vi "Variant_KVP to Strict Variant.vi"(6 "KVP":variant, 7 "use system decimal point (F)":bool, 8 "Strict type matching? (F)":bool, 9 "Default Value Name (empty: label)":string, 10 "Default Value":variant, 11 "Parent Name":string) -> (0 "all found?":bool, 1 "any found?":bool, 2 "Value":variant, 3 "name out":string)   [LabVIEW 2013, in "OpenVariant.lvlib"]
doc: "***********************\nDEPRECATED METHOD KEPT FOR BACKWARD COMPATIBILITY.\nUse the \"Variant_KVP to Strict variant (Standard).vi\" method instead for future development.\n***********************\nThis VI takes a default value as the input and replaces it recursively (cluster, array) with values found in key value pair arrays."
uses:
  TypeDescriptor/TypeDescriptor_GetPString.vi
  Variant_EmptyCluster.vi
  Scalar/FinalStringFormatting.vi
  TypeDescriptor/TypeDescriptor_SetName.vi
  <vilib>/Utility/GetType.llb/TD_Create Cluster.vi
  <vilib>/Utility/GetType.llb/TD_Get Array Information.vi
  <vilib>/Utility/GetType.llb/Get Type Code from I16 Array And Pos.vi
  Scalar/Get Decimal Separator.vi
  OpenVariant.lvlib
  TypeDescriptor/OpenDescriptor.lvlib
  Conversions/OpenConvert.lvlib
  Scalar/OpenScalar.lvlib
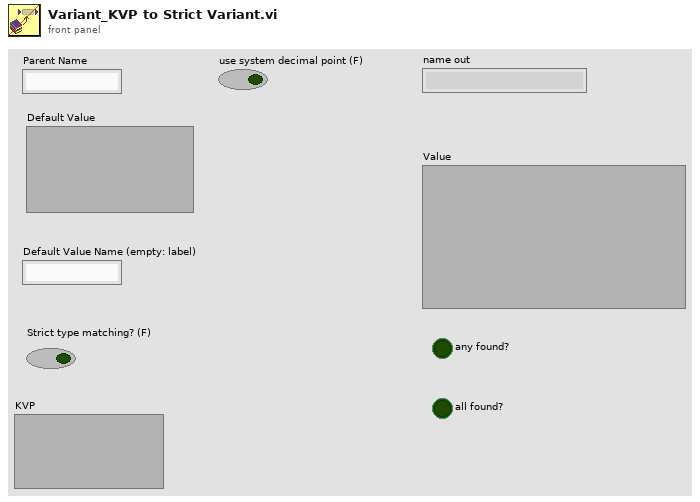
[diagram p1: front panel]
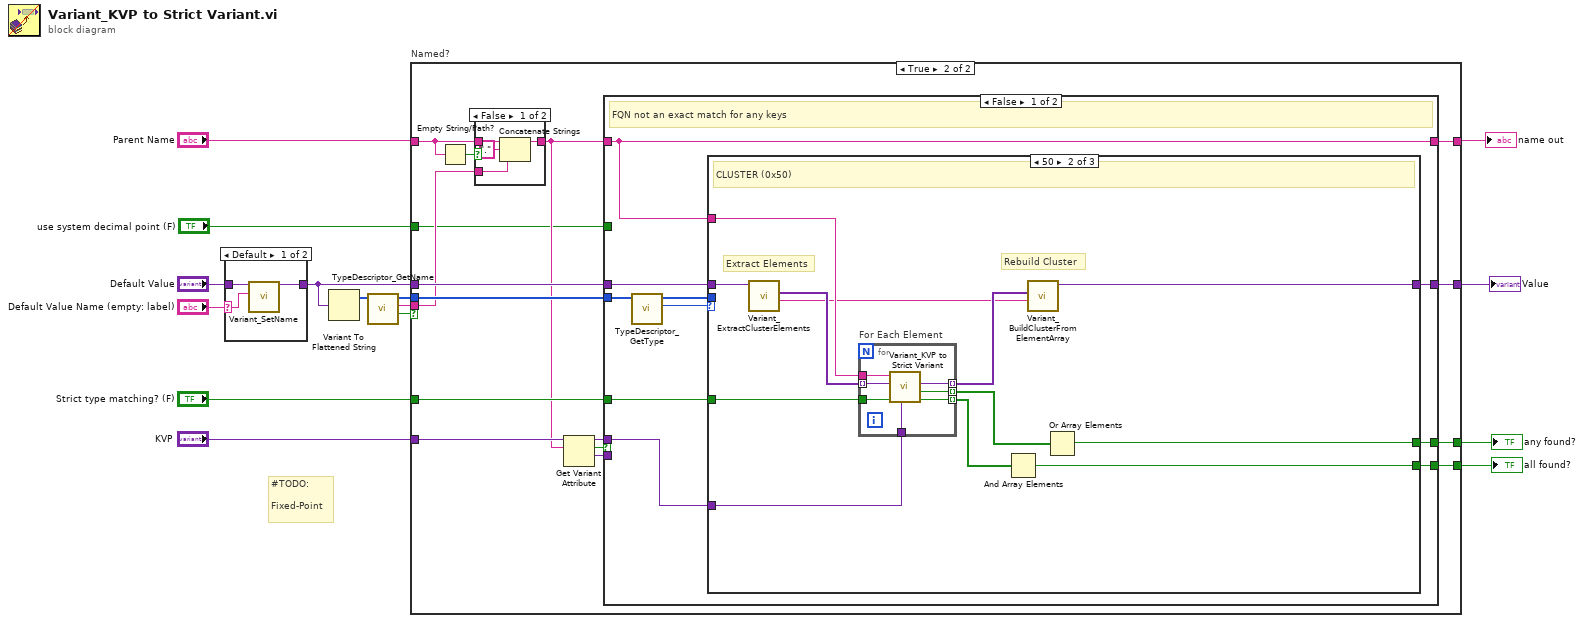
[diagram p0: block diagram]
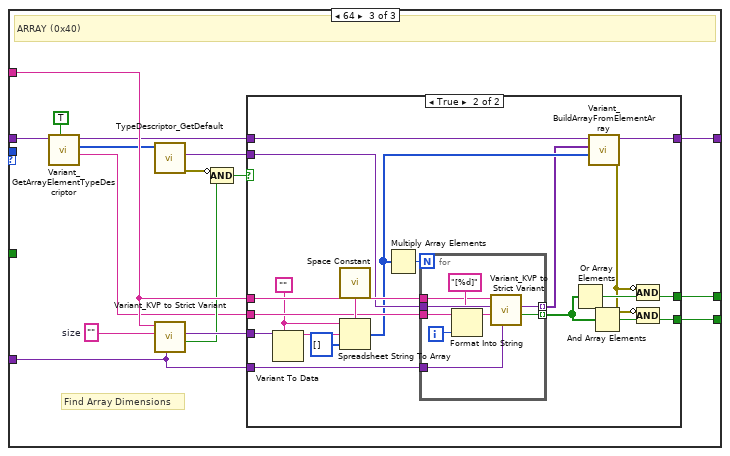
[diagram p6: hidden frame]
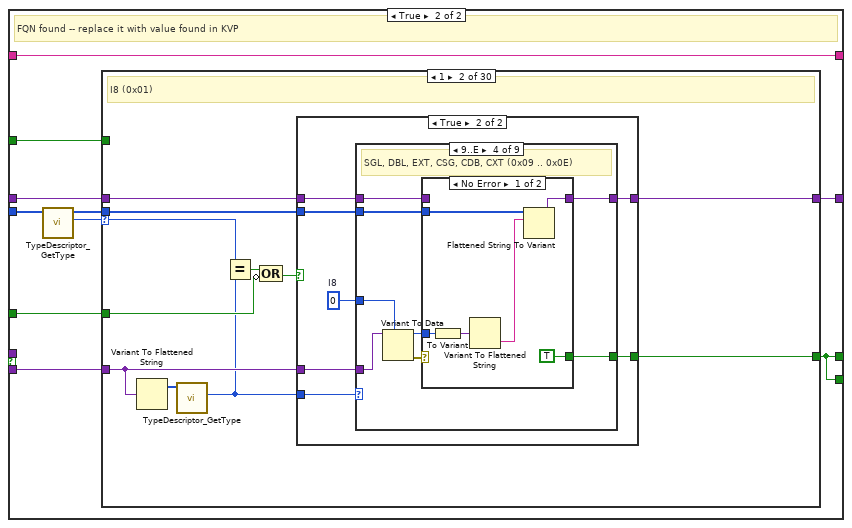
[diagram p8: hidden frame]
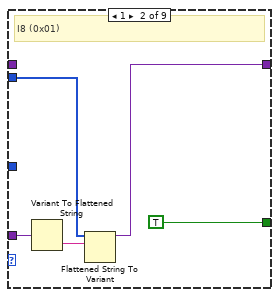
[diagram p12: hidden frame]
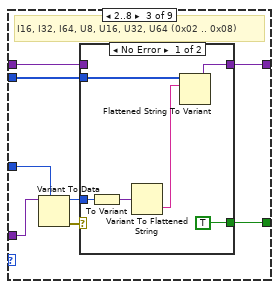
[diagram p13: hidden frame]
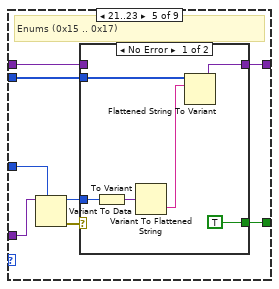
[diagram p16: hidden frame]
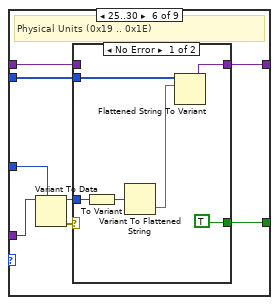
[diagram p18: hidden frame]
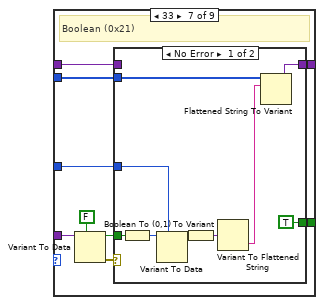
[diagram p20: hidden frame]
diagram:
  # "#TODO: \n\nFixed-Point"
  n1 = case shown="Default" "Default Value Name (empty: label)" {
    selector: "Default Value Name (empty: label)" -> [w17 _]
    tunnel: "Default Value" -> [w18 w19]
    tunnel: [w16 w19] -> w6
    frame Default {
      n2 = call "Variant_SetName.vi"("Name"=w17, "Variant"=w18) -> ("Named Variant"=w16:variant)  [unwired: 9 in]
    }
    frame "" {
    }
  }
  n3 = Variant To Flattened String(Variant=w6) -> (1:w5:i16[])  [unwired: 1 out]
  n4 = call "TypeDescriptor_GetName.vi"("type descriptor"=w5) -> ("found"=w3:bool, "name"=w4:string, "type descriptor dup"=w15:i16[])  [unwired: 8 in]
  n5 = case "Named?" shown="True" w3 {
    tunnel: [w21 w37] -> w13
    tunnel: w6 -> [w21 w36]
    tunnel: w15 -> [_ w32]
    tunnel: w4 -> [_ w28]
    tunnel: "Parent Name" -> [w20 w33]
    tunnel: [w20 w35] -> w14
    tunnel: "Strict type matching? (F)" -> [_ w31]
    tunnel: [_ w30] -> w10
    tunnel: [_ w29] -> w9
    tunnel: "KVP" -> [_ w27]
    tunnel: "use system decimal point (F)" -> [_ w22]
    frame False {
      # "No Name Found -- no value to replace"
    }
    frame True {
      # "Has Name?"
      n6 = Empty String/Path?(string/path=w33) -> (empty?=w34:bool)
      n7 = case shown="False" w34 {
        tunnel: w28 -> [w39 w42]
        tunnel: [w40 w42] -> w24
        tunnel: w33 -> [w41 _]
        frame False {
          n8 = Concatenate Strings(w41, "." ("string"), w39) -> (w40:string)
        }
        frame True {
        }
      }
      n9 = Get Variant Attribute(Variant=w27, name=w24) -> (duplicate Variant=w26:variant, found=w23:bool, value=w25:variant)  [unwired: 2 in, 1 out]
      n10 = case shown="False" w23 {
        tunnel: [w51 w128] -> w37
        tunnel: w36 -> [w50 w127]
        tunnel: w32 -> [w52 w126]
        tunnel: w24 -> [w48 w123]
        tunnel: [w48 w123] -> w35
        tunnel: w31 -> [w47 w122]
        tunnel: [w46 w121] -> w30
        tunnel: [w45 w121] -> w29
        tunnel: w26 -> [w43 _]
        tunnel: w25 -> [_ w120]
        tunnel: w22 -> [_ w119]
        frame False {
          # "FQN not an exact match for any keys"
          n11 = call "TypeDescriptor_GetType.vi"("type descriptor"=w52) -> ("Type"=w49:u8, "type descriptor dup"=w44:i16[])  [unwired: 9 in]
          n12 = case shown="50" w49 {
            tunnel: [w53 w56 w86] -> w51
            tunnel: w50 -> [w53 w65 w76]
            tunnel: w48 -> [_ w64 w83]
            tunnel: w47 -> [_ w63 _]
            tunnel: [_ w61 w88] -> w46
            tunnel: [_ w59 w87] -> w45
            tunnel: w44 -> [_ _ _]
            tunnel: w43 -> [_ w54 w73]
            frame Default {
              # "No Match"
            }
            frame 80 {
              # "Rebuild Cluster"
              # "Extract Elements"
              # "CLUSTER (0x50)"
              n13 = call "Variant_ExtractClusterElements.vi"("Cluster"=w65) -> ("name"=w55:string, "Elements"=w57:variant[])  [unwired: 8 in, 1 out]
              n14 = for "For Each Element" {
                tunnel: [w72] -> w58 mode=indexing
                tunnel: w54 -> [w71]
                tunnel: w57 -> [w70] mode=indexing
                tunnel: w64 -> [w69]
                tunnel: [w68] -> w62 mode=indexing
                tunnel: [w67] -> w60 mode=indexing
                tunnel: w63 -> [w66]
                n15 = call "Variant_KVP to Strict Variant.vi"("KVP"=w71, "Strict type matching? (F)"=w66, "Default Value"=w70, "Parent Name"=w69) -> ("all found?"=w68:bool, "any found?"=w67:bool, "Value"=w72:variant)  [unwired: 4 in, 1 out]
              }
              n16 = And Array Elements(Boolean array=w62) -> (logical AND=w61:bool)
              n17 = call "Variant_BuildClusterFromElementArray.vi"("name"=w55, "Elements"=w58) -> ("Cluster"=w56:variant)  [unwired: 9 in]
              n18 = Or Array Elements(Boolean array=w60) -> (logical OR=w59:bool)
            }
            frame 64 {
              w84 = ""  # size
              # "Find Array Dimensions"
              # "ARRAY (0x40)"
              n19 = call "Variant_GetArrayElementTypeDescriptor.vi"("Name Element if empty string (F)"=TRUE, "Array"=w76) -> ("Element Name"=w78:string, "Element Descriptor"=w77:i16[], "Array dup"=w75:variant)  [unwired: 7 in]
              n20 = call "TypeDescriptor_GetDefault.vi"("type descriptor"=w77) -> ("error out"=w74:errorcluster, "Default"=w81:variant)  [unwired: 8 in, 1 out]
              n21 = call "Variant_KVP to Strict Variant.vi"("KVP"=w73, "Default Value"=w84, "Parent Name"=w83) -> ("any found?"=w80:bool, "Value"=w85:variant)  [unwired: 5 in, 2 out]
              n22 = Compound Arithmetic op=AND(invert w74, w80) -> (w79:bool)
              n23 = case shown="True" w79 {
                tunnel: [_ w93] -> w88
                tunnel: [_ w96] -> w87
                tunnel: [w89 w98] -> w86
                tunnel: w73 -> [_ w105]
                tunnel: w85 -> [_ w104]
                tunnel: w83 -> [_ w102]
                tunnel: w78 -> [_ w101]
                tunnel: w75 -> [w89 w99]
                tunnel: w81 -> [_ w92]
                frame False {
                  # "No Array Dimensions Found in the key value pairs"
                }
                frame True {
                  w100 = "" ("format string")
                  n24 = Variant To Data(type=w100, Variant=w104) -> (data=w103:string)  [unwired: 1 in, 1 out]
                  n25 = call <vilib>:"Space Constant.vi"() -> ("String"=w106:string)
                  n26 = Spreadsheet String To Array(delimiter (Tab)=w106, format string=w100, spreadsheet string=w103, array type (2D Dbl)=u32[] [] ("Dimensions")) -> (array=w91:u32[])
                  n27 = Multiply Array Elements(1:w91) -> (0:w109:u32)
                  n28 = for {
                    N: w109 -> [_]
                    tunnel: w92 -> [w118]
                    tunnel: w105 -> [w115]
                    tunnel: w102 -> [w114]
                    tunnel: [w113] -> w108 mode=indexing
                    tunnel: w101 -> [w112]
                    tunnel: [w110] -> w90 mode=indexing
                    i -> [w111]
                    n29 = Format Into String(format string="[%d]", initial string=w112, w111) -> (resulting string=w116:string)  [unwired: 1 in, 1 out]
                    n30 = call "Variant_KVP to Strict Variant.vi"("KVP"=w115, "Default Value Name (empty: label)"=w116, "Default Value"=w118, "Parent Name"=w114) -> ("any found?"=w113:bool, "Value"=w110:variant)  [unwired: 4 in, 2 out]
                  }
                  n31 = Or Array Elements(Boolean array=w108) -> (logical OR=w97:bool)
                  n32 = call "Variant_BuildArrayFromElementArray.vi"("Dimensions"=w91, "Elements"=w90, "Default Array"=w99) -> ("error out"=w95:errorcluster, "Output Array"=w98:variant)  [unwired: 7 in]
                  n33 = And Array Elements(Boolean array=w108) -> (logical AND=w94:bool)
                  n34 = Compound Arithmetic op=AND(invert w95, w97) -> (w96:bool)
                  n35 = Compound Arithmetic op=AND(invert w95, w94) -> (w93:bool)
                }
              }
            }
          }
        }
        frame True {
          # "FQN found -- replace it with value found in KVP"
          n36 = call "TypeDescriptor_GetType.vi"("type descriptor"=w126) -> ("Type"=w124:u8, "type descriptor dup"=w125:i16[])  [unwired: 9 in]
          n37 = case shown="1" w124 {
            selector: w124 -> [_ w131 w263 w393 w525 w656 w787 w918 w1049 w1180 w1270 w1360 w1449 w1535 w1620 w1706 w1811 w1915 w2017 w2089 w2158 w2229 w2299 w2368 w2438 w2497 w2805 w2863 _ w2903]
            tunnel: w120 -> [_ w136 w267 w398 w529 w660 w791 w922 w1053 w1185 w1275 w1364 w1453 w1540 w1625 w1711 w1816 w1920 w2023 w2093 w2163 w2233 w2303 w2373 w2443 w2503 w2814 w2854 _ w2917]
            tunnel: [w129 w138 w269 w400 w531 w662 w793 w924 w1055 w1187 w1277 w1366 w1455 w1542 w1627 w1713 w1818 w1922 w2025 w2095 w2165 w2235 w2305 w2375 w2445 w2506 w2810 w2866 w2890 w2913] -> w128
            tunnel: w127 -> [w129 w139 w270 w401 w532 w663 w794 w925 w1056 w1188 w1278 w1367 w1456 w1538 w1628 w1714 w1819 w1923 w2026 w2096 w2166 w2236 w2306 w2376 w2446 w2507 w2811 w2867 w2892 w2914]
            tunnel: w125 -> [_ w137 w268 w399 w530 w661 w792 w923 w1054 w1186 w1276 w1365 w1454 w1541 w1626 w1712 w1817 w1921 w2024 w2094 w2164 w2234 w2304 w2374 w2444 w2505 w2809 w2853 _ w2910]
            tunnel: [_ w135 w266 w397 w528 w659 w790 w921 w1052 w1184 w1274 w1363 w1452 w1539 w1624 w1710 w1815 w1919 w2022 w2092 w2162 w2232 w2302 w2372 w2442 w2500 w2807 w2865 w2891 w2908] -> w121
            tunnel: w122 -> [_ w132 w261 w394 w523 w654 w786 w916 w1048 w1181 w1271 w1358 w1447 w1534 w1621 w1707 w1812 w1916 w2019 w2087 w2159 w2228 w2297 w2369 w2439 w2495 w2803 w2856 w2889 w2905]
            tunnel: w119 -> [_ _ _ _ _ _ _ _ _ w1178 w1268 w1357 _ _ _ _ _ _ _ _ _ _ _ _ _ w2494 _ _ _ _]
            frame Default {
            }
            frame 1 {
              # "I8 (0x01)"
              n38 = Variant To Flattened String(Variant=w136) -> (1:w140:i16[])  [unwired: 1 out]
              n39 = call "TypeDescriptor_GetType.vi"("type descriptor"=w140) -> ("Type"=w130:u8)  [unwired: 9 in, 1 out]
              n40 = Equal?(x=w131, y=w130) -> (x = y?=w134:bool)
              n41 = Compound Arithmetic op=OR(w134, invert w132) -> (w133:bool)
              n42 = case shown="True" w133 {
                tunnel: w139 -> [w141 w148]
                tunnel: [w141 w147] -> w138
                tunnel: w137 -> [_ w146]
                tunnel: w130 -> [_ w145]
                tunnel: w136 -> [_ w143]
                tunnel: [_ w142] -> w135
                frame False {
                }
                frame True {
                  w144 = i8 0  # I8
                  n43 = case shown="9..E" w145 {
                    tunnel: w148 -> [w149 _ w159 w174 w189 w204 w216 w238 _]
                    tunnel: [w149 w151 w161 w176 w191 w206 w222 w240 w259] -> w147
                    tunnel: w146 -> [_ w152 w162 w177 w192 w207 w223 w242 w260]
                    tunnel: w144 -> [_ _ w157 w172 w187 w202 w217 w236 w258]
                    tunnel: w143 -> [_ w154 w156 w171 w186 w201 w221 w235 w254]
                    tunnel: [_ TRUE w155 w170 w185 w200 w215 w234 TRUE] -> w142
                    frame Default {
                      # "INCOMPATIBLE DATATYPES"
                    }
                    frame 1 {
                      # "I8 (0x01)"
                      n44 = Variant To Flattened String(Variant=w154) -> (data string=w153:string)  [unwired: 1 out]
                      n45 = Flattened String To Variant(6:w153, 7:w152) -> (3:w151:variant)  [unwired: 1 in, 1 out]
                    }
                    frame 2..8 {
                      # "I16, I32, I64, U8, U16, U32, U64 (0x02 .. 0x08)"
                      n46 = Variant To Data(type=w157, Variant=w156) -> (data=w158:i8, error out=w160:errorcluster)  [unwired: 1 in]
                      n47 = case shown="No Error" w160 {
                        tunnel: w162 -> [w168 _]
                        tunnel: [w167 w169] -> w161
                        tunnel: w159 -> [_ w169]
                        tunnel: w158 -> [w165 _]
                        tunnel: [TRUE _] -> w155
                        frame No Error {
                          n48 = To Variant(anything=w165) -> (Variant=w164:variant)
                          n49 = Variant To Flattened String(Variant=w164) -> (data string=w166:string)  [unwired: 1 out]
                          n50 = Flattened String To Variant(6:w166, 7:w168) -> (3:w167:variant)  [unwired: 1 in, 1 out]
                        }
                        frame Error {
                        }
                      }
                    }
                    frame 9..14 {
                      # "SGL, DBL, EXT, CSG, CDB, CXT (0x09 .. 0x0E)"
                      n51 = Variant To Data(type=w172, Variant=w171) -> (data=w173:i8, error out=w175:errorcluster)  [unwired: 1 in]
                      n52 = case shown="No Error" w175 {
                        tunnel: w177 -> [w183 _]
                        tunnel: [w182 w184] -> w176
                        tunnel: w174 -> [_ w184]
                        tunnel: w173 -> [w180 _]
                        tunnel: [TRUE _] -> w170
                        frame No Error {
                          n53 = To Variant(anything=w180) -> (Variant=w179:variant)
                          n54 = Variant To Flattened String(Variant=w179) -> (data string=w181:string)  [unwired: 1 out]
                          n55 = Flattened String To Variant(6:w181, 7:w183) -> (3:w182:variant)  [unwired: 1 in, 1 out]
                        }
                        frame Error {
                        }
                      }
                    }
                    frame 21..23 {
                      # "Enums (0x15 .. 0x17)"
                      n56 = Variant To Data(type=w187, Variant=w186) -> (data=w188:i8, error out=w190:errorcluster)  [unwired: 1 in]
                      n57 = case shown="No Error" w190 {
                        tunnel: w192 -> [w198 _]
                        tunnel: [w197 w199] -> w191
                        tunnel: w189 -> [_ w199]
                        tunnel: w188 -> [w195 _]
                        tunnel: [TRUE _] -> w185
                        frame No Error {
                          n58 = To Variant(anything=w195) -> (Variant=w194:variant)
                          n59 = Variant To Flattened String(Variant=w194) -> (data string=w196:string)  [unwired: 1 out]
                          n60 = Flattened String To Variant(6:w196, 7:w198) -> (3:w197:variant)  [unwired: 1 in, 1 out]
                        }
                        frame Error {
                        }
                      }
                    }
                    frame 25..30 {
                      # "Physical Units (0x19 .. 0x1E)"
                      n61 = Variant To Data(type=w202, Variant=w201) -> (data=w203:i8, error out=w205:errorcluster)  [unwired: 1 in]
                      n62 = case shown="No Error" w205 {
                        tunnel: w207 -> [w213 _]
                        tunnel: [w212 w214] -> w206
                        tunnel: w204 -> [_ w214]
                        tunnel: w203 -> [w210 _]
                        tunnel: [TRUE _] -> w200
                        frame No Error {
                          n63 = To Variant(anything=w210) -> (Variant=w209:variant)
                          n64 = Variant To Flattened String(Variant=w209) -> (data string=w211:string)  [unwired: 1 out]
                          n65 = Flattened String To Variant(6:w211, 7:w213) -> (3:w212:variant)  [unwired: 1 in, 1 out]
                        }
                        frame Error {
                        }
                      }
                    }
                    frame 33 {
                      # "Boolean (0x21)"
                      n66 = Variant To Data(type=FALSE, Variant=w221) -> (data=w218:bool, error out=w219:errorcluster)  [unwired: 1 in]
                      n67 = case shown="No Error" w219 {
                        tunnel: w223 -> [w232 _]
                        tunnel: [w231 w233] -> w222
                        tunnel: w218 -> [w228 _]
                        tunnel: w217 -> [w226 _]
                        tunnel: w216 -> [_ w233]
                        tunnel: [TRUE _] -> w215
                        frame No Error {
                          n68 = Boolean To (0,1)(Boolean=w228) -> (0, 1=w227:i16)
                          n69 = Variant To Data(type=w226, Variant=w227) -> (data=w225:i8)  [unwired: 1 in, 1 out]
                          n70 = To Variant(anything=w225) -> (Variant=w229:variant)
                          n71 = Variant To Flattened String(Variant=w229) -> (data string=w230:string)  [unwired: 1 out]
                          n72 = Flattened String To Variant(6:w230, 7:w232) -> (3:w231:variant)  [unwired: 1 in, 1 out]
                        }
                        frame Error {
                        }
                      }
                    }
                    frame 48 {
                      # "STRING (0x30)"
                      n73 = Variant To Data(type="", Variant=w235) -> (data=w237:string, error out=w239:errorcluster)  [unwired: 1 in]
                      n74 = case shown="No Error" w239 {
                        tunnel: w242 -> [w250 _]
                        tunnel: [w249 w251] -> w240
                        tunnel: w238 -> [_ w251]
                        tunnel: w237 -> [w246 _]
                        tunnel: w236 -> [w244 _]
                        tunnel: [TRUE _] -> w234
                        frame No Error {
                          n75 = Fract/Exp String To Number(string=w246, default (0 dbl)=w244) -> (number=w245:i8)  [unwired: 2 in, 1 out]
                          n76 = To Variant(anything=w245) -> (Variant=w248:variant)
                          n77 = Variant To Flattened String(Variant=w248) -> (data string=w247:string)  [unwired: 1 out]
                          n78 = Flattened String To Variant(6:w247, 7:w250) -> (3:w249:variant)  [unwired: 1 in, 1 out]
                        }
                        frame Error {
                        }
                      }
                    }
                    frame 112 {
                      # "Refnum (0x70)"
                      n79 = Variant To Flattened String(Variant=w254) -> (data string=w253:string)  [unwired: 1 out]
                      n80 = Type Cast(type=w258, x=w253) -> (*(type *) &x=w257:i8)
                      n81 = To Variant(anything=w257) -> (Variant=w256:variant)
                      n82 = Variant To Flattened String(Variant=w256) -> (data string=w255:string)  [unwired: 1 out]
                      n83 = Flattened String To Variant(6:w255, 7:w260) -> (3:w259:variant)  [unwired: 1 in, 1 out]
                    }
                  }
                }
              }
            }
            frame 2 {
              # "I16 (0x02)"
              n84 = Variant To Flattened String(Variant=w267) -> (1:w271:i16[])  [unwired: 1 out]
              n85 = call "TypeDescriptor_GetType.vi"("type descriptor"=w271) -> ("Type"=w262:u8)  [unwired: 9 in, 1 out]
              n86 = Equal?(x=w263, y=w262) -> (x = y?=w265:bool)
              n87 = Compound Arithmetic op=OR(w265, invert w261) -> (w264:bool)
              n88 = case shown="True" w264 {
                tunnel: w270 -> [w272 w279]
                tunnel: [w272 w278] -> w269
                tunnel: w268 -> [_ w277]
                tunnel: w262 -> [_ w276]
                tunnel: w267 -> [_ w274]
                tunnel: [_ w273] -> w266
                frame False {
                }
                frame True {
                  w275 = i16 0  # I16
                  n89 = case shown="2" w276 {
                    tunnel: w279 -> [w280 _ w290 w305 w320 w335 w347 w369 _]
                    tunnel: [w280 w282 w292 w307 w322 w337 w353 w371 w390] -> w278
                    tunnel: w277 -> [_ w283 w293 w308 w323 w338 w354 w373 w391]
                    tunnel: w275 -> [_ _ w288 w303 w318 w333 w348 w367 w389]
                    tunnel: w274 -> [_ w285 w287 w302 w317 w332 w352 w366 w385]
                    tunnel: [_ TRUE w286 w301 w316 w331 w346 w365 TRUE] -> w273
                    frame Default {
                      # "INCOMPATIBLE DATATYPES"
                    }
                    frame 2 {
                      # "I16 (0x02)"
                      n90 = Variant To Flattened String(Variant=w285) -> (data string=w284:string)  [unwired: 1 out]
                      n91 = Flattened String To Variant(6:w284, 7:w283) -> (3:w282:variant)  [unwired: 1 in, 1 out]
                    }
                    frame 1, 3..8 {
                      # "I8, I32, I64, U8, U16, U32, U64 (0x02 .. 0x08)"
                      n92 = Variant To Data(type=w288, Variant=w287) -> (data=w289:i16, error out=w291:errorcluster)  [unwired: 1 in]
                      n93 = case shown="No Error" w291 {
                        tunnel: w293 -> [w299 _]
                        tunnel: [w298 w300] -> w292
                        tunnel: w290 -> [_ w300]
                        tunnel: w289 -> [w296 _]
                        tunnel: [TRUE _] -> w286
                        frame No Error {
                          n94 = To Variant(anything=w296) -> (Variant=w295:variant)
                          n95 = Variant To Flattened String(Variant=w295) -> (data string=w297:string)  [unwired: 1 out]
                          n96 = Flattened String To Variant(6:w297, 7:w299) -> (3:w298:variant)  [unwired: 1 in, 1 out]
                        }
                        frame Error {
                        }
                      }
                    }
                    frame 9..14 {
                      # "SGL, DBL, EXT, CSG, CDB, CXT (0x09 .. 0x0E)"
                      n97 = Variant To Data(type=w303, Variant=w302) -> (data=w304:i16, error out=w306:errorcluster)  [unwired: 1 in]
                      n98 = case shown="No Error" w306 {
                        tunnel: w308 -> [w314 _]
                        tunnel: [w313 w315] -> w307
                        tunnel: w305 -> [_ w315]
                        tunnel: w304 -> [w311 _]
                        tunnel: [TRUE _] -> w301
                        frame No Error {
                          n99 = To Variant(anything=w311) -> (Variant=w310:variant)
                          n100 = Variant To Flattened String(Variant=w310) -> (data string=w312:string)  [unwired: 1 out]
                          n101 = Flattened String To Variant(6:w312, 7:w314) -> (3:w313:variant)  [unwired: 1 in, 1 out]
                        }
                        frame Error {
                        }
                      }
                    }
                    frame 21..23 {
                      # "Enums (0x15 .. 0x17)"
                      n102 = Variant To Data(type=w318, Variant=w317) -> (data=w319:i16, error out=w321:errorcluster)  [unwired: 1 in]
                      n103 = case shown="No Error" w321 {
                        tunnel: w323 -> [w329 _]
                        tunnel: [w328 w330] -> w322
                        tunnel: w320 -> [_ w330]
                        tunnel: w319 -> [w326 _]
                        tunnel: [TRUE _] -> w316
                        frame No Error {
                          n104 = To Variant(anything=w326) -> (Variant=w325:variant)
                          n105 = Variant To Flattened String(Variant=w325) -> (data string=w327:string)  [unwired: 1 out]
                          n106 = Flattened String To Variant(6:w327, 7:w329) -> (3:w328:variant)  [unwired: 1 in, 1 out]
                        }
                        frame Error {
                        }
                      }
                    }
                    frame 25..30 {
                      # "Physical Units (0x19 .. 0x1E)"
                      n107 = Variant To Data(type=w333, Variant=w332) -> (data=w334:i16, error out=w336:errorcluster)  [unwired: 1 in]
                      n108 = case shown="No Error" w336 {
                        tunnel: w338 -> [w344 _]
                        tunnel: [w343 w345] -> w337
                        tunnel: w335 -> [_ w345]
                        tunnel: w334 -> [w341 _]
                        tunnel: [TRUE _] -> w331
                        frame No Error {
                          n109 = To Variant(anything=w341) -> (Variant=w340:variant)
                          n110 = Variant To Flattened String(Variant=w340) -> (data string=w342:string)  [unwired: 1 out]
                          n111 = Flattened String To Variant(6:w342, 7:w344) -> (3:w343:variant)  [unwired: 1 in, 1 out]
                        }
                        frame Error {
                        }
                      }
                    }
                    frame 33 {
                      # "Boolean (0x21)"
                      n112 = Variant To Data(type=FALSE, Variant=w352) -> (data=w349:bool, error out=w350:errorcluster)  [unwired: 1 in]
                      n113 = case shown="No Error" w350 {
                        tunnel: w354 -> [w363 _]
                        tunnel: [w362 w364] -> w353
                        tunnel: w349 -> [w359 _]
                        tunnel: w348 -> [w357 _]
                        tunnel: w347 -> [_ w364]
                        tunnel: [TRUE _] -> w346
                        frame No Error {
                          n114 = Boolean To (0,1)(Boolean=w359) -> (0, 1=w358:i16)
                          n115 = Variant To Data(type=w357, Variant=w358) -> (data=w356:i16)  [unwired: 1 in, 1 out]
                          n116 = To Variant(anything=w356) -> (Variant=w360:variant)
                          n117 = Variant To Flattened String(Variant=w360) -> (data string=w361:string)  [unwired: 1 out]
                          n118 = Flattened String To Variant(6:w361, 7:w363) -> (3:w362:variant)  [unwired: 1 in, 1 out]
                        }
                        frame Error {
                        }
                      }
                    }
                    frame 48 {
                      # "STRING (0x30)"
                      n119 = Variant To Data(type="", Variant=w366) -> (data=w368:string, error out=w370:errorcluster)  [unwired: 1 in]
                      n120 = case shown="No Error" w370 {
                        tunnel: w373 -> [w381 _]
                        tunnel: [w380 w382] -> w371
                        tunnel: w369 -> [_ w382]
                        tunnel: w368 -> [w377 _]
                        tunnel: w367 -> [w375 _]
                        tunnel: [TRUE _] -> w365
                        frame No Error {
                          n121 = Fract/Exp String To Number(string=w377, default (0 dbl)=w375) -> (number=w376:i16)  [unwired: 2 in, 1 out]
                          n122 = To Variant(anything=w376) -> (Variant=w379:variant)
                          n123 = Variant To Flattened String(Variant=w379) -> (data string=w378:string)  [unwired: 1 out]
                          n124 = Flattened String To Variant(6:w378, 7:w381) -> (3:w380:variant)  [unwired: 1 in, 1 out]
                        }
                        frame Error {
                        }
                      }
                    }
                    frame 112 {
                      # "Refnum (0x70)"
                      n125 = Variant To Flattened String(Variant=w385) -> (data string=w384:string)  [unwired: 1 out]
                      n126 = Type Cast(type=w389, x=w384) -> (*(type *) &x=w388:i16)
                      n127 = To Variant(anything=w388) -> (Variant=w387:variant)
                      n128 = Variant To Flattened String(Variant=w387) -> (data string=w386:string)  [unwired: 1 out]
                      n129 = Flattened String To Variant(6:w386, 7:w391) -> (3:w390:variant)  [unwired: 1 in, 1 out]
                    }
                  }
                }
              }
            }
            frame 3 {
              # "I32 (0x03)"
              n130 = Variant To Flattened String(Variant=w398) -> (1:w402:i16[])  [unwired: 1 out]
              n131 = call "TypeDescriptor_GetType.vi"("type descriptor"=w402) -> ("Type"=w392:u8)  [unwired: 9 in, 1 out]
              n132 = Equal?(x=w393, y=w392) -> (x = y?=w396:bool)
              n133 = Compound Arithmetic op=OR(w396, invert w394) -> (w395:bool)
              n134 = case shown="True" w395 {
                tunnel: w401 -> [w403 w410]
                tunnel: [w403 w409] -> w400
                tunnel: w399 -> [_ w408]
                tunnel: w392 -> [_ w407]
                tunnel: w398 -> [_ w405]
                tunnel: [_ w404] -> w397
                frame False {
                }
                frame True {
                  w406 = 0  # I32
                  n135 = case shown="21" w407 {
                    tunnel: w410 -> [w411 _ w421 w436 w451 w466 w478 w500 _]
                    tunnel: [w411 w413 w423 w438 w453 w468 w484 w502 w521] -> w409
                    tunnel: w408 -> [_ w414 w424 w439 w454 w469 w485 w504 w522]
                    tunnel: w406 -> [_ _ w419 w434 w449 w464 w479 w498 w520]
                    tunnel: w405 -> [_ w416 w418 w433 w448 w463 w483 w497 w516]
                    tunnel: [_ TRUE w417 w432 w447 w462 w477 w496 TRUE] -> w404
                    frame Default {
                      # "INCOMPATIBLE DATATYPES"
                    }
                    frame 3 {
                      # "I32 (0x03)"
                      n136 = Variant To Flattened String(Variant=w416) -> (data string=w415:string)  [unwired: 1 out]
                      n137 = Flattened String To Variant(6:w415, 7:w414) -> (3:w413:variant)  [unwired: 1 in, 1 out]
                    }
                    frame 1, 2, 4..8 {
                      # "I8, I16, I64, U8, U16, U32, U64 (0x02 .. 0x08)"
                      n138 = Variant To Data(type=w419, Variant=w418) -> (data=w420:i32, error out=w422:errorcluster)  [unwired: 1 in]
                      n139 = case shown="No Error" w422 {
                        tunnel: w424 -> [w430 _]
                        tunnel: [w429 w431] -> w423
                        tunnel: w421 -> [_ w431]
                        tunnel: w420 -> [w427 _]
                        tunnel: [TRUE _] -> w417
                        frame No Error {
                          n140 = To Variant(anything=w427) -> (Variant=w426:variant)
                          n141 = Variant To Flattened String(Variant=w426) -> (data string=w428:string)  [unwired: 1 out]
                          n142 = Flattened String To Variant(6:w428, 7:w430) -> (3:w429:variant)  [unwired: 1 in, 1 out]
                        }
                        frame Error {
                        }
                      }
                    }
                    frame 9..14 {
                      # "SGL, DBL, EXT, CSG, CDB, CXT (0x09 .. 0x0E)"
                      n143 = Variant To Data(type=w434, Variant=w433) -> (data=w435:i32, error out=w437:errorcluster)  [unwired: 1 in]
                      n144 = case shown="No Error" w437 {
                        tunnel: w439 -> [w445 _]
                        tunnel: [w444 w446] -> w438
                        tunnel: w436 -> [_ w446]
                        tunnel: w435 -> [w442 _]
                        tunnel: [TRUE _] -> w432
                        frame No Error {
                          n145 = To Variant(anything=w442) -> (Variant=w441:variant)
                          n146 = Variant To Flattened String(Variant=w441) -> (data string=w443:string)  [unwired: 1 out]
                          n147 = Flattened String To Variant(6:w443, 7:w445) -> (3:w444:variant)  [unwired: 1 in, 1 out]
                        }
                        frame Error {
                        }
                      }
                    }
                    frame 21..23 {
                      # "Enums (0x15 .. 0x17)"
                      n148 = Variant To Data(type=w449, Variant=w448) -> (data=w450:i32, error out=w452:errorcluster)  [unwired: 1 in]
                      n149 = case shown="No Error" w452 {
                        tunnel: w454 -> [w460 _]
                        tunnel: [w459 w461] -> w453
                        tunnel: w451 -> [_ w461]
                        tunnel: w450 -> [w457 _]
                        tunnel: [TRUE _] -> w447
                        frame No Error {
                          n150 = To Variant(anything=w457) -> (Variant=w456:variant)
                          n151 = Variant To Flattened String(Variant=w456) -> (data string=w458:string)  [unwired: 1 out]
                          n152 = Flattened String To Variant(6:w458, 7:w460) -> (3:w459:variant)  [unwired: 1 in, 1 out]
                        }
                        frame Error {
                        }
                      }
                    }
                    frame 25..30 {
                      # "Physical Units (0x19 .. 0x1E)"
                      n153 = Variant To Data(type=w464, Variant=w463) -> (data=w465:i32, error out=w467:errorcluster)  [unwired: 1 in]
                      n154 = case shown="No Error" w467 {
                        tunnel: w469 -> [w475 _]
                        tunnel: [w474 w476] -> w468
                        tunnel: w466 -> [_ w476]
                        tunnel: w465 -> [w472 _]
                        tunnel: [TRUE _] -> w462
                        frame No Error {
                          n155 = To Variant(anything=w472) -> (Variant=w471:variant)
                          n156 = Variant To Flattened String(Variant=w471) -> (data string=w473:string)  [unwired: 1 out]
                          n157 = Flattened String To Variant(6:w473, 7:w475) -> (3:w474:variant)  [unwired: 1 in, 1 out]
                        }
                        frame Error {
                        }
                      }
                    }
                    frame 33 {
                      # "Boolean (0x21)"
                      n158 = Variant To Data(type=FALSE, Variant=w483) -> (data=w480:bool, error out=w481:errorcluster)  [unwired: 1 in]
                      n159 = case shown="No Error" w481 {
                        tunnel: w485 -> [w494 _]
                        tunnel: [w493 w495] -> w484
                        tunnel: w480 -> [w490 _]
                        tunnel: w479 -> [w488 _]
                        tunnel: w478 -> [_ w495]
                        tunnel: [TRUE _] -> w477
                        frame No Error {
                          n160 = Boolean To (0,1)(Boolean=w490) -> (0, 1=w489:i16)
                          n161 = Variant To Data(type=w488, Variant=w489) -> (data=w487:i32)  [unwired: 1 in, 1 out]
                          n162 = To Variant(anything=w487) -> (Variant=w491:variant)
                          n163 = Variant To Flattened String(Variant=w491) -> (data string=w492:string)  [unwired: 1 out]
                          n164 = Flattened String To Variant(6:w492, 7:w494) -> (3:w493:variant)  [unwired: 1 in, 1 out]
                        }
                        frame Error {
                        }
                      }
                    }
                    frame 48 {
                      # "STRING (0x30)"
                      n165 = Variant To Data(type="", Variant=w497) -> (data=w499:string, error out=w501:errorcluster)  [unwired: 1 in]
                      n166 = case shown="No Error" w501 {
                        tunnel: w504 -> [w512 _]
                        tunnel: [w511 w513] -> w502
                        tunnel: w500 -> [_ w513]
                        tunnel: w499 -> [w508 _]
                        tunnel: w498 -> [w506 _]
                        tunnel: [TRUE _] -> w496
                        frame No Error {
                          n167 = Fract/Exp String To Number(string=w508, default (0 dbl)=w506) -> (number=w507:i32)  [unwired: 2 in, 1 out]
                          n168 = To Variant(anything=w507) -> (Variant=w510:variant)
                          n169 = Variant To Flattened String(Variant=w510) -> (data string=w509:string)  [unwired: 1 out]
                          n170 = Flattened String To Variant(6:w509, 7:w512) -> (3:w511:variant)  [unwired: 1 in, 1 out]
                        }
                        frame Error {
                        }
                      }
                    }
                    frame 112 {
                      # "Refnum (0x70)"
                      n171 = Variant To Flattened String(Variant=w516) -> (data string=w515:string)  [unwired: 1 out]
                      n172 = Type Cast(type=w520, x=w515) -> (*(type *) &x=w519:i32)
                      n173 = To Variant(anything=w519) -> (Variant=w518:variant)
                      n174 = Variant To Flattened String(Variant=w518) -> (data string=w517:string)  [unwired: 1 out]
                      n175 = Flattened String To Variant(6:w517, 7:w522) -> (3:w521:variant)  [unwired: 1 in, 1 out]
                    }
                  }
                }
              }
            }
            frame 4 {
              # "I64 (0x04)"
              n176 = Variant To Flattened String(Variant=w529) -> (1:w533:i16[])  [unwired: 1 out]
              n177 = call "TypeDescriptor_GetType.vi"("type descriptor"=w533) -> ("Type"=w524:u8)  [unwired: 9 in, 1 out]
              n178 = Equal?(x=w525, y=w524) -> (x = y?=w527:bool)
              n179 = Compound Arithmetic op=OR(w527, invert w523) -> (w526:bool)
              n180 = case shown="True" w526 {
                tunnel: w532 -> [w534 w541]
                tunnel: [w534 w540] -> w531
                tunnel: w530 -> [_ w539]
                tunnel: w524 -> [_ w538]
                tunnel: w529 -> [_ w536]
                tunnel: [_ w535] -> w528
                frame False {
                }
                frame True {
                  w537 = i64 0  # I64
                  n181 = case shown="1..3, 5..8" w538 {
                    tunnel: w541 -> [w542 _ w552 w567 w582 w597 w609 w631 _]
                    tunnel: [w542 w544 w554 w569 w584 w599 w615 w633 w652] -> w540
                    tunnel: w539 -> [_ w545 w555 w570 w585 w600 w616 w635 w653]
                    tunnel: w537 -> [_ _ w550 w565 w580 w595 w610 w629 w651]
                    tunnel: w536 -> [_ w547 w549 w564 w579 w594 w614 w628 w647]
                    tunnel: [_ TRUE w548 w563 w578 w593 w608 w627 TRUE] -> w535
                    frame Default {
                      # "INCOMPATIBLE DATATYPES"
                    }
                    frame 4 {
                      # "I64 (0x04)"
                      n182 = Variant To Flattened String(Variant=w547) -> (data string=w546:string)  [unwired: 1 out]
                      n183 = Flattened String To Variant(6:w546, 7:w545) -> (3:w544:variant)  [unwired: 1 in, 1 out]
                    }
                    frame 1..3, 5..8 {
                      # "I8, I16, I32, U8, U16, U32, U64"
                      n184 = Variant To Data(type=w550, Variant=w549) -> (data=w551:i64, error out=w553:errorcluster)  [unwired: 1 in]
                      n185 = case shown="No Error" w553 {
                        tunnel: w555 -> [w561 _]
                        tunnel: [w560 w562] -> w554
                        tunnel: w552 -> [_ w562]
                        tunnel: w551 -> [w558 _]
                        tunnel: [TRUE _] -> w548
                        frame No Error {
                          n186 = To Variant(anything=w558) -> (Variant=w557:variant)
                          n187 = Variant To Flattened String(Variant=w557) -> (data string=w559:string)  [unwired: 1 out]
                          n188 = Flattened String To Variant(6:w559, 7:w561) -> (3:w560:variant)  [unwired: 1 in, 1 out]
                        }
                        frame Error {
                        }
                      }
                    }
                    frame 9..14 {
                      # "SGL, DBL, EXT, CSG, CDB, CXT (0x09 .. 0x0E)"
                      n189 = Variant To Data(type=w565, Variant=w564) -> (data=w566:i64, error out=w568:errorcluster)  [unwired: 1 in]
                      n190 = case shown="No Error" w568 {
                        tunnel: w570 -> [w576 _]
                        tunnel: [w575 w577] -> w569
                        tunnel: w567 -> [_ w577]
                        tunnel: w566 -> [w573 _]
                        tunnel: [TRUE _] -> w563
                        frame No Error {
                          n191 = To Variant(anything=w573) -> (Variant=w572:variant)
                          n192 = Variant To Flattened String(Variant=w572) -> (data string=w574:string)  [unwired: 1 out]
                          n193 = Flattened String To Variant(6:w574, 7:w576) -> (3:w575:variant)  [unwired: 1 in, 1 out]
                        }
                        frame Error {
                        }
                      }
                    }
                    frame 21..23 {
                      # "Enums (0x15 .. 0x17)"
                      n194 = Variant To Data(type=w580, Variant=w579) -> (data=w581:i64, error out=w583:errorcluster)  [unwired: 1 in]
                      n195 = case shown="No Error" w583 {
                        tunnel: w585 -> [w591 _]
                        tunnel: [w590 w592] -> w584
                        tunnel: w582 -> [_ w592]
                        tunnel: w581 -> [w588 _]
                        tunnel: [TRUE _] -> w578
                        frame No Error {
                          n196 = To Variant(anything=w588) -> (Variant=w587:variant)
                          n197 = Variant To Flattened String(Variant=w587) -> (data string=w589:string)  [unwired: 1 out]
                          n198 = Flattened String To Variant(6:w589, 7:w591) -> (3:w590:variant)  [unwired: 1 in, 1 out]
                        }
                        frame Error {
                        }
                      }
                    }
                    frame 25..30 {
                      # "Physical Units (0x19 .. 0x1E)"
                      n199 = Variant To Data(type=w595, Variant=w594) -> (data=w596:i64, error out=w598:errorcluster)  [unwired: 1 in]
                      n200 = case shown="No Error" w598 {
                        tunnel: w600 -> [w606 _]
                        tunnel: [w605 w607] -> w599
                        tunnel: w597 -> [_ w607]
                        tunnel: w596 -> [w603 _]
                        tunnel: [TRUE _] -> w593
                        frame No Error {
                          n201 = To Variant(anything=w603) -> (Variant=w602:variant)
                          n202 = Variant To Flattened String(Variant=w602) -> (data string=w604:string)  [unwired: 1 out]
                          n203 = Flattened String To Variant(6:w604, 7:w606) -> (3:w605:variant)  [unwired: 1 in, 1 out]
                        }
                        frame Error {
                        }
                      }
                    }
                    frame 33 {
                      # "Boolean (0x21)"
                      n204 = Variant To Data(type=FALSE, Variant=w614) -> (data=w611:bool, error out=w612:errorcluster)  [unwired: 1 in]
                      n205 = case shown="No Error" w612 {
                        tunnel: w616 -> [w625 _]
                        tunnel: [w624 w626] -> w615
                        tunnel: w611 -> [w621 _]
                        tunnel: w610 -> [w619 _]
                        tunnel: w609 -> [_ w626]
                        tunnel: [TRUE _] -> w608
                        frame No Error {
                          n206 = Boolean To (0,1)(Boolean=w621) -> (0, 1=w620:i16)
                          n207 = Variant To Data(type=w619, Variant=w620) -> (data=w618:i64)  [unwired: 1 in, 1 out]
                          n208 = To Variant(anything=w618) -> (Variant=w622:variant)
                          n209 = Variant To Flattened String(Variant=w622) -> (data string=w623:string)  [unwired: 1 out]
                          n210 = Flattened String To Variant(6:w623, 7:w625) -> (3:w624:variant)  [unwired: 1 in, 1 out]
                        }
                        frame Error {
                        }
                      }
                    }
                    frame 48 {
                      # "STRING (0x30)"
                      n211 = Variant To Data(type="", Variant=w628) -> (data=w630:string, error out=w632:errorcluster)  [unwired: 1 in]
                      n212 = case shown="No Error" w632 {
                        tunnel: w635 -> [w643 _]
                        tunnel: [w642 w644] -> w633
                        tunnel: w631 -> [_ w644]
                        tunnel: w630 -> [w639 _]
                        tunnel: w629 -> [w637 _]
                        tunnel: [TRUE _] -> w627
                        frame No Error {
                          n213 = Fract/Exp String To Number(string=w639, default (0 dbl)=w637) -> (number=w638:i64)  [unwired: 2 in, 1 out]
                          n214 = To Variant(anything=w638) -> (Variant=w641:variant)
                          n215 = Variant To Flattened String(Variant=w641) -> (data string=w640:string)  [unwired: 1 out]
                          n216 = Flattened String To Variant(6:w640, 7:w643) -> (3:w642:variant)  [unwired: 1 in, 1 out]
                        }
                        frame Error {
                        }
                      }
                    }
                    frame 112 {
                      # "Refnum (0x70)"
                      n217 = Variant To Flattened String(Variant=w647) -> (data string=w646:string)  [unwired: 1 out]
                      n218 = Type Cast(type=w651, x=w646) -> (*(type *) &x=w650:i64)
                      n219 = To Variant(anything=w650) -> (Variant=w649:variant)
                      n220 = Variant To Flattened String(Variant=w649) -> (data string=w648:string)  [unwired: 1 out]
                      n221 = Flattened String To Variant(6:w648, 7:w653) -> (3:w652:variant)  [unwired: 1 in, 1 out]
                    }
                  }
                }
              }
            }
            frame 5 {
              # "U8 (0x05)"
              n222 = Variant To Flattened String(Variant=w660) -> (1:w664:i16[])  [unwired: 1 out]
              n223 = call "TypeDescriptor_GetType.vi"("type descriptor"=w664) -> ("Type"=w655:u8)  [unwired: 9 in, 1 out]
              n224 = Equal?(x=w656, y=w655) -> (x = y?=w658:bool)
              n225 = Compound Arithmetic op=OR(w658, invert w654) -> (w657:bool)
              n226 = case shown="True" w657 {
                tunnel: w663 -> [w665 w672]
                tunnel: [w665 w671] -> w662
                tunnel: w661 -> [_ w670]
                tunnel: w655 -> [_ w669]
                tunnel: w660 -> [_ w667]
                tunnel: [_ w666] -> w659
                frame False {
                }
                frame True {
                  w668 = u8 0  # U8
                  n227 = case shown="1..4, 6..8" w669 {
                    tunnel: w672 -> [w673 _ w683 w698 w713 w728 w740 w762 _]
                    tunnel: [w673 w675 w685 w700 w715 w730 w746 w764 w783] -> w671
                    tunnel: w670 -> [_ w676 w686 w701 w716 w731 w747 w766 w784]
                    tunnel: w668 -> [_ _ w681 w696 w711 w726 w741 w760 w782]
                    tunnel: w667 -> [_ w678 w680 w695 w710 w725 w745 w759 w778]
                    tunnel: [_ TRUE w679 w694 w709 w724 w739 w758 TRUE] -> w666
                    frame Default {
                      # "INCOMPATIBLE DATATYPES"
                    }
                    frame 5 {
                      # "U8 (0x05)"
                      n228 = Variant To Flattened String(Variant=w678) -> (data string=w677:string)  [unwired: 1 out]
                      n229 = Flattened String To Variant(6:w677, 7:w676) -> (3:w675:variant)  [unwired: 1 in, 1 out]
                    }
                    frame 1..4, 6..8 {
                      # "I8, I16, I32, I64, U16, U32, U64"
                      n230 = Variant To Data(type=w681, Variant=w680) -> (data=w682:u8, error out=w684:errorcluster)  [unwired: 1 in]
                      n231 = case shown="No Error" w684 {
                        tunnel: w686 -> [w692 _]
                        tunnel: [w691 w693] -> w685
                        tunnel: w683 -> [_ w693]
                        tunnel: w682 -> [w689 _]
                        tunnel: [TRUE _] -> w679
                        frame No Error {
                          n232 = To Variant(anything=w689) -> (Variant=w688:variant)
                          n233 = Variant To Flattened String(Variant=w688) -> (data string=w690:string)  [unwired: 1 out]
                          n234 = Flattened String To Variant(6:w690, 7:w692) -> (3:w691:variant)  [unwired: 1 in, 1 out]
                        }
                        frame Error {
                        }
                      }
                    }
                    frame 9..14 {
                      # "SGL, DBL, EXT, CSG, CDB, CXT (0x09 .. 0x0E)"
                      n235 = Variant To Data(type=w696, Variant=w695) -> (data=w697:u8, error out=w699:errorcluster)  [unwired: 1 in]
                      n236 = case shown="No Error" w699 {
                        tunnel: w701 -> [w707 _]
                        tunnel: [w706 w708] -> w700
                        tunnel: w698 -> [_ w708]
                        tunnel: w697 -> [w704 _]
                        tunnel: [TRUE _] -> w694
                        frame No Error {
                          n237 = To Variant(anything=w704) -> (Variant=w703:variant)
                          n238 = Variant To Flattened String(Variant=w703) -> (data string=w705:string)  [unwired: 1 out]
                          n239 = Flattened String To Variant(6:w705, 7:w707) -> (3:w706:variant)  [unwired: 1 in, 1 out]
                        }
                        frame Error {
                        }
                      }
                    }
                    frame 21..23 {
                      # "Enums (0x15 .. 0x17)"
                      n240 = Variant To Data(type=w711, Variant=w710) -> (data=w712:u8, error out=w714:errorcluster)  [unwired: 1 in]
                      n241 = case shown="No Error" w714 {
                        tunnel: w716 -> [w722 _]
                        tunnel: [w721 w723] -> w715
                        tunnel: w713 -> [_ w723]
                        tunnel: w712 -> [w719 _]
                        tunnel: [TRUE _] -> w709
                        frame No Error {
                          n242 = To Variant(anything=w719) -> (Variant=w718:variant)
                          n243 = Variant To Flattened String(Variant=w718) -> (data string=w720:string)  [unwired: 1 out]
                          n244 = Flattened String To Variant(6:w720, 7:w722) -> (3:w721:variant)  [unwired: 1 in, 1 out]
                        }
                        frame Error {
                        }
                      }
                    }
                    frame 25..30 {
                      # "Physical Units (0x19 .. 0x1E)"
                      n245 = Variant To Data(type=w726, Variant=w725) -> (data=w727:u8, error out=w729:errorcluster)  [unwired: 1 in]
                      n246 = case shown="No Error" w729 {
                        tunnel: w731 -> [w737 _]
                        tunnel: [w736 w738] -> w730
                        tunnel: w728 -> [_ w738]
                        tunnel: w727 -> [w734 _]
                        tunnel: [TRUE _] -> w724
                        frame No Error {
                          n247 = To Variant(anything=w734) -> (Variant=w733:variant)
                          n248 = Variant To Flattened String(Variant=w733) -> (data string=w735:string)  [unwired: 1 out]
                          n249 = Flattened String To Variant(6:w735, 7:w737) -> (3:w736:variant)  [unwired: 1 in, 1 out]
                        }
                        frame Error {
                        }
                      }
                    }
                    frame 33 {
                      # "Boolean (0x21)"
                      n250 = Variant To Data(type=FALSE, Variant=w745) -> (data=w742:bool, error out=w743:errorcluster)  [unwired: 1 in]
                      n251 = case shown="No Error" w743 {
                        tunnel: w747 -> [w756 _]
                        tunnel: [w755 w757] -> w746
                        tunnel: w742 -> [w752 _]
                        tunnel: w741 -> [w750 _]
                        tunnel: w740 -> [_ w757]
                        tunnel: [TRUE _] -> w739
                        frame No Error {
                          n252 = Boolean To (0,1)(Boolean=w752) -> (0, 1=w751:i16)
                          n253 = Variant To Data(type=w750, Variant=w751) -> (data=w749:u8)  [unwired: 1 in, 1 out]
                          n254 = To Variant(anything=w749) -> (Variant=w753:variant)
                          n255 = Variant To Flattened String(Variant=w753) -> (data string=w754:string)  [unwired: 1 out]
                          n256 = Flattened String To Variant(6:w754, 7:w756) -> (3:w755:variant)  [unwired: 1 in, 1 out]
                        }
                        frame Error {
                        }
                      }
                    }
                    frame 48 {
                      # "STRING (0x30)"
                      n257 = Variant To Data(type="", Variant=w759) -> (data=w761:string, error out=w763:errorcluster)  [unwired: 1 in]
                      n258 = case shown="No Error" w763 {
                        tunnel: w766 -> [w774 _]
                        tunnel: [w773 w775] -> w764
                        tunnel: w762 -> [_ w775]
                        tunnel: w761 -> [w770 _]
                        tunnel: w760 -> [w768 _]
                        tunnel: [TRUE _] -> w758
                        frame No Error {
                          n259 = Fract/Exp String To Number(string=w770, default (0 dbl)=w768) -> (number=w769:u8)  [unwired: 2 in, 1 out]
                          n260 = To Variant(anything=w769) -> (Variant=w772:variant)
                          n261 = Variant To Flattened String(Variant=w772) -> (data string=w771:string)  [unwired: 1 out]
                          n262 = Flattened String To Variant(6:w771, 7:w774) -> (3:w773:variant)  [unwired: 1 in, 1 out]
                        }
                        frame Error {
                        }
                      }
                    }
                    frame 112 {
                      # "Refnum (0x70)"
                      n263 = Variant To Flattened String(Variant=w778) -> (data string=w777:string)  [unwired: 1 out]
                      n264 = Type Cast(type=w782, x=w777) -> (*(type *) &x=w781:u8)
                      n265 = To Variant(anything=w781) -> (Variant=w780:variant)
                      n266 = Variant To Flattened String(Variant=w780) -> (data string=w779:string)  [unwired: 1 out]
                      n267 = Flattened String To Variant(6:w779, 7:w784) -> (3:w783:variant)  [unwired: 1 in, 1 out]
                    }
                  }
                }
              }
            }
            frame 6 {
              # "U16 (0x06)"
              n268 = Variant To Flattened String(Variant=w791) -> (1:w795:i16[])  [unwired: 1 out]
              n269 = call "TypeDescriptor_GetType.vi"("type descriptor"=w795) -> ("Type"=w785:u8)  [unwired: 9 in, 1 out]
              n270 = Equal?(x=w787, y=w785) -> (x = y?=w789:bool)
              n271 = Compound Arithmetic op=OR(w789, invert w786) -> (w788:bool)
              n272 = case shown="True" w788 {
                tunnel: w794 -> [w796 w803]
                tunnel: [w796 w802] -> w793
                tunnel: w792 -> [_ w801]
                tunnel: w785 -> [_ w800]
                tunnel: w791 -> [_ w798]
                tunnel: [_ w797] -> w790
                frame False {
                }
                frame True {
                  w799 = u16 0  # U16
                  n273 = case shown="1..5, 7, 8" w800 {
                    tunnel: w803 -> [w804 _ w814 w829 w844 w859 w871 w893 _]
                    tunnel: [w804 w806 w816 w831 w846 w861 w877 w895 w914] -> w802
                    tunnel: w801 -> [_ w807 w817 w832 w847 w862 w878 w897 w915]
                    tunnel: w799 -> [_ _ w812 w827 w842 w857 w872 w891 w913]
                    tunnel: w798 -> [_ w809 w811 w826 w841 w856 w876 w890 w909]
                    tunnel: [_ TRUE w810 w825 w840 w855 w870 w889 TRUE] -> w797
                    frame Default {
                      # "INCOMPATIBLE DATATYPES"
                    }
                    frame 6 {
                      # "U16 (0x06)"
                      n274 = Variant To Flattened String(Variant=w809) -> (data string=w808:string)  [unwired: 1 out]
                      n275 = Flattened String To Variant(6:w808, 7:w807) -> (3:w806:variant)  [unwired: 1 in, 1 out]
                    }
                    frame 1..5, 7, 8 {
                      # "I8, I16, I32, I64, U8, U32, U64"
                      n276 = Variant To Data(type=w812, Variant=w811) -> (data=w813:u16, error out=w815:errorcluster)  [unwired: 1 in]
                      n277 = case shown="No Error" w815 {
                        tunnel: w817 -> [w823 _]
                        tunnel: [w822 w824] -> w816
                        tunnel: w814 -> [_ w824]
                        tunnel: w813 -> [w820 _]
                        tunnel: [TRUE _] -> w810
                        frame No Error {
                          n278 = To Variant(anything=w820) -> (Variant=w819:variant)
                          n279 = Variant To Flattened String(Variant=w819) -> (data string=w821:string)  [unwired: 1 out]
                          n280 = Flattened String To Variant(6:w821, 7:w823) -> (3:w822:variant)  [unwired: 1 in, 1 out]
                        }
                        frame Error {
                        }
                      }
                    }
                    frame 9..14 {
                      # "SGL, DBL, EXT, CSG, CDB, CXT (0x09 .. 0x0E)"
                      n281 = Variant To Data(type=w827, Variant=w826) -> (data=w828:u16, error out=w830:errorcluster)  [unwired: 1 in]
                      n282 = case shown="No Error" w830 {
                        tunnel: w832 -> [w838 _]
                        tunnel: [w837 w839] -> w831
                        tunnel: w829 -> [_ w839]
                        tunnel: w828 -> [w835 _]
                        tunnel: [TRUE _] -> w825
                        frame No Error {
                          n283 = To Variant(anything=w835) -> (Variant=w834:variant)
                          n284 = Variant To Flattened String(Variant=w834) -> (data string=w836:string)  [unwired: 1 out]
                          n285 = Flattened String To Variant(6:w836, 7:w838) -> (3:w837:variant)  [unwired: 1 in, 1 out]
                        }
                        frame Error {
                        }
                      }
                    }
                    frame 21..23 {
                      # "Enums (0x15 .. 0x17)"
                      n286 = Variant To Data(type=w842, Variant=w841) -> (data=w843:u16, error out=w845:errorcluster)  [unwired: 1 in]
                      n287 = case shown="No Error" w845 {
                        tunnel: w847 -> [w853 _]
                        tunnel: [w852 w854] -> w846
                        tunnel: w844 -> [_ w854]
                        tunnel: w843 -> [w850 _]
                        tunnel: [TRUE _] -> w840
                        frame No Error {
                          n288 = To Variant(anything=w850) -> (Variant=w849:variant)
                          n289 = Variant To Flattened String(Variant=w849) -> (data string=w851:string)  [unwired: 1 out]
                          n290 = Flattened String To Variant(6:w851, 7:w853) -> (3:w852:variant)  [unwired: 1 in, 1 out]
                        }
                        frame Error {
                        }
                      }
                    }
                    frame 25..30 {
                      # "Physical Units (0x19 .. 0x1E)"
                      n291 = Variant To Data(type=w857, Variant=w856) -> (data=w858:u16, error out=w860:errorcluster)  [unwired: 1 in]
                      n292 = case shown="No Error" w860 {
                        tunnel: w862 -> [w868 _]
                        tunnel: [w867 w869] -> w861
                        tunnel: w859 -> [_ w869]
                        tunnel: w858 -> [w865 _]
                        tunnel: [TRUE _] -> w855
                        frame No Error {
                          n293 = To Variant(anything=w865) -> (Variant=w864:variant)
                          n294 = Variant To Flattened String(Variant=w864) -> (data string=w866:string)  [unwired: 1 out]
                          n295 = Flattened String To Variant(6:w866, 7:w868) -> (3:w867:variant)  [unwired: 1 in, 1 out]
                        }
                        frame Error {
                        }
                      }
                    }
                    frame 33 {
                      # "Boolean (0x21)"
                      n296 = Variant To Data(type=FALSE, Variant=w876) -> (data=w873:bool, error out=w874:errorcluster)  [unwired: 1 in]
                      n297 = case shown="No Error" w874 {
                        tunnel: w878 -> [w887 _]
                        tunnel: [w886 w888] -> w877
                        tunnel: w873 -> [w883 _]
                        tunnel: w872 -> [w881 _]
                        tunnel: w871 -> [_ w888]
                        tunnel: [TRUE _] -> w870
                        frame No Error {
                          n298 = Boolean To (0,1)(Boolean=w883) -> (0, 1=w882:i16)
                          n299 = Variant To Data(type=w881, Variant=w882) -> (data=w880:u16)  [unwired: 1 in, 1 out]
                          n300 = To Variant(anything=w880) -> (Variant=w884:variant)
                          n301 = Variant To Flattened String(Variant=w884) -> (data string=w885:string)  [unwired: 1 out]
                          n302 = Flattened String To Variant(6:w885, 7:w887) -> (3:w886:variant)  [unwired: 1 in, 1 out]
                        }
                        frame Error {
                        }
                      }
                    }
                    frame 48 {
                      # "STRING (0x30)"
                      n303 = Variant To Data(type="", Variant=w890) -> (data=w892:string, error out=w894:errorcluster)  [unwired: 1 in]
                      n304 = case shown="No Error" w894 {
                        tunnel: w897 -> [w905 _]
                        tunnel: [w904 w906] -> w895
                        tunnel: w893 -> [_ w906]
                        tunnel: w892 -> [w901 _]
                        tunnel: w891 -> [w899 _]
                        tunnel: [TRUE _] -> w889
                        frame No Error {
                          n305 = Fract/Exp String To Number(string=w901, default (0 dbl)=w899) -> (number=w900:u16)  [unwired: 2 in, 1 out]
                          n306 = To Variant(anything=w900) -> (Variant=w903:variant)
                          n307 = Variant To Flattened String(Variant=w903) -> (data string=w902:string)  [unwired: 1 out]
                          n308 = Flattened String To Variant(6:w902, 7:w905) -> (3:w904:variant)  [unwired: 1 in, 1 out]
                        }
                        frame Error {
                        }
                      }
                    }
                    frame 112 {
                      # "Refnum (0x70)"
                      n309 = Variant To Flattened String(Variant=w909) -> (data string=w908:string)  [unwired: 1 out]
                      n310 = Type Cast(type=w913, x=w908) -> (*(type *) &x=w912:u16)
                      n311 = To Variant(anything=w912) -> (Variant=w911:variant)
                      n312 = Variant To Flattened String(Variant=w911) -> (data string=w910:string)  [unwired: 1 out]
                      n313 = Flattened String To Variant(6:w910, 7:w915) -> (3:w914:variant)  [unwired: 1 in, 1 out]
                    }
                  }
                }
              }
            }
            frame 7 {
              # "U32 (0x07)"
              n314 = Variant To Flattened String(Variant=w922) -> (1:w926:i16[])  [unwired: 1 out]
              n315 = call "TypeDescriptor_GetType.vi"("type descriptor"=w926) -> ("Type"=w917:u8)  [unwired: 9 in, 1 out]
              n316 = Equal?(x=w918, y=w917) -> (x = y?=w920:bool)
              n317 = Compound Arithmetic op=OR(w920, invert w916) -> (w919:bool)
              n318 = case shown="True" w919 {
                tunnel: w925 -> [w927 w934]
                tunnel: [w927 w933] -> w924
                tunnel: w923 -> [_ w932]
                tunnel: w917 -> [_ w931]
                tunnel: w922 -> [_ w929]
                tunnel: [_ w928] -> w921
                frame False {
                }
                frame True {
                  w930 = u32 0  # U32
                  n319 = case shown="1..6, 8" w931 {
                    tunnel: w934 -> [w935 _ w945 w960 w975 w990 w1002 w1024 _]
                    tunnel: [w935 w937 w947 w962 w977 w992 w1008 w1026 w1045] -> w933
                    tunnel: w932 -> [_ w938 w948 w963 w978 w993 w1009 w1028 w1046]
                    tunnel: w930 -> [_ _ w943 w958 w973 w988 w1003 w1022 w1044]
                    tunnel: w929 -> [_ w940 w942 w957 w972 w987 w1007 w1021 w1040]
                    tunnel: [_ TRUE w941 w956 w971 w986 w1001 w1020 TRUE] -> w928
                    frame Default {
                      # "INCOMPATIBLE DATATYPES"
                    }
                    frame 7 {
                      # "U32 (0x07)"
                      n320 = Variant To Flattened String(Variant=w940) -> (data string=w939:string)  [unwired: 1 out]
                      n321 = Flattened String To Variant(6:w939, 7:w938) -> (3:w937:variant)  [unwired: 1 in, 1 out]
                    }
                    frame 1..6, 8 {
                      # "I8, I16, I32, I64, U8, U16, U64"
                      n322 = Variant To Data(type=w943, Variant=w942) -> (data=w944:u32, error out=w946:errorcluster)  [unwired: 1 in]
                      n323 = case shown="No Error" w946 {
                        tunnel: w948 -> [w954 _]
                        tunnel: [w953 w955] -> w947
                        tunnel: w945 -> [_ w955]
                        tunnel: w944 -> [w951 _]
                        tunnel: [TRUE _] -> w941
                        frame No Error {
                          n324 = To Variant(anything=w951) -> (Variant=w950:variant)
                          n325 = Variant To Flattened String(Variant=w950) -> (data string=w952:string)  [unwired: 1 out]
                          n326 = Flattened String To Variant(6:w952, 7:w954) -> (3:w953:variant)  [unwired: 1 in, 1 out]
                        }
                        frame Error {
                        }
                      }
                    }
                    frame 9..14 {
                      # "SGL, DBL, EXT, CSG, CDB, CXT (0x09 .. 0x0E)"
                      n327 = Variant To Data(type=w958, Variant=w957) -> (data=w959:u32, error out=w961:errorcluster)  [unwired: 1 in]
                      n328 = case shown="No Error" w961 {
                        tunnel: w963 -> [w969 _]
                        tunnel: [w968 w970] -> w962
                        tunnel: w960 -> [_ w970]
                        tunnel: w959 -> [w966 _]
                        tunnel: [TRUE _] -> w956
                        frame No Error {
                          n329 = To Variant(anything=w966) -> (Variant=w965:variant)
                          n330 = Variant To Flattened String(Variant=w965) -> (data string=w967:string)  [unwired: 1 out]
                          n331 = Flattened String To Variant(6:w967, 7:w969) -> (3:w968:variant)  [unwired: 1 in, 1 out]
                        }
                        frame Error {
                        }
                      }
                    }
                    frame 21..23 {
                      # "Enums (0x15 .. 0x17)"
                      n332 = Variant To Data(type=w973, Variant=w972) -> (data=w974:u32, error out=w976:errorcluster)  [unwired: 1 in]
                      n333 = case shown="No Error" w976 {
                        tunnel: w978 -> [w984 _]
                        tunnel: [w983 w985] -> w977
                        tunnel: w975 -> [_ w985]
                        tunnel: w974 -> [w981 _]
                        tunnel: [TRUE _] -> w971
                        frame No Error {
                          n334 = To Variant(anything=w981) -> (Variant=w980:variant)
                          n335 = Variant To Flattened String(Variant=w980) -> (data string=w982:string)  [unwired: 1 out]
                          n336 = Flattened String To Variant(6:w982, 7:w984) -> (3:w983:variant)  [unwired: 1 in, 1 out]
                        }
                        frame Error {
                        }
                      }
                    }
                    frame 25..30 {
                      # "Physical Units (0x19 .. 0x1E)"
                      n337 = Variant To Data(type=w988, Variant=w987) -> (data=w989:u32, error out=w991:errorcluster)  [unwired: 1 in]
                      n338 = case shown="No Error" w991 {
                        tunnel: w993 -> [w999 _]
                        tunnel: [w998 w1000] -> w992
                        tunnel: w990 -> [_ w1000]
                        tunnel: w989 -> [w996 _]
                        tunnel: [TRUE _] -> w986
                        frame No Error {
                          n339 = To Variant(anything=w996) -> (Variant=w995:variant)
                          n340 = Variant To Flattened String(Variant=w995) -> (data string=w997:string)  [unwired: 1 out]
                          n341 = Flattened String To Variant(6:w997, 7:w999) -> (3:w998:variant)  [unwired: 1 in, 1 out]
                        }
                        frame Error {
                        }
                      }
                    }
                    frame 33 {
                      # "Boolean (0x21)"
                      n342 = Variant To Data(type=FALSE, Variant=w1007) -> (data=w1004:bool, error out=w1005:errorcluster)  [unwired: 1 in]
                      n343 = case shown="No Error" w1005 {
                        tunnel: w1009 -> [w1018 _]
                        tunnel: [w1017 w1019] -> w1008
                        tunnel: w1004 -> [w1014 _]
                        tunnel: w1003 -> [w1012 _]
                        tunnel: w1002 -> [_ w1019]
                        tunnel: [TRUE _] -> w1001
                        frame No Error {
                          n344 = Boolean To (0,1)(Boolean=w1014) -> (0, 1=w1013:i16)
                          n345 = Variant To Data(type=w1012, Variant=w1013) -> (data=w1011:u32)  [unwired: 1 in, 1 out]
                          n346 = To Variant(anything=w1011) -> (Variant=w1015:variant)
                          n347 = Variant To Flattened String(Variant=w1015) -> (data string=w1016:string)  [unwired: 1 out]
                          n348 = Flattened String To Variant(6:w1016, 7:w1018) -> (3:w1017:variant)  [unwired: 1 in, 1 out]
                        }
                        frame Error {
                        }
                      }
                    }
                    frame 48 {
                      # "STRING (0x30)"
                      n349 = Variant To Data(type="", Variant=w1021) -> (data=w1023:string, error out=w1025:errorcluster)  [unwired: 1 in]
                      n350 = case shown="No Error" w1025 {
                        tunnel: w1028 -> [w1036 _]
                        tunnel: [w1035 w1037] -> w1026
                        tunnel: w1024 -> [_ w1037]
                        tunnel: w1023 -> [w1032 _]
                        tunnel: w1022 -> [w1030 _]
                        tunnel: [TRUE _] -> w1020
                        frame No Error {
                          n351 = Fract/Exp String To Number(string=w1032, default (0 dbl)=w1030) -> (number=w1031:u32)  [unwired: 2 in, 1 out]
                          n352 = To Variant(anything=w1031) -> (Variant=w1034:variant)
                          n353 = Variant To Flattened String(Variant=w1034) -> (data string=w1033:string)  [unwired: 1 out]
                          n354 = Flattened String To Variant(6:w1033, 7:w1036) -> (3:w1035:variant)  [unwired: 1 in, 1 out]
                        }
                        frame Error {
                        }
                      }
                    }
                    frame 112 {
                      # "Refnum (0x70)"
                      n355 = Variant To Flattened String(Variant=w1040) -> (data string=w1039:string)  [unwired: 1 out]
                      n356 = Type Cast(type=w1044, x=w1039) -> (*(type *) &x=w1043:u32)
                      n357 = To Variant(anything=w1043) -> (Variant=w1042:variant)
                      n358 = Variant To Flattened String(Variant=w1042) -> (data string=w1041:string)  [unwired: 1 out]
                      n359 = Flattened String To Variant(6:w1041, 7:w1046) -> (3:w1045:variant)  [unwired: 1 in, 1 out]
                    }
                  }
                }
              }
            }
            frame 8 {
              # "U64 (0x08)"
              n360 = Variant To Flattened String(Variant=w1053) -> (1:w1057:i16[])  [unwired: 1 out]
              n361 = call "TypeDescriptor_GetType.vi"("type descriptor"=w1057) -> ("Type"=w1047:u8)  [unwired: 9 in, 1 out]
              n362 = Equal?(x=w1049, y=w1047) -> (x = y?=w1051:bool)
              n363 = Compound Arithmetic op=OR(w1051, invert w1048) -> (w1050:bool)
              n364 = case shown="True" w1050 {
                tunnel: w1056 -> [w1058 w1065]
                tunnel: [w1058 w1064] -> w1055
                tunnel: w1054 -> [_ w1063]
                tunnel: w1047 -> [_ w1062]
                tunnel: w1053 -> [_ w1060]
                tunnel: [_ w1059] -> w1052
                frame False {
                }
                frame True {
                  w1061 = u64 0  # U64
                  n365 = case shown="1..7" w1062 {
                    tunnel: w1065 -> [w1066 _ w1076 w1091 w1106 w1121 w1133 w1155 _]
                    tunnel: [w1066 w1068 w1078 w1093 w1108 w1123 w1139 w1157 w1176] -> w1064
                    tunnel: w1063 -> [_ w1069 w1079 w1094 w1109 w1124 w1140 w1159 w1177]
                    tunnel: w1061 -> [_ _ w1074 w1089 w1104 w1119 w1134 w1153 w1175]
                    tunnel: w1060 -> [_ w1071 w1073 w1088 w1103 w1118 w1138 w1152 w1171]
                    tunnel: [_ TRUE w1072 w1087 w1102 w1117 w1132 w1151 TRUE] -> w1059
                    frame Default {
                      # "INCOMPATIBLE DATATYPES"
                    }
                    frame 8 {
                      # "U64 (0x08)"
                      n366 = Variant To Flattened String(Variant=w1071) -> (data string=w1070:string)  [unwired: 1 out]
                      n367 = Flattened String To Variant(6:w1070, 7:w1069) -> (3:w1068:variant)  [unwired: 1 in, 1 out]
                    }
                    frame 1..7 {
                      # "I8, I16, I32, I64, U8, U16, U32"
                      n368 = Variant To Data(type=w1074, Variant=w1073) -> (data=w1075:u64, error out=w1077:errorcluster)  [unwired: 1 in]
                      n369 = case shown="No Error" w1077 {
                        tunnel: w1079 -> [w1085 _]
                        tunnel: [w1084 w1086] -> w1078
                        tunnel: w1076 -> [_ w1086]
                        tunnel: w1075 -> [w1082 _]
                        tunnel: [TRUE _] -> w1072
                        frame No Error {
                          n370 = To Variant(anything=w1082) -> (Variant=w1081:variant)
                          n371 = Variant To Flattened String(Variant=w1081) -> (data string=w1083:string)  [unwired: 1 out]
                          n372 = Flattened String To Variant(6:w1083, 7:w1085) -> (3:w1084:variant)  [unwired: 1 in, 1 out]
                        }
                        frame Error {
                        }
                      }
                    }
                    frame 9..14 {
                      # "SGL, DBL, EXT, CSG, CDB, CXT (0x09 .. 0x0E)"
                      n373 = Variant To Data(type=w1089, Variant=w1088) -> (data=w1090:u64, error out=w1092:errorcluster)  [unwired: 1 in]
                      n374 = case shown="No Error" w1092 {
                        tunnel: w1094 -> [w1100 _]
                        tunnel: [w1099 w1101] -> w1093
                        tunnel: w1091 -> [_ w1101]
                        tunnel: w1090 -> [w1097 _]
                        tunnel: [TRUE _] -> w1087
                        frame No Error {
                          n375 = To Variant(anything=w1097) -> (Variant=w1096:variant)
                          n376 = Variant To Flattened String(Variant=w1096) -> (data string=w1098:string)  [unwired: 1 out]
                          n377 = Flattened String To Variant(6:w1098, 7:w1100) -> (3:w1099:variant)  [unwired: 1 in, 1 out]
                        }
                        frame Error {
                        }
                      }
                    }
                    frame 21..23 {
                      # "Enums (0x15 .. 0x17)"
                      n378 = Variant To Data(type=w1104, Variant=w1103) -> (data=w1105:u64, error out=w1107:errorcluster)  [unwired: 1 in]
                      n379 = case shown="No Error" w1107 {
                        tunnel: w1109 -> [w1115 _]
                        tunnel: [w1114 w1116] -> w1108
                        tunnel: w1106 -> [_ w1116]
                        tunnel: w1105 -> [w1112 _]
                        tunnel: [TRUE _] -> w1102
                        frame No Error {
                          n380 = To Variant(anything=w1112) -> (Variant=w1111:variant)
                          n381 = Variant To Flattened String(Variant=w1111) -> (data string=w1113:string)  [unwired: 1 out]
                          n382 = Flattened String To Variant(6:w1113, 7:w1115) -> (3:w1114:variant)  [unwired: 1 in, 1 out]
                        }
                        frame Error {
                        }
                      }
                    }
                    frame 25..30 {
                      # "Physical Units (0x19 .. 0x1E)"
                      n383 = Variant To Data(type=w1119, Variant=w1118) -> (data=w1120:u64, error out=w1122:errorcluster)  [unwired: 1 in]
                      n384 = case shown="No Error" w1122 {
                        tunnel: w1124 -> [w1130 _]
                        tunnel: [w1129 w1131] -> w1123
                        tunnel: w1121 -> [_ w1131]
                        tunnel: w1120 -> [w1127 _]
                        tunnel: [TRUE _] -> w1117
                        frame No Error {
                          n385 = To Variant(anything=w1127) -> (Variant=w1126:variant)
                          n386 = Variant To Flattened String(Variant=w1126) -> (data string=w1128:string)  [unwired: 1 out]
                          n387 = Flattened String To Variant(6:w1128, 7:w1130) -> (3:w1129:variant)  [unwired: 1 in, 1 out]
                        }
                        frame Error {
                        }
                      }
                    }
                    frame 33 {
                      # "Boolean (0x21)"
                      n388 = Variant To Data(type=FALSE, Variant=w1138) -> (data=w1135:bool, error out=w1136:errorcluster)  [unwired: 1 in]
                      n389 = case shown="No Error" w1136 {
                        tunnel: w1140 -> [w1149 _]
                        tunnel: [w1148 w1150] -> w1139
                        tunnel: w1135 -> [w1145 _]
                        tunnel: w1134 -> [w1143 _]
                        tunnel: w1133 -> [_ w1150]
                        tunnel: [TRUE _] -> w1132
                        frame No Error {
                          n390 = Boolean To (0,1)(Boolean=w1145) -> (0, 1=w1144:i16)
                          n391 = Variant To Data(type=w1143, Variant=w1144) -> (data=w1142:u64)  [unwired: 1 in, 1 out]
                          n392 = To Variant(anything=w1142) -> (Variant=w1146:variant)
                          n393 = Variant To Flattened String(Variant=w1146) -> (data string=w1147:string)  [unwired: 1 out]
                          n394 = Flattened String To Variant(6:w1147, 7:w1149) -> (3:w1148:variant)  [unwired: 1 in, 1 out]
                        }
                        frame Error {
                        }
                      }
                    }
                    frame 48 {
                      # "STRING (0x30)"
                      n395 = Variant To Data(type="", Variant=w1152) -> (data=w1154:string, error out=w1156:errorcluster)  [unwired: 1 in]
                      n396 = case shown="No Error" w1156 {
                        tunnel: w1159 -> [w1167 _]
                        tunnel: [w1166 w1168] -> w1157
                        tunnel: w1155 -> [_ w1168]
                        tunnel: w1154 -> [w1163 _]
                        tunnel: w1153 -> [w1161 _]
                        tunnel: [TRUE _] -> w1151
                        frame No Error {
                          n397 = Fract/Exp String To Number(string=w1163, default (0 dbl)=w1161) -> (number=w1162:u64)  [unwired: 2 in, 1 out]
                          n398 = To Variant(anything=w1162) -> (Variant=w1165:variant)
                          n399 = Variant To Flattened String(Variant=w1165) -> (data string=w1164:string)  [unwired: 1 out]
                          n400 = Flattened String To Variant(6:w1164, 7:w1167) -> (3:w1166:variant)  [unwired: 1 in, 1 out]
                        }
                        frame Error {
                        }
                      }
                    }
                    frame 112 {
                      # "Refnum (0x70)"
                      n401 = Variant To Flattened String(Variant=w1171) -> (data string=w1170:string)  [unwired: 1 out]
                      n402 = Type Cast(type=w1175, x=w1170) -> (*(type *) &x=w1174:u64)
                      n403 = To Variant(anything=w1174) -> (Variant=w1173:variant)
                      n404 = Variant To Flattened String(Variant=w1173) -> (data string=w1172:string)  [unwired: 1 out]
                      n405 = Flattened String To Variant(6:w1172, 7:w1177) -> (3:w1176:variant)  [unwired: 1 in, 1 out]
                    }
                  }
                }
              }
            }
            frame 9 {
              # "SGL (0x09)"
              n406 = Variant To Flattened String(Variant=w1185) -> (1:w1189:i16[])  [unwired: 1 out]
              n407 = call "TypeDescriptor_GetType.vi"("type descriptor"=w1189) -> ("Type"=w1179:u8)  [unwired: 9 in, 1 out]
              n408 = Equal?(x=w1180, y=w1179) -> (x = y?=w1183:bool)
              n409 = Compound Arithmetic op=OR(w1183, invert w1181) -> (w1182:bool)
              n410 = case shown="True" w1182 {
                tunnel: w1188 -> [w1190 w1198]
                tunnel: [w1190 w1197] -> w1187
                tunnel: w1186 -> [_ w1196]
                tunnel: w1179 -> [_ w1195]
                tunnel: w1185 -> [_ w1193]
                tunnel: [_ w1192] -> w1184
                tunnel: w1178 -> [_ w1191]
                frame False {
                }
                frame True {
                  w1194 = sgl 0.0  # SGL
                  n411 = case shown="30" w1195 {
                    tunnel: w1198 -> [w1199 _ w1209 w1224 w1239 w1255]
                    tunnel: [w1199 w1200 w1211 w1226 w1241 w1257] -> w1197
                    tunnel: w1196 -> [_ w1202 w1212 w1227 w1242 w1259]
                    tunnel: w1194 -> [_ _ w1207 w1222 w1237 w1253]
                    tunnel: w1193 -> [_ w1204 w1206 w1221 w1236 w1252]
                    tunnel: [_ TRUE w1205 w1220 w1235 w1251] -> w1192
                    tunnel: w1191 -> [_ _ _ _ _ w1250]
                    frame Default {
                      # "INCOMPATIBLE DATATYPES"
                    }
                    frame 9 {
                      # "SGL (0x09)"
                      n412 = Variant To Flattened String(Variant=w1204) -> (data string=w1203:string)  [unwired: 1 out]
                      n413 = Flattened String To Variant(6:w1203, 7:w1202) -> (3:w1200:variant)  [unwired: 1 in, 1 out]
                    }
                    frame 1..8 {
                      # "I8, I16, I32, I64, U8, U16, U32, U64"
                      n414 = Variant To Data(type=w1207, Variant=w1206) -> (data=w1208:sgl, error out=w1210:errorcluster)  [unwired: 1 in]
                      n415 = case shown="No Error" w1210 {
                        tunnel: w1212 -> [w1218 _]
                        tunnel: [w1217 w1219] -> w1211
                        tunnel: w1209 -> [_ w1219]
                        tunnel: w1208 -> [w1215 _]
                        tunnel: [TRUE _] -> w1205
                        frame No Error {
                          n416 = To Variant(anything=w1215) -> (Variant=w1214:variant)
                          n417 = Variant To Flattened String(Variant=w1214) -> (data string=w1216:string)  [unwired: 1 out]
                          n418 = Flattened String To Variant(6:w1216, 7:w1218) -> (3:w1217:variant)  [unwired: 1 in, 1 out]
                        }
                        frame Error {
                        }
                      }
                    }
                    frame 10..14 {
                      # "DBL, EXT, CSG, CDB, CXT (0x10 .. 0x0E)"
                      n419 = Variant To Data(type=w1222, Variant=w1221) -> (data=w1223:sgl, error out=w1225:errorcluster)  [unwired: 1 in]
                      n420 = case shown="No Error" w1225 {
                        tunnel: w1227 -> [w1233 _]
                        tunnel: [w1232 w1234] -> w1226
                        tunnel: w1224 -> [_ w1234]
                        tunnel: w1223 -> [w1230 _]
                        tunnel: [TRUE _] -> w1220
                        frame No Error {
                          n421 = To Variant(anything=w1230) -> (Variant=w1229:variant)
                          n422 = Variant To Flattened String(Variant=w1229) -> (data string=w1231:string)  [unwired: 1 out]
                          n423 = Flattened String To Variant(6:w1231, 7:w1233) -> (3:w1232:variant)  [unwired: 1 in, 1 out]
                        }
                        frame Error {
                        }
                      }
                    }
                    frame 25..30 {
                      # "Physical Units (0x19 .. 0x1E)"
                      n424 = Variant To Data(type=w1237, Variant=w1236) -> (data=w1238:sgl, error out=w1240:errorcluster)  [unwired: 1 in]
                      n425 = case shown="No Error" w1240 {
                        tunnel: w1242 -> [w1248 _]
                        tunnel: [w1247 w1249] -> w1241
                        tunnel: w1239 -> [_ w1249]
                        tunnel: w1238 -> [w1245 _]
                        tunnel: [TRUE _] -> w1235
                        frame No Error {
                          n426 = To Variant(anything=w1245) -> (Variant=w1244:variant)
                          n427 = Variant To Flattened String(Variant=w1244) -> (data string=w1246:string)  [unwired: 1 out]
                          n428 = Flattened String To Variant(6:w1246, 7:w1248) -> (3:w1247:variant)  [unwired: 1 in, 1 out]
                        }
                        frame Error {
                        }
                      }
                    }
                    frame 48 {
                      # "STRING (0x30)"
                      n429 = Variant To Data(type="", Variant=w1252) -> (data=w1254:string, error out=w1256:errorcluster)  [unwired: 1 in]
                      n430 = case shown="No Error" w1256 {
                        tunnel: w1259 -> [w1266 _]
                        tunnel: [w1265 w1267] -> w1257
                        tunnel: w1255 -> [_ w1267]
                        tunnel: w1254 -> [w1261 _]
                        tunnel: w1253 -> [_ _]
                        tunnel: [TRUE _] -> w1251
                        tunnel: w1250 -> [_ _]
                        frame No Error {
                          n431 = call "String to SingleFloat (Scalar).vi"("Value (String)"=w1261) -> ("Value (Single)"=w1260:sgl)  [unwired: 8 in, 2 out]
                          n432 = To Variant(anything=w1260) -> (Variant=w1264:variant)
                          n433 = Variant To Flattened String(Variant=w1264) -> (data string=w1263:string)  [unwired: 1 out]
                          n434 = Flattened String To Variant(6:w1263, 7:w1266) -> (3:w1265:variant)  [unwired: 1 in, 1 out]
                        }
                        frame Error {
                        }
                      }
                    }
                  }
                }
              }
            }
            frame 10 {
              # "DBL (0xA)"
              n435 = Variant To Flattened String(Variant=w1275) -> (1:w1279:i16[])  [unwired: 1 out]
              n436 = call "TypeDescriptor_GetType.vi"("type descriptor"=w1279) -> ("Type"=w1269:u8)  [unwired: 9 in, 1 out]
              n437 = Equal?(x=w1270, y=w1269) -> (x = y?=w1273:bool)
              n438 = Compound Arithmetic op=OR(w1273, invert w1271) -> (w1272:bool)
              n439 = case shown="True" w1272 {
                tunnel: w1278 -> [w1280 w1288]
                tunnel: [w1280 w1287] -> w1277
                tunnel: w1276 -> [_ w1286]
                tunnel: w1269 -> [_ w1285]
                tunnel: w1275 -> [_ w1283]
                tunnel: [_ w1282] -> w1274
                tunnel: w1268 -> [_ w1281]
                frame False {
                }
                frame True {
                  w1284 = 0.0  # DBL
                  n440 = case shown="30" w1285 {
                    tunnel: w1288 -> [w1289 _ w1299 w1314 w1329 w1344]
                    tunnel: [w1289 w1291 w1301 w1316 w1331 w1346] -> w1287
                    tunnel: w1286 -> [_ w1292 w1302 w1317 w1332 w1348]
                    tunnel: w1284 -> [_ _ w1297 w1312 w1327 _]
                    tunnel: w1283 -> [_ w1294 w1296 w1311 w1326 w1342]
                    tunnel: [_ TRUE w1295 w1310 w1325 w1341] -> w1282
                    tunnel: w1281 -> [_ _ _ _ _ w1340]
                    frame Default {
                      # "INCOMPATIBLE DATATYPES"
                    }
                    frame 10 {
                      # "DBL (0x0A)"
                      n441 = Variant To Flattened String(Variant=w1294) -> (data string=w1293:string)  [unwired: 1 out]
                      n442 = Flattened String To Variant(6:w1293, 7:w1292) -> (3:w1291:variant)  [unwired: 1 in, 1 out]
                    }
                    frame 1..8 {
                      # "I8, I16, I32, I64, U8, U16, U32, U64"
                      n443 = Variant To Data(type=w1297, Variant=w1296) -> (data=w1298:dbl, error out=w1300:errorcluster)  [unwired: 1 in]
                      n444 = case shown="No Error" w1300 {
                        tunnel: w1302 -> [w1308 _]
                        tunnel: [w1307 w1309] -> w1301
                        tunnel: w1299 -> [_ w1309]
                        tunnel: w1298 -> [w1305 _]
                        tunnel: [TRUE _] -> w1295
                        frame No Error {
                          n445 = To Variant(anything=w1305) -> (Variant=w1304:variant)
                          n446 = Variant To Flattened String(Variant=w1304) -> (data string=w1306:string)  [unwired: 1 out]
                          n447 = Flattened String To Variant(6:w1306, 7:w1308) -> (3:w1307:variant)  [unwired: 1 in, 1 out]
                        }
                        frame Error {
                        }
                      }
                    }
                    frame 9, 11..14 {
                      # "SGL, EXT, CSG, CDB, CXT (0x09 .. 0x0E)"
                      n448 = Variant To Data(type=w1312, Variant=w1311) -> (data=w1313:dbl, error out=w1315:errorcluster)  [unwired: 1 in]
                      n449 = case shown="No Error" w1315 {
                        tunnel: w1317 -> [w1323 _]
                        tunnel: [w1322 w1324] -> w1316
                        tunnel: w1314 -> [_ w1324]
                        tunnel: w1313 -> [w1320 _]
                        tunnel: [TRUE _] -> w1310
                        frame No Error {
                          n450 = To Variant(anything=w1320) -> (Variant=w1319:variant)
                          n451 = Variant To Flattened String(Variant=w1319) -> (data string=w1321:string)  [unwired: 1 out]
                          n452 = Flattened String To Variant(6:w1321, 7:w1323) -> (3:w1322:variant)  [unwired: 1 in, 1 out]
                        }
                        frame Error {
                        }
                      }
                    }
                    frame 25..30 {
                      # "Physical Units (0x19 .. 0x1E)"
                      n453 = Variant To Data(type=w1327, Variant=w1326) -> (data=w1328:dbl, error out=w1330:errorcluster)  [unwired: 1 in]
                      n454 = case shown="No Error" w1330 {
                        tunnel: w1332 -> [w1338 _]
                        tunnel: [w1337 w1339] -> w1331
                        tunnel: w1329 -> [_ w1339]
                        tunnel: w1328 -> [w1335 _]
                        tunnel: [TRUE _] -> w1325
                        frame No Error {
                          n455 = To Variant(anything=w1335) -> (Variant=w1334:variant)
                          n456 = Variant To Flattened String(Variant=w1334) -> (data string=w1336:string)  [unwired: 1 out]
                          n457 = Flattened String To Variant(6:w1336, 7:w1338) -> (3:w1337:variant)  [unwired: 1 in, 1 out]
                        }
                        frame Error {
                        }
                      }
                    }
                    frame 48 {
                      # "STRING (0x30)"
                      n458 = Variant To Data(type="", Variant=w1342) -> (data=w1343:string, error out=w1345:errorcluster)  [unwired: 1 in]
                      n459 = case shown="No Error" w1345 {
                        tunnel: w1348 -> [w1355 _]
                        tunnel: [w1354 w1356] -> w1346
                        tunnel: w1344 -> [_ w1356]
                        tunnel: w1343 -> [w1350 _]
                        tunnel: [TRUE _] -> w1341
                        tunnel: w1340 -> [_ _]
                        frame No Error {
                          n460 = call "String to DoubleFloat (Scalar).vi"("Value (String)"=w1350) -> ("Value (Double)"=w1349:dbl)  [unwired: 8 in, 2 out]
                          n461 = To Variant(anything=w1349) -> (Variant=w1353:variant)
                          n462 = Variant To Flattened String(Variant=w1353) -> (data string=w1352:string)  [unwired: 1 out]
                          n463 = Flattened String To Variant(6:w1352, 7:w1355) -> (3:w1354:variant)  [unwired: 1 in, 1 out]
                        }
                        frame Error {
                        }
                      }
                    }
                  }
                }
              }
            }
            frame 11 {
              # "EXT (0x0B)"
              n464 = Variant To Flattened String(Variant=w1364) -> (1:w1368:i16[])  [unwired: 1 out]
              n465 = call "TypeDescriptor_GetType.vi"("type descriptor"=w1368) -> ("Type"=w1359:u8)  [unwired: 9 in, 1 out]
              n466 = Equal?(x=w1360, y=w1359) -> (x = y?=w1362:bool)
              n467 = Compound Arithmetic op=OR(w1362, invert w1358) -> (w1361:bool)
              n468 = case shown="True" w1361 {
                tunnel: w1367 -> [w1369 w1377]
                tunnel: [w1369 w1376] -> w1366
                tunnel: w1365 -> [_ w1375]
                tunnel: w1359 -> [_ w1374]
                tunnel: w1364 -> [_ w1372]
                tunnel: [_ w1371] -> w1363
                tunnel: w1357 -> [_ w1370]
                frame False {
                }
                frame True {
                  w1373 = ext 0.0  # EXT
                  n469 = case shown="30" w1374 {
                    tunnel: w1377 -> [w1378 _ w1388 w1403 w1418 w1434]
                    tunnel: [w1378 w1379 w1390 w1405 w1420 w1436] -> w1376
                    tunnel: w1375 -> [_ w1381 w1391 w1406 w1421 w1438]
                    tunnel: w1373 -> [_ _ w1386 w1401 w1416 w1432]
                    tunnel: w1372 -> [_ w1383 w1385 w1400 w1415 w1431]
                    tunnel: [_ TRUE w1384 w1399 w1414 w1430] -> w1371
                    tunnel: w1370 -> [_ _ _ _ _ w1429]
                    frame Default {
                      # "INCOMPATIBLE DATATYPES"
                    }
                    frame 11 {
                      # "EXT (0x0B)"
                      n470 = Variant To Flattened String(Variant=w1383) -> (data string=w1382:string)  [unwired: 1 out]
                      n471 = Flattened String To Variant(6:w1382, 7:w1381) -> (3:w1379:variant)  [unwired: 1 in, 1 out]
                    }
                    frame 1..8 {
                      # "I8, I16, I32, I64, U8, U16, U32, U64"
                      n472 = Variant To Data(type=w1386, Variant=w1385) -> (data=w1387:ext, error out=w1389:errorcluster)  [unwired: 1 in]
                      n473 = case shown="No Error" w1389 {
                        tunnel: w1391 -> [w1397 _]
                        tunnel: [w1396 w1398] -> w1390
                        tunnel: w1388 -> [_ w1398]
                        tunnel: w1387 -> [w1394 _]
                        tunnel: [TRUE _] -> w1384
                        frame No Error {
                          n474 = To Variant(anything=w1394) -> (Variant=w1393:variant)
                          n475 = Variant To Flattened String(Variant=w1393) -> (data string=w1395:string)  [unwired: 1 out]
                          n476 = Flattened String To Variant(6:w1395, 7:w1397) -> (3:w1396:variant)  [unwired: 1 in, 1 out]
                        }
                        frame Error {
                        }
                      }
                    }
                    frame 9, 10, 12..14 {
                      # "SGL, DBL, CSG, CDB, CXT (0x09 .. 0x0E)"
                      n477 = Variant To Data(type=w1401, Variant=w1400) -> (data=w1402:ext, error out=w1404:errorcluster)  [unwired: 1 in]
                      n478 = case shown="No Error" w1404 {
                        tunnel: w1406 -> [w1412 _]
                        tunnel: [w1411 w1413] -> w1405
                        tunnel: w1403 -> [_ w1413]
                        tunnel: w1402 -> [w1409 _]
                        tunnel: [TRUE _] -> w1399
                        frame No Error {
                          n479 = To Variant(anything=w1409) -> (Variant=w1408:variant)
                          n480 = Variant To Flattened String(Variant=w1408) -> (data string=w1410:string)  [unwired: 1 out]
                          n481 = Flattened String To Variant(6:w1410, 7:w1412) -> (3:w1411:variant)  [unwired: 1 in, 1 out]
                        }
                        frame Error {
                        }
                      }
                    }
                    frame 25..30 {
                      # "Physical Units (0x19 .. 0x1E)"
                      n482 = Variant To Data(type=w1416, Variant=w1415) -> (data=w1417:ext, error out=w1419:errorcluster)  [unwired: 1 in]
                      n483 = case shown="No Error" w1419 {
                        tunnel: w1421 -> [w1427 _]
                        tunnel: [w1426 w1428] -> w1420
                        tunnel: w1418 -> [_ w1428]
                        tunnel: w1417 -> [w1424 _]
                        tunnel: [TRUE _] -> w1414
                        frame No Error {
                          n484 = To Variant(anything=w1424) -> (Variant=w1423:variant)
                          n485 = Variant To Flattened String(Variant=w1423) -> (data string=w1425:string)  [unwired: 1 out]
                          n486 = Flattened String To Variant(6:w1425, 7:w1427) -> (3:w1426:variant)  [unwired: 1 in, 1 out]
                        }
                        frame Error {
                        }
                      }
                    }
                    frame 48 {
                      # "STRING (0x30)"
                      n487 = Variant To Data(type="", Variant=w1431) -> (data=w1433:string, error out=w1435:errorcluster)  [unwired: 1 in]
                      n488 = case shown="No Error" w1435 {
                        tunnel: w1438 -> [w1445 _]
                        tunnel: [w1444 w1446] -> w1436
                        tunnel: w1434 -> [_ w1446]
                        tunnel: w1433 -> [w1440 _]
                        tunnel: w1432 -> [_ _]
                        tunnel: [TRUE _] -> w1430
                        tunnel: w1429 -> [_ _]
                        frame No Error {
                          n489 = call "String to ExtendedFloat (Scalar).vi"("Value (String)"=w1440) -> ("Value (Extended)"=w1439:ext)  [unwired: 8 in, 2 out]
                          n490 = To Variant(anything=w1439) -> (Variant=w1443:variant)
                          n491 = Variant To Flattened String(Variant=w1443) -> (data string=w1442:string)  [unwired: 1 out]
                          n492 = Flattened String To Variant(6:w1442, 7:w1445) -> (3:w1444:variant)  [unwired: 1 in, 1 out]
                        }
                        frame Error {
                        }
                      }
                    }
                  }
                }
              }
            }
            frame 12 {
              # "CSG (0x0C)"
              n493 = Variant To Flattened String(Variant=w1453) -> (1:w1457:i16[])  [unwired: 1 out]
              n494 = call "TypeDescriptor_GetType.vi"("type descriptor"=w1457) -> ("Type"=w1448:u8)  [unwired: 9 in, 1 out]
              n495 = Equal?(x=w1449, y=w1448) -> (x = y?=w1451:bool)
              n496 = Compound Arithmetic op=OR(w1451, invert w1447) -> (w1450:bool)
              n497 = case shown="True" w1450 {
                tunnel: w1456 -> [w1458 w1465]
                tunnel: [w1458 w1464] -> w1455
                tunnel: w1454 -> [_ w1463]
                tunnel: w1448 -> [_ w1462]
                tunnel: w1453 -> [_ w1460]
                tunnel: [_ w1459] -> w1452
                frame False {
                }
                frame True {
                  w1461 = csg 0.0+0.0i  # CSG
                  n498 = case shown="30" w1462 {
                    tunnel: w1465 -> [w1466 _ w1476 w1491 w1506 w1521]
                    tunnel: [w1466 w1467 w1478 w1493 w1508 w1523] -> w1464
                    tunnel: w1463 -> [_ w1469 w1479 w1494 w1509 w1524]
                    tunnel: w1461 -> [_ _ w1474 w1489 w1504 _]
                    tunnel: w1460 -> [_ w1471 w1473 w1488 w1503 w1519]
                    tunnel: [_ TRUE w1472 w1487 w1502 w1518] -> w1459
                    frame Default {
                      # "INCOMPATIBLE DATATYPES"
                    }
                    frame 12 {
                      # "CSG (0x0C)"
                      n499 = Variant To Flattened String(Variant=w1471) -> (data string=w1470:string)  [unwired: 1 out]
                      n500 = Flattened String To Variant(6:w1470, 7:w1469) -> (3:w1467:variant)  [unwired: 1 in, 1 out]
                    }
                    frame 1..8 {
                      # "I8, I16, I32, I64, U8, U16, U32, U64"
                      n501 = Variant To Data(type=w1474, Variant=w1473) -> (data=w1475:csg, error out=w1477:errorcluster)  [unwired: 1 in]
                      n502 = case shown="No Error" w1477 {
                        tunnel: w1479 -> [w1485 _]
                        tunnel: [w1484 w1486] -> w1478
                        tunnel: w1476 -> [_ w1486]
                        tunnel: w1475 -> [w1482 _]
                        tunnel: [TRUE _] -> w1472
                        frame No Error {
                          n503 = To Variant(anything=w1482) -> (Variant=w1481:variant)
                          n504 = Variant To Flattened String(Variant=w1481) -> (data string=w1483:string)  [unwired: 1 out]
                          n505 = Flattened String To Variant(6:w1483, 7:w1485) -> (3:w1484:variant)  [unwired: 1 in, 1 out]
                        }
                        frame Error {
                        }
                      }
                    }
                    frame 9..11, 13, 14 {
                      # "SGL, DBL, EXT, CDB, CXT (0x09 .. 0x0E)"
                      n506 = Variant To Data(type=w1489, Variant=w1488) -> (data=w1490:csg, error out=w1492:errorcluster)  [unwired: 1 in]
                      n507 = case shown="No Error" w1492 {
                        tunnel: w1494 -> [w1500 _]
                        tunnel: [w1499 w1501] -> w1493
                        tunnel: w1491 -> [_ w1501]
                        tunnel: w1490 -> [w1497 _]
                        tunnel: [TRUE _] -> w1487
                        frame No Error {
                          n508 = To Variant(anything=w1497) -> (Variant=w1496:variant)
                          n509 = Variant To Flattened String(Variant=w1496) -> (data string=w1498:string)  [unwired: 1 out]
                          n510 = Flattened String To Variant(6:w1498, 7:w1500) -> (3:w1499:variant)  [unwired: 1 in, 1 out]
                        }
                        frame Error {
                        }
                      }
                    }
                    frame 25..30 {
                      # "Physical Units (0x19 .. 0x1E)"
                      n511 = Variant To Data(type=w1504, Variant=w1503) -> (data=w1505:csg, error out=w1507:errorcluster)  [unwired: 1 in]
                      n512 = case shown="No Error" w1507 {
                        tunnel: w1509 -> [w1515 _]
                        tunnel: [w1514 w1516] -> w1508
                        tunnel: w1506 -> [_ w1516]
                        tunnel: w1505 -> [w1512 _]
                        tunnel: [TRUE _] -> w1502
                        frame No Error {
                          n513 = To Variant(anything=w1512) -> (Variant=w1511:variant)
                          n514 = Variant To Flattened String(Variant=w1511) -> (data string=w1513:string)  [unwired: 1 out]
                          n515 = Flattened String To Variant(6:w1513, 7:w1515) -> (3:w1514:variant)  [unwired: 1 in, 1 out]
                        }
                        frame Error {
                        }
                      }
                    }
                    frame 48 {
                      # "String (0x30)"
                      n516 = Variant To Data(type="", Variant=w1519) -> (data=w1520:string, error out=w1522:errorcluster)  [unwired: 1 in]
                      n517 = case shown="No Error" w1522 {
                        tunnel: w1524 -> [w1531 _]
                        tunnel: [w1530 w1532] -> w1523
                        tunnel: w1521 -> [_ w1532]
                        tunnel: w1520 -> [w1526 _]
                        tunnel: [TRUE _] -> w1518
                        frame No Error {
                          n518 = call "String to SingleComplex (Scalar).vi"("Value (String)"=w1526) -> ("Value (CSG)"=w1525:csg)  [unwired: 8 in, 2 out]
                          n519 = To Variant(anything=w1525) -> (Variant=w1528:variant)
                          n520 = Variant To Flattened String(Variant=w1528) -> (data string=w1529:string)  [unwired: 1 out]
                          n521 = Flattened String To Variant(6:w1529, 7:w1531) -> (3:w1530:variant)  [unwired: 1 in, 1 out]
                        }
                        frame Error {
                        }
                      }
                    }
                  }
                }
              }
            }
            frame 13 {
              # "CDB (0x0D)"
              n522 = Variant To Flattened String(Variant=w1540) -> (1:w1543:i16[])  [unwired: 1 out]
              n523 = call "TypeDescriptor_GetType.vi"("type descriptor"=w1543) -> ("Type"=w1533:u8)  [unwired: 9 in, 1 out]
              n524 = Equal?(x=w1535, y=w1533) -> (x = y?=w1537:bool)
              n525 = Compound Arithmetic op=OR(w1537, invert w1534) -> (w1536:bool)
              n526 = case shown="True" w1536 {
                tunnel: [w1544 w1550] -> w1542
                tunnel: w1541 -> [_ w1549]
                tunnel: w1533 -> [_ w1548]
                tunnel: w1540 -> [_ w1546]
                tunnel: [_ w1545] -> w1539
                tunnel: w1538 -> [w1544 w1551]
                frame False {
                }
                frame True {
                  w1547 = cdb 0.0+0.0i  # CDB
                  n527 = case shown="30" w1548 {
                    tunnel: w1551 -> [w1552 _ w1562 w1577 w1592 w1607]
                    tunnel: [w1552 w1553 w1564 w1579 w1594 w1609] -> w1550
                    tunnel: w1549 -> [_ w1555 w1565 w1580 w1595 w1610]
                    tunnel: w1547 -> [_ _ w1560 w1575 w1590 _]
                    tunnel: w1546 -> [_ w1557 w1559 w1574 w1589 w1605]
                    tunnel: [_ TRUE w1558 w1573 w1588 w1604] -> w1545
                    frame Default {
                      # "INCOMPATIBLE DATATYPES"
                    }
                    frame 13 {
                      # "CDB (0x0D)"
                      n528 = Variant To Flattened String(Variant=w1557) -> (data string=w1556:string)  [unwired: 1 out]
                      n529 = Flattened String To Variant(6:w1556, 7:w1555) -> (3:w1553:variant)  [unwired: 1 in, 1 out]
                    }
                    frame 1..8 {
                      # "I8, I16, I32, I64, U8, U16, U32, U64"
                      n530 = Variant To Data(type=w1560, Variant=w1559) -> (data=w1561:cdb, error out=w1563:errorcluster)  [unwired: 1 in]
                      n531 = case shown="No Error" w1563 {
                        tunnel: w1565 -> [w1571 _]
                        tunnel: [w1570 w1572] -> w1564
                        tunnel: w1562 -> [_ w1572]
                        tunnel: w1561 -> [w1568 _]
                        tunnel: [TRUE _] -> w1558
                        frame No Error {
                          n532 = To Variant(anything=w1568) -> (Variant=w1567:variant)
                          n533 = Variant To Flattened String(Variant=w1567) -> (data string=w1569:string)  [unwired: 1 out]
                          n534 = Flattened String To Variant(6:w1569, 7:w1571) -> (3:w1570:variant)  [unwired: 1 in, 1 out]
                        }
                        frame Error {
                        }
                      }
                    }
                    frame 9..12, 14 {
                      # "SGL, DBL, EXT, CSG, CXT (0x09 .. 0x0E)"
                      n535 = Variant To Data(type=w1575, Variant=w1574) -> (data=w1576:cdb, error out=w1578:errorcluster)  [unwired: 1 in]
                      n536 = case shown="No Error" w1578 {
                        tunnel: w1580 -> [w1586 _]
                        tunnel: [w1585 w1587] -> w1579
                        tunnel: w1577 -> [_ w1587]
                        tunnel: w1576 -> [w1583 _]
                        tunnel: [TRUE _] -> w1573
                        frame No Error {
                          n537 = To Variant(anything=w1583) -> (Variant=w1582:variant)
                          n538 = Variant To Flattened String(Variant=w1582) -> (data string=w1584:string)  [unwired: 1 out]
                          n539 = Flattened String To Variant(6:w1584, 7:w1586) -> (3:w1585:variant)  [unwired: 1 in, 1 out]
                        }
                        frame Error {
                        }
                      }
                    }
                    frame 25..30 {
                      # "Physical Units (0x19 .. 0x1E)"
                      n540 = Variant To Data(type=w1590, Variant=w1589) -> (data=w1591:cdb, error out=w1593:errorcluster)  [unwired: 1 in]
                      n541 = case shown="No Error" w1593 {
                        tunnel: w1595 -> [w1601 _]
                        tunnel: [w1600 w1602] -> w1594
                        tunnel: w1592 -> [_ w1602]
                        tunnel: w1591 -> [w1598 _]
                        tunnel: [TRUE _] -> w1588
                        frame No Error {
                          n542 = To Variant(anything=w1598) -> (Variant=w1597:variant)
                          n543 = Variant To Flattened String(Variant=w1597) -> (data string=w1599:string)  [unwired: 1 out]
                          n544 = Flattened String To Variant(6:w1599, 7:w1601) -> (3:w1600:variant)  [unwired: 1 in, 1 out]
                        }
                        frame Error {
                        }
                      }
                    }
                    frame 48 {
                      # "String (0x30)"
                      n545 = Variant To Data(type="", Variant=w1605) -> (data=w1606:string, error out=w1608:errorcluster)  [unwired: 1 in]
                      n546 = case shown="No Error" w1608 {
                        tunnel: w1610 -> [w1617 _]
                        tunnel: [w1616 w1618] -> w1609
                        tunnel: w1607 -> [_ w1618]
                        tunnel: w1606 -> [w1612 _]
                        tunnel: [TRUE _] -> w1604
                        frame No Error {
                          n547 = call "String to DoubleComplex (Scalar).vi"("Value (String)"=w1612) -> ("Value (CDB)"=w1611:cdb)  [unwired: 8 in, 2 out]
                          n548 = To Variant(anything=w1611) -> (Variant=w1614:variant)
                          n549 = Variant To Flattened String(Variant=w1614) -> (data string=w1615:string)  [unwired: 1 out]
                          n550 = Flattened String To Variant(6:w1615, 7:w1617) -> (3:w1616:variant)  [unwired: 1 in, 1 out]
                        }
                        frame Error {
                        }
                      }
                    }
                  }
                }
              }
            }
            frame 14 {
              # "CXT (0x0E)"
              n551 = Variant To Flattened String(Variant=w1625) -> (1:w1629:i16[])  [unwired: 1 out]
              n552 = call "TypeDescriptor_GetType.vi"("type descriptor"=w1629) -> ("Type"=w1619:u8)  [unwired: 9 in, 1 out]
              n553 = Equal?(x=w1620, y=w1619) -> (x = y?=w1623:bool)
              n554 = Compound Arithmetic op=OR(w1623, invert w1621) -> (w1622:bool)
              n555 = case shown="True" w1622 {
                tunnel: w1628 -> [w1630 w1637]
                tunnel: [w1630 w1636] -> w1627
                tunnel: w1626 -> [_ w1635]
                tunnel: w1619 -> [_ w1634]
                tunnel: w1625 -> [_ w1632]
                tunnel: [_ w1631] -> w1624
                frame False {
                }
                frame True {
                  w1633 = cxt 0.0+0.0i  # CXT
                  n556 = case shown="30" w1634 {
                    tunnel: w1637 -> [w1638 _ w1648 w1663 w1678 w1693]
                    tunnel: [w1638 w1639 w1650 w1665 w1680 w1695] -> w1636
                    tunnel: w1635 -> [_ w1641 w1651 w1666 w1681 w1696]
                    tunnel: w1633 -> [_ _ w1646 w1661 w1676 _]
                    tunnel: w1632 -> [_ w1643 w1645 w1660 w1675 w1691]
                    tunnel: [_ TRUE w1644 w1659 w1674 w1690] -> w1631
                    frame Default {
                      # "INCOMPATIBLE DATATYPES"
                    }
                    frame 14 {
                      # "CXT (0x0E)"
                      n557 = Variant To Flattened String(Variant=w1643) -> (data string=w1642:string)  [unwired: 1 out]
                      n558 = Flattened String To Variant(6:w1642, 7:w1641) -> (3:w1639:variant)  [unwired: 1 in, 1 out]
                    }
                    frame 1..8 {
                      # "I8, I16, I32, I64, U8, U16, U32, U64"
                      n559 = Variant To Data(type=w1646, Variant=w1645) -> (data=w1647:cxt, error out=w1649:errorcluster)  [unwired: 1 in]
                      n560 = case shown="No Error" w1649 {
                        tunnel: w1651 -> [w1657 _]
                        tunnel: [w1656 w1658] -> w1650
                        tunnel: w1648 -> [_ w1658]
                        tunnel: w1647 -> [w1654 _]
                        tunnel: [TRUE _] -> w1644
                        frame No Error {
                          n561 = To Variant(anything=w1654) -> (Variant=w1653:variant)
                          n562 = Variant To Flattened String(Variant=w1653) -> (data string=w1655:string)  [unwired: 1 out]
                          n563 = Flattened String To Variant(6:w1655, 7:w1657) -> (3:w1656:variant)  [unwired: 1 in, 1 out]
                        }
                        frame Error {
                        }
                      }
                    }
                    frame 9..13 {
                      # "SGL, DBL, EXT, CSG, CDB (0x09 .. 0x0E)"
                      n564 = Variant To Data(type=w1661, Variant=w1660) -> (data=w1662:cxt, error out=w1664:errorcluster)  [unwired: 1 in]
                      n565 = case shown="No Error" w1664 {
                        tunnel: w1666 -> [w1672 _]
                        tunnel: [w1671 w1673] -> w1665
                        tunnel: w1663 -> [_ w1673]
                        tunnel: w1662 -> [w1669 _]
                        tunnel: [TRUE _] -> w1659
                        frame No Error {
                          n566 = To Variant(anything=w1669) -> (Variant=w1668:variant)
                          n567 = Variant To Flattened String(Variant=w1668) -> (data string=w1670:string)  [unwired: 1 out]
                          n568 = Flattened String To Variant(6:w1670, 7:w1672) -> (3:w1671:variant)  [unwired: 1 in, 1 out]
                        }
                        frame Error {
                        }
                      }
                    }
                    frame 25..30 {
                      # "Physical Units (0x19 .. 0x1E)"
                      n569 = Variant To Data(type=w1676, Variant=w1675) -> (data=w1677:cxt, error out=w1679:errorcluster)  [unwired: 1 in]
                      n570 = case shown="No Error" w1679 {
                        tunnel: w1681 -> [w1687 _]
                        tunnel: [w1686 w1688] -> w1680
                        tunnel: w1678 -> [_ w1688]
                        tunnel: w1677 -> [w1684 _]
                        tunnel: [TRUE _] -> w1674
                        frame No Error {
                          n571 = To Variant(anything=w1684) -> (Variant=w1683:variant)
                          n572 = Variant To Flattened String(Variant=w1683) -> (data string=w1685:string)  [unwired: 1 out]
                          n573 = Flattened String To Variant(6:w1685, 7:w1687) -> (3:w1686:variant)  [unwired: 1 in, 1 out]
                        }
                        frame Error {
                        }
                      }
                    }
                    frame 48 {
                      # "String (0x30)"
                      n574 = Variant To Data(type="", Variant=w1691) -> (data=w1692:string, error out=w1694:errorcluster)  [unwired: 1 in]
                      n575 = case shown="No Error" w1694 {
                        tunnel: w1696 -> [w1703 _]
                        tunnel: [w1702 w1704] -> w1695
                        tunnel: w1693 -> [_ w1704]
                        tunnel: w1692 -> [w1698 _]
                        tunnel: [TRUE _] -> w1690
                        frame No Error {
                          n576 = call "String to ExtendedComplex (Scalar).vi"("Value (String)"=w1698) -> ("Value (CXT)"=w1697:cxt)  [unwired: 8 in, 2 out]
                          n577 = To Variant(anything=w1697) -> (Variant=w1700:variant)
                          n578 = Variant To Flattened String(Variant=w1700) -> (data string=w1701:string)  [unwired: 1 out]
                          n579 = Flattened String To Variant(6:w1701, 7:w1703) -> (3:w1702:variant)  [unwired: 1 in, 1 out]
                        }
                        frame Error {
                        }
                      }
                    }
                  }
                }
              }
            }
            frame 23 {
              # "Enum U32 (0x17)"
              n580 = Variant To Flattened String(Variant=w1711) -> (1:w1715:i16[])  [unwired: 1 out]
              n581 = call "TypeDescriptor_GetType.vi"("type descriptor"=w1715) -> ("Type"=w1705:u8)  [unwired: 9 in, 1 out]
              n582 = Equal?(x=w1706, y=w1705) -> (x = y?=w1709:bool)
              n583 = Compound Arithmetic op=OR(w1709, invert w1707) -> (w1708:bool)
              n584 = case shown="True" w1708 {
                tunnel: w1714 -> [w1716 w1718]
                tunnel: [w1716 w1723] -> w1713
                tunnel: w1712 -> [_ w1722]
                tunnel: w1705 -> [_ w1721]
                tunnel: w1711 -> [_ w1717]
                tunnel: [_ w1719] -> w1710
                frame False {
                }
                frame True {
                  w1720 = u32 0  # U32
                  n585 = case shown="16" w1721 {
                    tunnel: w1718 -> [w1724 w1726 _ _ _ w1762 w1784 w1799]
                    tunnel: [w1724 w1732 w1743 w1752 w1760 w1770 w1786 w1801] -> w1723
                    tunnel: w1722 -> [_ w1725 w1744 w1745 w1753 w1767 w1787 w1802]
                    tunnel: w1720 -> [_ w1729 _ _ _ w1764 w1782 w1797]
                    tunnel: w1717 -> [_ w1728 w1741 w1750 w1758 w1768 w1781 w1796]
                    tunnel: [_ w1727 TRUE TRUE TRUE w1761 w1780 w1795] -> w1719
                    frame Default {
                      # "INCOMPATIBLE DATATYPES"
                    }
                    frame 1..8 {
                      # "I8, I16, I32, I64, U8, U16, U32, U64"
                      n586 = Variant To Data(type=w1729, Variant=w1728) -> (data=w1730:u32, error out=w1731:errorcluster)  [unwired: 1 in]
                      n587 = case shown="No Error" w1731 {
                        tunnel: w1725 -> [w1738 _]
                        tunnel: [w1737 w1739] -> w1732
                        tunnel: w1726 -> [_ w1739]
                        tunnel: w1730 -> [w1735 _]
                        tunnel: [TRUE _] -> w1727
                        frame No Error {
                          n588 = To Variant(anything=w1735) -> (Variant=w1734:variant)
                          n589 = Variant To Flattened String(Variant=w1734) -> (data string=w1736:string)  [unwired: 1 out]
                          n590 = Flattened String To Variant(6:w1736, 7:w1738) -> (3:w1737:variant)  [unwired: 1 in, 1 out]
                        }
                        frame Error {
                        }
                      }
                    }
                    frame 23 {
                      # "Enum U32"
                      n591 = Variant To Flattened String(Variant=w1741) -> (data string=w1740:string)  [unwired: 1 out]
                      n592 = Flattened String To Variant(6:w1740, 7:w1744) -> (3:w1743:variant)  [unwired: 1 in, 1 out]
                    }
                    frame 22 {
                      # "Enum U16"
                      n593 = Variant To Flattened String(Variant=w1750) -> (data string=w1749:string)  [unwired: 1 out]
                      n594 = Byte Array To String(unsigned byte array=u8[] [0, 0]) -> (string=w1748:string)
                      n595 = Concatenate Strings(w1748, w1749) -> (w1746:string)
                      n596 = Flattened String To Variant(6:w1746, 7:w1745) -> (3:w1752:variant)  [unwired: 1 in, 1 out]
                    }
                    frame 21 {
                      # "Enum U8"
                      n597 = Variant To Flattened String(Variant=w1758) -> (data string=w1757:string)  [unwired: 1 out]
                      n598 = Byte Array To String(unsigned byte array=u8[] [0, 0, 0]) -> (string=w1756:string)
                      n599 = Concatenate Strings(w1756, w1757) -> (w1754:string)
                      n600 = Flattened String To Variant(6:w1754, 7:w1753) -> (3:w1760:variant)  [unwired: 1 in, 1 out]
                    }
                    frame 48 {
                      # "String (0x30)"
                      n601 = call "TypeDescriptor_ListElementNames.vi"("type descriptor"=w1767) -> ("element names"=w1766:string[])  [unwired: 7 in, 3 out]
                      n602 = Variant To Data(type="", Variant=w1768) -> (data=w1765:string)  [unwired: 1 in, 1 out]
                      n603 = Search 1D Array(1D array=w1766, element=w1765) -> (index of element=w1763:i32)  [unwired: 1 in]
                      n604 = case shown="Default" w1763 {
                        selector: w1763 -> [_ w1773]
                        tunnel: [w1771 w1779] -> w1770
                        tunnel: w1767 -> [_ w1778]
                        tunnel: w1764 -> [_ w1776]
                        tunnel: w1762 -> [w1771 _]
                        tunnel: [_ TRUE] -> w1761
                        frame -1 {
                        }
                        frame Default {
                          n605 = Variant To Data(type=w1776, Variant=w1773) -> (data=w1775:u32)  [unwired: 1 in, 1 out]
                          n606 = To Variant(anything=w1775) -> (Variant=w1777:variant)
                          n607 = Variant To Flattened String(Variant=w1777) -> (data string=w1774:string)  [unwired: 1 out]
                          n608 = Flattened String To Variant(6:w1774, 7:w1778) -> (3:w1779:variant)  [unwired: 1 in, 1 out]
                        }
                      }
                    }
                    frame 9..13 {
                      # "SGL, DBL, EXT, CSG, CDB (0x09 .. 0x0E)"
                      n609 = Variant To Data(type=w1782, Variant=w1781) -> (data=w1783:u32, error out=w1785:errorcluster)  [unwired: 1 in]
                      n610 = case shown="No Error" w1785 {
                        tunnel: w1787 -> [w1793 _]
                        tunnel: [w1792 w1794] -> w1786
                        tunnel: w1784 -> [_ w1794]
                        tunnel: w1783 -> [w1790 _]
                        tunnel: [TRUE _] -> w1780
                        frame No Error {
                          n611 = To Variant(anything=w1790) -> (Variant=w1789:variant)
                          n612 = Variant To Flattened String(Variant=w1789) -> (data string=w1791:string)  [unwired: 1 out]
                          n613 = Flattened String To Variant(6:w1791, 7:w1793) -> (3:w1792:variant)  [unwired: 1 in, 1 out]
                        }
                        frame Error {
                        }
                      }
                    }
                    frame 25..30 {
                      # "Physical Units (0x19 .. 0x1E)"
                      n614 = Variant To Data(type=w1797, Variant=w1796) -> (data=w1798:u32, error out=w1800:errorcluster)  [unwired: 1 in]
                      n615 = case shown="No Error" w1800 {
                        tunnel: w1802 -> [w1808 _]
                        tunnel: [w1807 w1809] -> w1801
                        tunnel: w1799 -> [_ w1809]
                        tunnel: w1798 -> [w1805 _]
                        tunnel: [TRUE _] -> w1795
                        frame No Error {
                          n616 = To Variant(anything=w1805) -> (Variant=w1804:variant)
                          n617 = Variant To Flattened String(Variant=w1804) -> (data string=w1806:string)  [unwired: 1 out]
                          n618 = Flattened String To Variant(6:w1806, 7:w1808) -> (3:w1807:variant)  [unwired: 1 in, 1 out]
                        }
                        frame Error {
                        }
                      }
                    }
                  }
                }
              }
            }
            frame 22 {
              # "Enum U16 (0x16)"
              n619 = Variant To Flattened String(Variant=w1816) -> (1:w1820:i16[])  [unwired: 1 out]
              n620 = call "TypeDescriptor_GetType.vi"("type descriptor"=w1820) -> ("Type"=w1810:u8)  [unwired: 9 in, 1 out]
              n621 = Equal?(x=w1811, y=w1810) -> (x = y?=w1814:bool)
              n622 = Compound Arithmetic op=OR(w1814, invert w1812) -> (w1813:bool)
              n623 = case shown="True" w1813 {
                tunnel: w1819 -> [w1821 w1823]
                tunnel: [w1821 w1828] -> w1818
                tunnel: w1817 -> [_ w1827]
                tunnel: w1810 -> [_ w1826]
                tunnel: w1816 -> [_ w1822]
                tunnel: [_ w1824] -> w1815
                frame False {
                }
                frame True {
                  w1825 = u16 0  # U16
                  n624 = case shown="30" w1826 {
                    tunnel: w1823 -> [w1829 w1831 _ _ _ w1866 w1888 w1903]
                    tunnel: [w1829 w1837 w1848 w1856 w1864 w1874 w1890 w1905] -> w1828
                    tunnel: w1827 -> [_ w1830 w1849 w1853 w1857 w1871 w1891 w1906]
                    tunnel: w1825 -> [_ w1834 _ _ _ w1868 w1886 w1901]
                    tunnel: w1822 -> [_ w1833 w1846 w1854 w1862 w1872 w1885 w1900]
                    tunnel: [_ w1832 TRUE TRUE TRUE w1865 w1884 w1899] -> w1824
                    frame Default {
                      # "INCOMPATIBLE DATATYPES"
                    }
                    frame 1..8 {
                      # "I8, I16, I32, I64, U8, U16, U32, U64"
                      n625 = Variant To Data(type=w1834, Variant=w1833) -> (data=w1835:u16, error out=w1836:errorcluster)  [unwired: 1 in]
                      n626 = case shown="No Error" w1836 {
                        tunnel: w1830 -> [w1843 _]
                        tunnel: [w1842 w1844] -> w1837
                        tunnel: w1831 -> [_ w1844]
                        tunnel: w1835 -> [w1840 _]
                        tunnel: [TRUE _] -> w1832
                        frame No Error {
                          n627 = To Variant(anything=w1840) -> (Variant=w1839:variant)
                          n628 = Variant To Flattened String(Variant=w1839) -> (data string=w1841:string)  [unwired: 1 out]
                          n629 = Flattened String To Variant(6:w1841, 7:w1843) -> (3:w1842:variant)  [unwired: 1 in, 1 out]
                        }
                        frame Error {
                        }
                      }
                    }
                    frame 22 {
                      # "Enum U16"
                      n630 = Variant To Flattened String(Variant=w1846) -> (data string=w1845:string)  [unwired: 1 out]
                      n631 = Flattened String To Variant(6:w1845, 7:w1849) -> (3:w1848:variant)  [unwired: 1 in, 1 out]
                    }
                    frame 23 {
                      # "Enum U32"
                      n632 = Variant To Flattened String(Variant=w1854) -> (data string=w1852:string)  [unwired: 1 out]
                      n633 = String Subset(string=w1852, offset (0)=2) -> (substring=w1850:string)  [unwired: 1 in]
                      n634 = Flattened String To Variant(6:w1850, 7:w1853) -> (3:w1856:variant)  [unwired: 1 in, 1 out]
                    }
                    frame 21 {
                      # "Enum U8"
                      n635 = Variant To Flattened String(Variant=w1862) -> (data string=w1861:string)  [unwired: 1 out]
                      n636 = Byte Array To String(unsigned byte array=u8[] [0]) -> (string=w1860:string)
                      n637 = Concatenate Strings(w1860, w1861) -> (w1858:string)
                      n638 = Flattened String To Variant(6:w1858, 7:w1857) -> (3:w1864:variant)  [unwired: 1 in, 1 out]
                    }
                    frame 48 {
                      # "String (0x30)"
                      n639 = call "TypeDescriptor_ListElementNames.vi"("type descriptor"=w1871) -> ("element names"=w1870:string[])  [unwired: 7 in, 3 out]
                      n640 = Variant To Data(type="", Variant=w1872) -> (data=w1869:string)  [unwired: 1 in, 1 out]
                      n641 = Search 1D Array(1D array=w1870, element=w1869) -> (index of element=w1867:i32)  [unwired: 1 in]
                      n642 = case shown="Default" w1867 {
                        selector: w1867 -> [_ w1877]
                        tunnel: [w1875 w1883] -> w1874
                        tunnel: w1871 -> [_ w1882]
                        tunnel: w1868 -> [_ w1880]
                        tunnel: w1866 -> [w1875 _]
                        tunnel: [_ TRUE] -> w1865
                        frame -1 {
                        }
                        frame Default {
                          n643 = Variant To Data(type=w1880, Variant=w1877) -> (data=w1879:u16)  [unwired: 1 in, 1 out]
                          n644 = To Variant(anything=w1879) -> (Variant=w1881:variant)
                          n645 = Variant To Flattened String(Variant=w1881) -> (data string=w1878:string)  [unwired: 1 out]
                          n646 = Flattened String To Variant(6:w1878, 7:w1882) -> (3:w1883:variant)  [unwired: 1 in, 1 out]
                        }
                      }
                    }
                    frame 9..13 {
                      # "SGL, DBL, EXT, CSG, CDB (0x09 .. 0x0E)"
                      n647 = Variant To Data(type=w1886, Variant=w1885) -> (data=w1887:u16, error out=w1889:errorcluster)  [unwired: 1 in]
                      n648 = case shown="No Error" w1889 {
                        tunnel: w1891 -> [w1897 _]
                        tunnel: [w1896 w1898] -> w1890
                        tunnel: w1888 -> [_ w1898]
                        tunnel: w1887 -> [w1894 _]
                        tunnel: [TRUE _] -> w1884
                        frame No Error {
                          n649 = To Variant(anything=w1894) -> (Variant=w1893:variant)
                          n650 = Variant To Flattened String(Variant=w1893) -> (data string=w1895:string)  [unwired: 1 out]
                          n651 = Flattened String To Variant(6:w1895, 7:w1897) -> (3:w1896:variant)  [unwired: 1 in, 1 out]
                        }
                        frame Error {
                        }
                      }
                    }
                    frame 25..30 {
                      # "Physical Units (0x19 .. 0x1E)"
                      n652 = Variant To Data(type=w1901, Variant=w1900) -> (data=w1902:u16, error out=w1904:errorcluster)  [unwired: 1 in]
                      n653 = case shown="No Error" w1904 {
                        tunnel: w1906 -> [w1912 _]
                        tunnel: [w1911 w1913] -> w1905
                        tunnel: w1903 -> [_ w1913]
                        tunnel: w1902 -> [w1909 _]
                        tunnel: [TRUE _] -> w1899
                        frame No Error {
                          n654 = To Variant(anything=w1909) -> (Variant=w1908:variant)
                          n655 = Variant To Flattened String(Variant=w1908) -> (data string=w1910:string)  [unwired: 1 out]
                          n656 = Flattened String To Variant(6:w1910, 7:w1912) -> (3:w1911:variant)  [unwired: 1 in, 1 out]
                        }
                        frame Error {
                        }
                      }
                    }
                  }
                }
              }
            }
            frame 21 {
              # "Enum U8 (0x15)"
              n657 = Variant To Flattened String(Variant=w1920) -> (1:w1924:i16[])  [unwired: 1 out]
              n658 = call "TypeDescriptor_GetType.vi"("type descriptor"=w1924) -> ("Type"=w1914:u8)  [unwired: 9 in, 1 out]
              n659 = Equal?(x=w1915, y=w1914) -> (x = y?=w1918:bool)
              n660 = Compound Arithmetic op=OR(w1918, invert w1916) -> (w1917:bool)
              n661 = case shown="True" w1917 {
                tunnel: w1923 -> [w1925 w1927]
                tunnel: [w1925 w1932] -> w1922
                tunnel: w1921 -> [_ w1931]
                tunnel: w1914 -> [_ w1930]
                tunnel: w1920 -> [_ w1926]
                tunnel: [_ w1928] -> w1919
                frame False {
                }
                frame True {
                  w1929 = u8 0  # U8
                  n662 = case shown="30" w1930 {
                    tunnel: w1927 -> [w1933 w1935 _ _ _ w1969 w1991 w2006]
                    tunnel: [w1933 w1941 w1952 w1960 w1967 w1977 w1993 w2008] -> w1932
                    tunnel: w1931 -> [_ w1934 w1953 w1957 w1964 w1974 w1994 w2009]
                    tunnel: w1929 -> [_ w1938 _ _ _ w1971 w1989 w2004]
                    tunnel: w1926 -> [_ w1937 w1950 w1958 w1965 w1975 w1988 w2003]
                    tunnel: [_ w1936 TRUE TRUE TRUE w1968 w1987 w2002] -> w1928
                    frame Default {
                      # "INCOMPATIBLE DATATYPES"
                    }
                    frame 1..8 {
                      # "I8, I16, I32, I64, U8, U16, U32, U64"
                      n663 = Variant To Data(type=w1938, Variant=w1937) -> (data=w1939:u8, error out=w1940:errorcluster)  [unwired: 1 in]
                      n664 = case shown="No Error" w1940 {
                        tunnel: w1934 -> [w1947 _]
                        tunnel: [w1946 w1948] -> w1941
                        tunnel: w1935 -> [_ w1948]
                        tunnel: w1939 -> [w1944 _]
                        tunnel: [TRUE _] -> w1936
                        frame No Error {
                          n665 = To Variant(anything=w1944) -> (Variant=w1943:variant)
                          n666 = Variant To Flattened String(Variant=w1943) -> (data string=w1945:string)  [unwired: 1 out]
                          n667 = Flattened String To Variant(6:w1945, 7:w1947) -> (3:w1946:variant)  [unwired: 1 in, 1 out]
                        }
                        frame Error {
                        }
                      }
                    }
                    frame 21 {
                      # "Enum U8"
                      n668 = Variant To Flattened String(Variant=w1950) -> (data string=w1949:string)  [unwired: 1 out]
                      n669 = Flattened String To Variant(6:w1949, 7:w1953) -> (3:w1952:variant)  [unwired: 1 in, 1 out]
                    }
                    frame 23 {
                      # "Enum U32"
                      n670 = Variant To Flattened String(Variant=w1958) -> (data string=w1956:string)  [unwired: 1 out]
                      n671 = String Subset(string=w1956, offset (0)=3) -> (substring=w1954:string)  [unwired: 1 in]
                      n672 = Flattened String To Variant(6:w1954, 7:w1957) -> (3:w1960:variant)  [unwired: 1 in, 1 out]
                    }
                    frame 22 {
                      # "Enum U16"
                      n673 = Variant To Flattened String(Variant=w1965) -> (data string=w1963:string)  [unwired: 1 out]
                      n674 = String Subset(string=w1963, offset (0)=1) -> (substring=w1962:string)  [unwired: 1 in]
                      n675 = Flattened String To Variant(6:w1962, 7:w1964) -> (3:w1967:variant)  [unwired: 1 in, 1 out]
                    }
                    frame 48 {
                      # "String (0x30)"
                      n676 = call "TypeDescriptor_ListElementNames.vi"("type descriptor"=w1974) -> ("element names"=w1973:string[])  [unwired: 7 in, 3 out]
                      n677 = Variant To Data(type="", Variant=w1975) -> (data=w1972:string)  [unwired: 1 in, 1 out]
                      n678 = Search 1D Array(1D array=w1973, element=w1972) -> (index of element=w1970:i32)  [unwired: 1 in]
                      n679 = case shown="Default" w1970 {
                        selector: w1970 -> [_ w1980]
                        tunnel: [w1978 w1986] -> w1977
                        tunnel: w1974 -> [_ w1985]
                        tunnel: w1971 -> [_ w1983]
                        tunnel: w1969 -> [w1978 _]
                        tunnel: [_ TRUE] -> w1968
                        frame -1 {
                        }
                        frame Default {
                          n680 = Variant To Data(type=w1983, Variant=w1980) -> (data=w1982:u8)  [unwired: 1 in, 1 out]
                          n681 = To Variant(anything=w1982) -> (Variant=w1984:variant)
                          n682 = Variant To Flattened String(Variant=w1984) -> (data string=w1981:string)  [unwired: 1 out]
                          n683 = Flattened String To Variant(6:w1981, 7:w1985) -> (3:w1986:variant)  [unwired: 1 in, 1 out]
                        }
                      }
                    }
                    frame 9..13 {
                      # "SGL, DBL, EXT, CSG, CDB (0x09 .. 0x0E)"
                      n684 = Variant To Data(type=w1989, Variant=w1988) -> (data=w1990:u8, error out=w1992:errorcluster)  [unwired: 1 in]
                      n685 = case shown="No Error" w1992 {
                        tunnel: w1994 -> [w2000 _]
                        tunnel: [w1999 w2001] -> w1993
                        tunnel: w1991 -> [_ w2001]
                        tunnel: w1990 -> [w1997 _]
                        tunnel: [TRUE _] -> w1987
                        frame No Error {
                          n686 = To Variant(anything=w1997) -> (Variant=w1996:variant)
                          n687 = Variant To Flattened String(Variant=w1996) -> (data string=w1998:string)  [unwired: 1 out]
                          n688 = Flattened String To Variant(6:w1998, 7:w2000) -> (3:w1999:variant)  [unwired: 1 in, 1 out]
                        }
                        frame Error {
                        }
                      }
                    }
                    frame 25..30 {
                      # "Physical Units (0x19 .. 0x1E)"
                      n689 = Variant To Data(type=w2004, Variant=w2003) -> (data=w2005:u8, error out=w2007:errorcluster)  [unwired: 1 in]
                      n690 = case shown="No Error" w2007 {
                        tunnel: w2009 -> [w2015 _]
                        tunnel: [w2014 w2016] -> w2008
                        tunnel: w2006 -> [_ w2016]
                        tunnel: w2005 -> [w2012 _]
                        tunnel: [TRUE _] -> w2002
                        frame No Error {
                          n691 = To Variant(anything=w2012) -> (Variant=w2011:variant)
                          n692 = Variant To Flattened String(Variant=w2011) -> (data string=w2013:string)  [unwired: 1 out]
                          n693 = Flattened String To Variant(6:w2013, 7:w2015) -> (3:w2014:variant)  [unwired: 1 in, 1 out]
                        }
                        frame Error {
                        }
                      }
                    }
                  }
                }
              }
            }
            frame 25 {
              # "SGL PhysUnit (0x19)"
              n694 = Variant To Flattened String(Variant=w2023) -> (1:w2027:i16[])  [unwired: 1 out]
              n695 = call "TypeDescriptor_GetType.vi"("type descriptor"=w2027) -> ("Type"=w2018:u8)  [unwired: 9 in, 1 out]
              n696 = Equal?(x=w2017, y=w2018) -> (x = y?=w2021:bool)
              n697 = Compound Arithmetic op=OR(w2021, invert w2019) -> (w2020:bool)
              n698 = case shown="True" w2020 {
                tunnel: w2026 -> [w2028 w2035]
                tunnel: [w2028 w2034] -> w2025
                tunnel: w2024 -> [_ w2033]
                tunnel: w2018 -> [_ w2032]
                tunnel: w2023 -> [_ w2030]
                tunnel: [_ w2029] -> w2022
                frame False {
                }
                frame True {
                  w2031 = sgl 0.0  # SGL
                  n699 = case shown="1..8" w2032 {
                    tunnel: w2035 -> [w2036 _ w2046 w2061 w2076]
                    tunnel: [w2036 w2038 w2048 w2063 w2078] -> w2034
                    tunnel: w2033 -> [_ w2039 w2049 w2064 w2079]
                    tunnel: w2031 -> [_ _ w2044 w2059 w2074]
                    tunnel: w2030 -> [_ w2041 w2043 w2058 w2073]
                    tunnel: [_ TRUE w2042 w2057 w2072] -> w2029
                    frame Default {
                      # "INCOMPATIBLE DATATYPES"
                    }
                    frame 25 {
                      # "SGL PhysUnit (0x19)"
                      n700 = Variant To Flattened String(Variant=w2041) -> (data string=w2040:string)  [unwired: 1 out]
                      n701 = Flattened String To Variant(6:w2040, 7:w2039) -> (3:w2038:variant)  [unwired: 1 in, 1 out]
                    }
                    frame 1..8 {
                      # "I8, I16, I32, I64, U8, U16, U32, U64"
                      n702 = Variant To Data(type=w2044, Variant=w2043) -> (data=w2045:sgl, error out=w2047:errorcluster)  [unwired: 1 in]
                      n703 = case shown="No Error" w2047 {
                        tunnel: w2049 -> [w2055 _]
                        tunnel: [w2054 w2056] -> w2048
                        tunnel: w2046 -> [_ w2056]
                        tunnel: w2045 -> [w2052 _]
                        tunnel: [TRUE _] -> w2042
                        frame No Error {
                          n704 = To Variant(anything=w2052) -> (Variant=w2051:variant)
                          n705 = Variant To Flattened String(Variant=w2051) -> (data string=w2053:string)  [unwired: 1 out]
                          n706 = Flattened String To Variant(6:w2053, 7:w2055) -> (3:w2054:variant)  [unwired: 1 in, 1 out]
                        }
                        frame Error {
                        }
                      }
                    }
                    frame 9..14 {
                      # "SGL, DBL, EXT, CSG, CDB (0x09 .. 0x0E)"
                      n707 = Variant To Data(type=w2059, Variant=w2058) -> (data=w2060:sgl, error out=w2062:errorcluster)  [unwired: 1 in]
                      n708 = case shown="No Error" w2062 {
                        tunnel: w2064 -> [w2070 _]
                        tunnel: [w2069 w2071] -> w2063
                        tunnel: w2061 -> [_ w2071]
                        tunnel: w2060 -> [w2067 _]
                        tunnel: [TRUE _] -> w2057
                        frame No Error {
                          n709 = To Variant(anything=w2067) -> (Variant=w2066:variant)
                          n710 = Variant To Flattened String(Variant=w2066) -> (data string=w2068:string)  [unwired: 1 out]
                          n711 = Flattened String To Variant(6:w2068, 7:w2070) -> (3:w2069:variant)  [unwired: 1 in, 1 out]
                        }
                        frame Error {
                        }
                      }
                    }
                    frame 26..30 {
                      # "Physical Units (0x19 .. 0x1E)"
                      n712 = Variant To Data(type=w2074, Variant=w2073) -> (data=w2075:sgl, error out=w2077:errorcluster)  [unwired: 1 in]
                      n713 = case shown="No Error" w2077 {
                        tunnel: w2079 -> [w2085 _]
                        tunnel: [w2084 w2086] -> w2078
                        tunnel: w2076 -> [_ w2086]
                        tunnel: w2075 -> [w2082 _]
                        tunnel: [TRUE _] -> w2072
                        frame No Error {
                          n714 = To Variant(anything=w2082) -> (Variant=w2081:variant)
                          n715 = Variant To Flattened String(Variant=w2081) -> (data string=w2083:string)  [unwired: 1 out]
                          n716 = Flattened String To Variant(6:w2083, 7:w2085) -> (3:w2084:variant)  [unwired: 1 in, 1 out]
                        }
                        frame Error {
                        }
                      }
                    }
                  }
                }
              }
            }
            frame 26 {
              # "DBL PhysUnit (0x1A)"
              n717 = Variant To Flattened String(Variant=w2093) -> (1:w2097:i16[])  [unwired: 1 out]
              n718 = call "TypeDescriptor_GetType.vi"("type descriptor"=w2097) -> ("Type"=w2088:u8)  [unwired: 9 in, 1 out]
              n719 = Equal?(x=w2089, y=w2088) -> (x = y?=w2091:bool)
              n720 = Compound Arithmetic op=OR(w2091, invert w2087) -> (w2090:bool)
              n721 = case shown="True" w2090 {
                tunnel: w2096 -> [w2098 w2105]
                tunnel: [w2098 w2104] -> w2095
                tunnel: w2094 -> [_ w2103]
                tunnel: w2088 -> [_ w2102]
                tunnel: w2093 -> [_ w2100]
                tunnel: [_ w2099] -> w2092
                frame False {
                }
                frame True {
                  w2101 = 0.0  # DBL
                  n722 = case shown="1..8" w2102 {
                    tunnel: w2105 -> [w2106 _ w2116 w2131 w2146]
                    tunnel: [w2106 w2108 w2118 w2133 w2148] -> w2104
                    tunnel: w2103 -> [_ w2109 w2119 w2134 w2149]
                    tunnel: w2101 -> [_ _ w2114 w2129 w2144]
                    tunnel: w2100 -> [_ w2111 w2113 w2128 w2143]
                    tunnel: [_ TRUE w2112 w2127 w2142] -> w2099
                    frame Default {
                      # "INCOMPATIBLE DATATYPES"
                    }
                    frame 26 {
                      # "DBL PhysUnit (0x1A)"
                      n723 = Variant To Flattened String(Variant=w2111) -> (data string=w2110:string)  [unwired: 1 out]
                      n724 = Flattened String To Variant(6:w2110, 7:w2109) -> (3:w2108:variant)  [unwired: 1 in, 1 out]
                    }
                    frame 1..8 {
                      # "I8, I16, I32, I64, U8, U16, U32, U64"
                      n725 = Variant To Data(type=w2114, Variant=w2113) -> (data=w2115:dbl, error out=w2117:errorcluster)  [unwired: 1 in]
                      n726 = case shown="No Error" w2117 {
                        tunnel: w2119 -> [w2125 _]
                        tunnel: [w2124 w2126] -> w2118
                        tunnel: w2116 -> [_ w2126]
                        tunnel: w2115 -> [w2122 _]
                        tunnel: [TRUE _] -> w2112
                        frame No Error {
                          n727 = To Variant(anything=w2122) -> (Variant=w2121:variant)
                          n728 = Variant To Flattened String(Variant=w2121) -> (data string=w2123:string)  [unwired: 1 out]
                          n729 = Flattened String To Variant(6:w2123, 7:w2125) -> (3:w2124:variant)  [unwired: 1 in, 1 out]
                        }
                        frame Error {
                        }
                      }
                    }
                    frame 9..14 {
                      # "SGL, DBL, EXT, CSG, CDB (0x09 .. 0x0E)"
                      n730 = Variant To Data(type=w2129, Variant=w2128) -> (data=w2130:dbl, error out=w2132:errorcluster)  [unwired: 1 in]
                      n731 = case shown="No Error" w2132 {
                        tunnel: w2134 -> [w2140 _]
                        tunnel: [w2139 w2141] -> w2133
                        tunnel: w2131 -> [_ w2141]
                        tunnel: w2130 -> [w2137 _]
                        tunnel: [TRUE _] -> w2127
                        frame No Error {
                          n732 = To Variant(anything=w2137) -> (Variant=w2136:variant)
                          n733 = Variant To Flattened String(Variant=w2136) -> (data string=w2138:string)  [unwired: 1 out]
                          n734 = Flattened String To Variant(6:w2138, 7:w2140) -> (3:w2139:variant)  [unwired: 1 in, 1 out]
                        }
                        frame Error {
                        }
                      }
                    }
                    frame 25, 27..30 {
                      # "Physical Units (0x19 .. 0x1E)"
                      n735 = Variant To Data(type=w2144, Variant=w2143) -> (data=w2145:dbl, error out=w2147:errorcluster)  [unwired: 1 in]
                      n736 = case shown="No Error" w2147 {
                        tunnel: w2149 -> [w2155 _]
                        tunnel: [w2154 w2156] -> w2148
                        tunnel: w2146 -> [_ w2156]
                        tunnel: w2145 -> [w2152 _]
                        tunnel: [TRUE _] -> w2142
                        frame No Error {
                          n737 = To Variant(anything=w2152) -> (Variant=w2151:variant)
                          n738 = Variant To Flattened String(Variant=w2151) -> (data string=w2153:string)  [unwired: 1 out]
                          n739 = Flattened String To Variant(6:w2153, 7:w2155) -> (3:w2154:variant)  [unwired: 1 in, 1 out]
                        }
                        frame Error {
                        }
                      }
                    }
                  }
                }
              }
            }
            frame 27 {
              # "EXT PhysUnit (0x1B)"
              n740 = Variant To Flattened String(Variant=w2163) -> (1:w2167:i16[])  [unwired: 1 out]
              n741 = call "TypeDescriptor_GetType.vi"("type descriptor"=w2167) -> ("Type"=w2157:u8)  [unwired: 9 in, 1 out]
              n742 = Equal?(x=w2158, y=w2157) -> (x = y?=w2161:bool)
              n743 = Compound Arithmetic op=OR(w2161, invert w2159) -> (w2160:bool)
              n744 = case shown="True" w2160 {
                tunnel: w2166 -> [w2168 w2175]
                tunnel: [w2168 w2174] -> w2165
                tunnel: w2164 -> [_ w2173]
                tunnel: w2157 -> [_ w2172]
                tunnel: w2163 -> [_ w2170]
                tunnel: [_ w2169] -> w2162
                frame False {
                }
                frame True {
                  w2171 = ext 0.0  # EXT
                  n745 = case shown="1..8" w2172 {
                    tunnel: w2175 -> [w2176 _ w2186 w2201 w2216]
                    tunnel: [w2176 w2178 w2188 w2203 w2218] -> w2174
                    tunnel: w2173 -> [_ w2179 w2189 w2204 w2219]
                    tunnel: w2171 -> [_ _ w2184 w2199 w2214]
                    tunnel: w2170 -> [_ w2181 w2183 w2198 w2213]
                    tunnel: [_ TRUE w2182 w2197 w2212] -> w2169
                    frame Default {
                      # "INCOMPATIBLE DATATYPES"
                    }
                    frame 27 {
                      # "EXT PhysUnit (0x1B)"
                      n746 = Variant To Flattened String(Variant=w2181) -> (data string=w2180:string)  [unwired: 1 out]
                      n747 = Flattened String To Variant(6:w2180, 7:w2179) -> (3:w2178:variant)  [unwired: 1 in, 1 out]
                    }
                    frame 1..8 {
                      # "I8, I16, I32, I64, U8, U16, U32, U64"
                      n748 = Variant To Data(type=w2184, Variant=w2183) -> (data=w2185:ext, error out=w2187:errorcluster)  [unwired: 1 in]
                      n749 = case shown="No Error" w2187 {
                        tunnel: w2189 -> [w2195 _]
                        tunnel: [w2194 w2196] -> w2188
                        tunnel: w2186 -> [_ w2196]
                        tunnel: w2185 -> [w2192 _]
                        tunnel: [TRUE _] -> w2182
                        frame No Error {
                          n750 = To Variant(anything=w2192) -> (Variant=w2191:variant)
                          n751 = Variant To Flattened String(Variant=w2191) -> (data string=w2193:string)  [unwired: 1 out]
                          n752 = Flattened String To Variant(6:w2193, 7:w2195) -> (3:w2194:variant)  [unwired: 1 in, 1 out]
                        }
                        frame Error {
                        }
                      }
                    }
                    frame 9..14 {
                      # "SGL, DBL, EXT, CSG, CDB (0x09 .. 0x0E)"
                      n753 = Variant To Data(type=w2199, Variant=w2198) -> (data=w2200:ext, error out=w2202:errorcluster)  [unwired: 1 in]
                      n754 = case shown="No Error" w2202 {
                        tunnel: w2204 -> [w2210 _]
                        tunnel: [w2209 w2211] -> w2203
                        tunnel: w2201 -> [_ w2211]
                        tunnel: w2200 -> [w2207 _]
                        tunnel: [TRUE _] -> w2197
                        frame No Error {
                          n755 = To Variant(anything=w2207) -> (Variant=w2206:variant)
                          n756 = Variant To Flattened String(Variant=w2206) -> (data string=w2208:string)  [unwired: 1 out]
                          n757 = Flattened String To Variant(6:w2208, 7:w2210) -> (3:w2209:variant)  [unwired: 1 in, 1 out]
                        }
                        frame Error {
                        }
                      }
                    }
                    frame 25, 26, 28..30 {
                      # "Physical Units (0x19 .. 0x1E)"
                      n758 = Variant To Data(type=w2214, Variant=w2213) -> (data=w2215:ext, error out=w2217:errorcluster)  [unwired: 1 in]
                      n759 = case shown="No Error" w2217 {
                        tunnel: w2219 -> [w2225 _]
                        tunnel: [w2224 w2226] -> w2218
                        tunnel: w2216 -> [_ w2226]
                        tunnel: w2215 -> [w2222 _]
                        tunnel: [TRUE _] -> w2212
                        frame No Error {
                          n760 = To Variant(anything=w2222) -> (Variant=w2221:variant)
                          n761 = Variant To Flattened String(Variant=w2221) -> (data string=w2223:string)  [unwired: 1 out]
                          n762 = Flattened String To Variant(6:w2223, 7:w2225) -> (3:w2224:variant)  [unwired: 1 in, 1 out]
                        }
                        frame Error {
                        }
                      }
                    }
                  }
                }
              }
            }
            frame 28 {
              # "CSG PhysUnit (0x1C)"
              n763 = Variant To Flattened String(Variant=w2233) -> (1:w2237:i16[])  [unwired: 1 out]
              n764 = call "TypeDescriptor_GetType.vi"("type descriptor"=w2237) -> ("Type"=w2230:u8)  [unwired: 9 in, 1 out]
              n765 = Equal?(x=w2229, y=w2230) -> (x = y?=w2231:bool)
              n766 = Compound Arithmetic op=OR(w2231, invert w2228) -> (w2227:bool)
              n767 = case shown="True" w2227 {
                tunnel: w2236 -> [w2238 w2245]
                tunnel: [w2238 w2244] -> w2235
                tunnel: w2234 -> [_ w2243]
                tunnel: w2233 -> [_ w2241]
                tunnel: [_ w2240] -> w2232
                tunnel: w2230 -> [_ w2239]
                frame False {
                }
                frame True {
                  w2242 = csg 0.0+0.0i  # CSG
                  n768 = case shown="1..8" w2239 {
                    tunnel: w2245 -> [w2246 _ w2256 w2271 w2286]
                    tunnel: [w2246 w2248 w2258 w2273 w2288] -> w2244
                    tunnel: w2243 -> [_ w2249 w2259 w2274 w2289]
                    tunnel: w2242 -> [_ _ w2254 w2269 w2284]
                    tunnel: w2241 -> [_ w2251 w2253 w2268 w2283]
                    tunnel: [_ TRUE w2252 w2267 w2282] -> w2240
                    frame Default {
                      # "INCOMPATIBLE DATATYPES"
                    }
                    frame 28 {
                      # "CSG PhysUnit (0x1C)"
                      n769 = Variant To Flattened String(Variant=w2251) -> (data string=w2250:string)  [unwired: 1 out]
                      n770 = Flattened String To Variant(6:w2250, 7:w2249) -> (3:w2248:variant)  [unwired: 1 in, 1 out]
                    }
                    frame 1..8 {
                      # "I8, I16, I32, I64, U8, U16, U32, U64"
                      n771 = Variant To Data(type=w2254, Variant=w2253) -> (data=w2255:csg, error out=w2257:errorcluster)  [unwired: 1 in]
                      n772 = case shown="No Error" w2257 {
                        tunnel: w2259 -> [w2265 _]
                        tunnel: [w2264 w2266] -> w2258
                        tunnel: w2256 -> [_ w2266]
                        tunnel: w2255 -> [w2262 _]
                        tunnel: [TRUE _] -> w2252
                        frame No Error {
                          n773 = To Variant(anything=w2262) -> (Variant=w2261:variant)
                          n774 = Variant To Flattened String(Variant=w2261) -> (data string=w2263:string)  [unwired: 1 out]
                          n775 = Flattened String To Variant(6:w2263, 7:w2265) -> (3:w2264:variant)  [unwired: 1 in, 1 out]
                        }
                        frame Error {
                        }
                      }
                    }
                    frame 9..14 {
                      # "SGL, DBL, EXT, CSG, CDB (0x09 .. 0x0E)"
                      n776 = Variant To Data(type=w2269, Variant=w2268) -> (data=w2270:csg, error out=w2272:errorcluster)  [unwired: 1 in]
                      n777 = case shown="No Error" w2272 {
                        tunnel: w2274 -> [w2280 _]
                        tunnel: [w2279 w2281] -> w2273
                        tunnel: w2271 -> [_ w2281]
                        tunnel: w2270 -> [w2277 _]
                        tunnel: [TRUE _] -> w2267
                        frame No Error {
                          n778 = To Variant(anything=w2277) -> (Variant=w2276:variant)
                          n779 = Variant To Flattened String(Variant=w2276) -> (data string=w2278:string)  [unwired: 1 out]
                          n780 = Flattened String To Variant(6:w2278, 7:w2280) -> (3:w2279:variant)  [unwired: 1 in, 1 out]
                        }
                        frame Error {
                        }
                      }
                    }
                    frame 25..27, 29, 30 {
                      # "Physical Units (0x19 .. 0x1E)"
                      n781 = Variant To Data(type=w2284, Variant=w2283) -> (data=w2285:csg, error out=w2287:errorcluster)  [unwired: 1 in]
                      n782 = case shown="No Error" w2287 {
                        tunnel: w2289 -> [w2295 _]
                        tunnel: [w2294 w2296] -> w2288
                        tunnel: w2286 -> [_ w2296]
                        tunnel: w2285 -> [w2292 _]
                        tunnel: [TRUE _] -> w2282
                        frame No Error {
                          n783 = To Variant(anything=w2292) -> (Variant=w2291:variant)
                          n784 = Variant To Flattened String(Variant=w2291) -> (data string=w2293:string)  [unwired: 1 out]
                          n785 = Flattened String To Variant(6:w2293, 7:w2295) -> (3:w2294:variant)  [unwired: 1 in, 1 out]
                        }
                        frame Error {
                        }
                      }
                    }
                  }
                }
              }
            }
            frame 29 {
              # "CDB PhysUnit (0x1D)"
              n786 = Variant To Flattened String(Variant=w2303) -> (1:w2307:i16[])  [unwired: 1 out]
              n787 = call "TypeDescriptor_GetType.vi"("type descriptor"=w2307) -> ("Type"=w2298:u8)  [unwired: 9 in, 1 out]
              n788 = Equal?(x=w2299, y=w2298) -> (x = y?=w2301:bool)
              n789 = Compound Arithmetic op=OR(w2301, invert w2297) -> (w2300:bool)
              n790 = case shown="True" w2300 {
                tunnel: w2306 -> [w2308 w2315]
                tunnel: [w2308 w2314] -> w2305
                tunnel: w2304 -> [_ w2313]
                tunnel: w2298 -> [_ w2312]
                tunnel: w2303 -> [_ w2310]
                tunnel: [_ w2309] -> w2302
                frame False {
                }
                frame True {
                  w2311 = cdb 0.0+0.0i  # CDB
                  n791 = case shown="19..1C, 1E" w2312 {
                    tunnel: w2315 -> [w2316 _ w2326 w2341 w2356]
                    tunnel: [w2316 w2317 w2328 w2343 w2358] -> w2314
                    tunnel: w2313 -> [_ w2319 w2329 w2344 w2359]
                    tunnel: w2311 -> [_ _ w2324 w2339 w2354]
                    tunnel: w2310 -> [_ w2321 w2323 w2338 w2353]
                    tunnel: [_ TRUE w2322 w2337 w2352] -> w2309
                    frame Default {
                      # "INCOMPATIBLE DATATYPES"
                    }
                    frame 29 {
                      # "CDB PhysUnit (0x1D)"
                      n792 = Variant To Flattened String(Variant=w2321) -> (data string=w2320:string)  [unwired: 1 out]
                      n793 = Flattened String To Variant(6:w2320, 7:w2319) -> (3:w2317:variant)  [unwired: 1 in, 1 out]
                    }
                    frame 1..8 {
                      # "I8, I16, I32, I64, U8, U16, U32, U64"
                      n794 = Variant To Data(type=w2324, Variant=w2323) -> (data=w2325:cdb, error out=w2327:errorcluster)  [unwired: 1 in]
                      n795 = case shown="No Error" w2327 {
                        tunnel: w2329 -> [w2335 _]
                        tunnel: [w2334 w2336] -> w2328
                        tunnel: w2326 -> [_ w2336]
                        tunnel: w2325 -> [w2332 _]
                        tunnel: [TRUE _] -> w2322
                        frame No Error {
                          n796 = To Variant(anything=w2332) -> (Variant=w2331:variant)
                          n797 = Variant To Flattened String(Variant=w2331) -> (data string=w2333:string)  [unwired: 1 out]
                          n798 = Flattened String To Variant(6:w2333, 7:w2335) -> (3:w2334:variant)  [unwired: 1 in, 1 out]
                        }
                        frame Error {
                        }
                      }
                    }
                    frame 9..14 {
                      # "SGL, DBL, EXT, CSG, CDB (0x09 .. 0x0E)"
                      n799 = Variant To Data(type=w2339, Variant=w2338) -> (data=w2340:cdb, error out=w2342:errorcluster)  [unwired: 1 in]
                      n800 = case shown="No Error" w2342 {
                        tunnel: w2344 -> [w2350 _]
                        tunnel: [w2349 w2351] -> w2343
                        tunnel: w2341 -> [_ w2351]
                        tunnel: w2340 -> [w2347 _]
                        tunnel: [TRUE _] -> w2337
                        frame No Error {
                          n801 = To Variant(anything=w2347) -> (Variant=w2346:variant)
                          n802 = Variant To Flattened String(Variant=w2346) -> (data string=w2348:string)  [unwired: 1 out]
                          n803 = Flattened String To Variant(6:w2348, 7:w2350) -> (3:w2349:variant)  [unwired: 1 in, 1 out]
                        }
                        frame Error {
                        }
                      }
                    }
                    frame 25..28, 30 {
                      # "Physical Units (0x19 .. 0x1E)"
                      n804 = Variant To Data(type=w2354, Variant=w2353) -> (data=w2355:cdb, error out=w2357:errorcluster)  [unwired: 1 in]
                      n805 = case shown="No Error" w2357 {
                        tunnel: w2359 -> [w2365 _]
                        tunnel: [w2364 w2366] -> w2358
                        tunnel: w2356 -> [_ w2366]
                        tunnel: w2355 -> [w2362 _]
                        tunnel: [TRUE _] -> w2352
                        frame No Error {
                          n806 = To Variant(anything=w2362) -> (Variant=w2361:variant)
                          n807 = Variant To Flattened String(Variant=w2361) -> (data string=w2363:string)  [unwired: 1 out]
                          n808 = Flattened String To Variant(6:w2363, 7:w2365) -> (3:w2364:variant)  [unwired: 1 in, 1 out]
                        }
                        frame Error {
                        }
                      }
                    }
                  }
                }
              }
            }
            frame 30 {
              # "CXT PhysUnit (0x1E)"
              n809 = Variant To Flattened String(Variant=w2373) -> (1:w2377:i16[])  [unwired: 1 out]
              n810 = call "TypeDescriptor_GetType.vi"("type descriptor"=w2377) -> ("Type"=w2367:u8)  [unwired: 9 in, 1 out]
              n811 = Equal?(x=w2368, y=w2367) -> (x = y?=w2371:bool)
              n812 = Compound Arithmetic op=OR(w2371, invert w2369) -> (w2370:bool)
              n813 = case shown="True" w2370 {
                tunnel: w2376 -> [w2378 w2385]
                tunnel: [w2378 w2384] -> w2375
                tunnel: w2374 -> [_ w2383]
                tunnel: w2367 -> [_ w2382]
                tunnel: w2373 -> [_ w2380]
                tunnel: [_ w2379] -> w2372
                frame False {
                }
                frame True {
                  w2381 = cxt 0.0+0.0i  # CXT
                  n814 = case shown="1..8" w2382 {
                    tunnel: w2385 -> [w2386 _ w2396 w2411 w2426]
                    tunnel: [w2386 w2388 w2398 w2413 w2428] -> w2384
                    tunnel: w2383 -> [_ w2389 w2399 w2414 w2429]
                    tunnel: w2381 -> [_ _ w2394 w2409 w2424]
                    tunnel: w2380 -> [_ w2391 w2393 w2408 w2423]
                    tunnel: [_ TRUE w2392 w2407 w2422] -> w2379
                    frame Default {
                      # "INCOMPATIBLE DATATYPES"
                    }
                    frame 30 {
                      # "CXT PhysUnit (0x1E)"
                      n815 = Variant To Flattened String(Variant=w2391) -> (data string=w2390:string)  [unwired: 1 out]
                      n816 = Flattened String To Variant(6:w2390, 7:w2389) -> (3:w2388:variant)  [unwired: 1 in, 1 out]
                    }
                    frame 1..8 {
                      # "I8, I16, I32, I64, U8, U16, U32, U64"
                      n817 = Variant To Data(type=w2394, Variant=w2393) -> (data=w2395:cxt, error out=w2397:errorcluster)  [unwired: 1 in]
                      n818 = case shown="No Error" w2397 {
                        tunnel: w2399 -> [w2405 _]
                        tunnel: [w2404 w2406] -> w2398
                        tunnel: w2396 -> [_ w2406]
                        tunnel: w2395 -> [w2402 _]
                        tunnel: [TRUE _] -> w2392
                        frame No Error {
                          n819 = To Variant(anything=w2402) -> (Variant=w2401:variant)
                          n820 = Variant To Flattened String(Variant=w2401) -> (data string=w2403:string)  [unwired: 1 out]
                          n821 = Flattened String To Variant(6:w2403, 7:w2405) -> (3:w2404:variant)  [unwired: 1 in, 1 out]
                        }
                        frame Error {
                        }
                      }
                    }
                    frame 9..14 {
                      # "SGL, DBL, EXT, CSG, CDB (0x09 .. 0x0E)"
                      n822 = Variant To Data(type=w2409, Variant=w2408) -> (data=w2410:cxt, error out=w2412:errorcluster)  [unwired: 1 in]
                      n823 = case shown="No Error" w2412 {
                        tunnel: w2414 -> [w2420 _]
                        tunnel: [w2419 w2421] -> w2413
                        tunnel: w2411 -> [_ w2421]
                        tunnel: w2410 -> [w2417 _]
                        tunnel: [TRUE _] -> w2407
                        frame No Error {
                          n824 = To Variant(anything=w2417) -> (Variant=w2416:variant)
                          n825 = Variant To Flattened String(Variant=w2416) -> (data string=w2418:string)  [unwired: 1 out]
                          n826 = Flattened String To Variant(6:w2418, 7:w2420) -> (3:w2419:variant)  [unwired: 1 in, 1 out]
                        }
                        frame Error {
                        }
                      }
                    }
                    frame 25..29 {
                      # "Physical Units (0x19 .. 0x1E)"
                      n827 = Variant To Data(type=w2424, Variant=w2423) -> (data=w2425:cxt, error out=w2427:errorcluster)  [unwired: 1 in]
                      n828 = case shown="No Error" w2427 {
                        tunnel: w2429 -> [w2435 _]
                        tunnel: [w2434 w2436] -> w2428
                        tunnel: w2426 -> [_ w2436]
                        tunnel: w2425 -> [w2432 _]
                        tunnel: [TRUE _] -> w2422
                        frame No Error {
                          n829 = To Variant(anything=w2432) -> (Variant=w2431:variant)
                          n830 = Variant To Flattened String(Variant=w2431) -> (data string=w2433:string)  [unwired: 1 out]
                          n831 = Flattened String To Variant(6:w2433, 7:w2435) -> (3:w2434:variant)  [unwired: 1 in, 1 out]
                        }
                        frame Error {
                        }
                      }
                    }
                  }
                }
              }
            }
            frame 33 {
              # "Boolean (0x21)"
              n832 = Variant To Flattened String(Variant=w2443) -> (1:w2447:i16[])  [unwired: 1 out]
              n833 = call "TypeDescriptor_GetType.vi"("type descriptor"=w2447) -> ("Type"=w2437:u8)  [unwired: 9 in, 1 out]
              n834 = Equal?(x=w2438, y=w2437) -> (x = y?=w2441:bool)
              n835 = Compound Arithmetic op=OR(w2441, invert w2439) -> (w2440:bool)
              n836 = case shown="True" w2440 {
                tunnel: w2446 -> [w2448 w2454]
                tunnel: [w2448 w2453] -> w2445
                tunnel: w2444 -> [_ w2452]
                tunnel: w2437 -> [_ w2451]
                tunnel: w2443 -> [_ w2450]
                tunnel: [_ w2449] -> w2442
                frame False {
                }
                frame True {
                  n837 = case shown="30" w2451 {
                    tunnel: w2454 -> [w2455 _ _ w2475]
                    tunnel: [w2455 w2465 w2470 w2477] -> w2453
                    tunnel: w2452 -> [_ w2466 w2471 w2479]
                    tunnel: w2450 -> [_ w2464 w2468 w2473]
                    tunnel: [_ TRUE TRUE w2472] -> w2449
                    frame Default {
                      # "INCOMPATIBLE DATATYPES"
                    }
                    frame 1..8 {
                      # "I8, I16, I32, I64, U8, U16, U32"
                      n838 = Variant To Flattened String(Variant=w2464) -> (data string=w2463:string)  [unwired: 1 out]
                      n839 = String To Byte Array(string=w2463) -> (unsigned byte array=w2461:u8[])
                      n840 = Not Equal To 0?(x=w2461) -> (x != 0?=w2462:bool[])
                      n841 = Or Array Elements(Boolean array=w2462) -> (logical OR=w2460:bool)
                      n842 = Select(t="\u0001" ("string"), s=w2460, f="\u0000" ("string")) -> (s? t:f=w2457:string)
                      n843 = Flattened String To Variant(6:w2457, 7:w2466) -> (3:w2465:variant)  [unwired: 1 in, 1 out]
                    }
                    frame 33 {
                      # "Boolean (0x21)"
                      n844 = Variant To Flattened String(Variant=w2468) -> (data string=w2469:string)  [unwired: 1 out]
                      n845 = Flattened String To Variant(6:w2469, 7:w2471) -> (3:w2470:variant)  [unwired: 1 in, 1 out]
                    }
                    frame 48 {
                      # "STRING (0x30)"
                      n846 = Variant To Data(type="", Variant=w2473) -> (data=w2474:string, error out=w2476:errorcluster)  [unwired: 1 in]
                      n847 = case shown="No Error" w2476 {
                        tunnel: w2479 -> [w2481 _]
                        tunnel: [w2482 w2493] -> w2477
                        tunnel: w2475 -> [w2483 w2493]
                        tunnel: w2474 -> [w2485 _]
                        tunnel: [TRUE _] -> w2472
                        frame No Error {
                          n848 = To Lower Case(string=w2485) -> (all lower case string=w2484:string)
                          n849 = case shown="\"true\"" w2484 {
                            tunnel: w2483 -> [w2486 _ _]
                            tunnel: [w2486 w2487 w2490] -> w2482
                            tunnel: w2481 -> [_ w2489 w2492]
                            frame Default {
                            }
                            frame "true" {
                              n850 = Flattened String To Variant(6:"\u0001" ("data string"), 7:w2489) -> (3:w2487:variant)  [unwired: 1 in, 1 out]
                            }
                            frame "false" {
                              n851 = Flattened String To Variant(6:"\u0000" ("data string"), 7:w2492) -> (3:w2490:variant)  [unwired: 1 in, 1 out]
                            }
                          }
                        }
                        frame Error {
                        }
                      }
                    }
                  }
                }
              }
            }
            frame 48 {
              # "STRING (0x30)"
              n852 = Variant To Flattened String(Variant=w2503) -> (data string=w2502:string, 1:w2501:i16[])
              n853 = call "TypeDescriptor_GetType.vi"("type descriptor"=w2501) -> ("Type"=w2496:u8, "type descriptor dup"=w2504:i16[])  [unwired: 9 in]
              n854 = Equal?(x=w2497, y=w2496) -> (x = y?=w2499:bool)
              n855 = Compound Arithmetic op=OR(w2499, invert w2495) -> (w2498:bool)
              n856 = case shown="True" w2498 {
                tunnel: w2507 -> [w2508 w2517]
                tunnel: [w2508 w2516] -> w2506
                tunnel: w2505 -> [_ w2515]
                tunnel: w2496 -> [_ w2514]
                tunnel: w2504 -> [_ w2513]
                tunnel: w2503 -> [_ w2512]
                tunnel: w2502 -> [_ w2511]
                tunnel: [_ w2510] -> w2500
                tunnel: w2494 -> [_ w2509]
                frame False {
                }
                frame True {
                  n857 = case shown="30" w2514 {
                    tunnel: w2511 -> [_ w2522 _ _ _ _ _ _ _ _ _ _ _ _ _ _ _ _ w2799]
                    tunnel: w2517 -> [w2518 _ w2526 w2542 w2559 w2575 w2591 w2607 w2623 w2639 w2655 w2671 w2688 w2706 w2724 w2742 w2760 w2778 _]
                    tunnel: [w2518 w2521 w2528 w2544 w2561 w2577 w2593 w2609 w2625 w2641 w2657 w2673 w2690 w2708 w2726 w2744 w2762 w2780 w2800] -> w2516
                    tunnel: w2515 -> [_ w2520 w2530 w2546 w2562 w2578 w2594 w2610 w2626 w2642 w2658 w2674 w2691 w2709 w2727 w2745 w2763 w2781 w2801]
                    tunnel: w2513 -> [_ _ _ _ _ _ _ _ _ _ _ _ _ _ _ _ _ _ w2795]
                    tunnel: w2512 -> [_ _ w2524 w2540 w2556 w2572 w2588 w2604 w2620 w2636 w2652 w2668 w2685 w2703 w2721 w2739 w2757 w2775 _]
                    tunnel: [_ TRUE w2523 w2539 w2555 w2571 w2587 w2603 w2619 w2635 w2651 w2667 w2684 w2702 w2720 w2738 w2756 w2774 TRUE] -> w2510
                    tunnel: w2509 -> [_ _ _ _ _ _ _ _ _ _ _ _ w2683 w2701 w2719 w2737 w2755 w2773 _]
                    frame Default {
                      # "INCOMPATIBLE DATATYPES"
                    }
                    frame 48 {
                      # "STRING (0x30)"
                      n858 = Flattened String To Variant(6:w2522, 7:w2520) -> (3:w2521:variant)  [unwired: 1 in, 1 out]
                    }
                    frame 50 {
                      # "PATH (0x32)"
                      n859 = Variant To Data(type=path "", Variant=w2524) -> (data=w2525:path, error out=w2527:errorcluster)  [unwired: 1 in]
                      n860 = case shown="No Error" w2527 {
                        tunnel: w2530 -> [w2537 _]
                        tunnel: [w2536 w2538] -> w2528
                        tunnel: w2526 -> [_ w2538]
                        tunnel: w2525 -> [w2533 _]
                        tunnel: [TRUE _] -> w2523
                        frame No Error {
                          n861 = Path To String(path=w2533) -> (string=w2535:string)
                          n862 = To Variant(anything=w2535) -> (Variant=w2534:variant)
                          n863 = Variant To Flattened String(Variant=w2534) -> (data string=w2532:string)  [unwired: 1 out]
                          n864 = Flattened String To Variant(6:w2532, 7:w2537) -> (3:w2536:variant)  [unwired: 1 in, 1 out]
                        }
                        frame Error {
                        }
                      }
                    }
                    frame 33 {
                      # "BOOLEAN (0x21)"
                      n865 = Variant To Data(type=FALSE, Variant=w2540) -> (data=w2541:bool, error out=w2543:errorcluster)  [unwired: 1 in]
                      n866 = case shown="No Error" w2543 {
                        tunnel: w2546 -> [w2553 _]
                        tunnel: [w2552 w2554] -> w2544
                        tunnel: w2542 -> [_ w2554]
                        tunnel: w2541 -> [w2549 _]
                        tunnel: [TRUE _] -> w2539
                        frame No Error {
                          n867 = Format Into String(w2549) -> (resulting string=w2548:string)  [unwired: 3 in, 1 out]
                          n868 = To Variant(anything=w2548) -> (Variant=w2551:variant)
                          n869 = Variant To Flattened String(Variant=w2551) -> (data string=w2550:string)  [unwired: 1 out]
                          n870 = Flattened String To Variant(6:w2550, 7:w2553) -> (3:w2552:variant)  [unwired: 1 in, 1 out]
                        }
                        frame Error {
                        }
                      }
                    }
                    frame 1 {
                      # "I8 (0x01)"
                      n871 = Variant To Data(type=i8 0, Variant=w2556) -> (data=w2558:i8, error out=w2560:errorcluster)  [unwired: 1 in]
                      n872 = case shown="No Error" w2560 {
                        tunnel: w2562 -> [w2569 _]
                        tunnel: [w2568 w2570] -> w2561
                        tunnel: w2559 -> [_ w2570]
                        tunnel: w2558 -> [w2565 _]
                        tunnel: [TRUE _] -> w2555
                        frame No Error {
                          n873 = Format Into String(w2565) -> (resulting string=w2564:string)  [unwired: 3 in, 1 out]
                          n874 = To Variant(anything=w2564) -> (Variant=w2567:variant)
                          n875 = Variant To Flattened String(Variant=w2567) -> (data string=w2566:string)  [unwired: 1 out]
                          n876 = Flattened String To Variant(6:w2566, 7:w2569) -> (3:w2568:variant)  [unwired: 1 in, 1 out]
                        }
                        frame Error {
                        }
                      }
                    }
                    frame 2 {
                      # "I16 (0x02)"
                      n877 = Variant To Data(type=i16 0, Variant=w2572) -> (data=w2574:i16, error out=w2576:errorcluster)  [unwired: 1 in]
                      n878 = case shown="No Error" w2576 {
                        tunnel: w2578 -> [w2585 _]
                        tunnel: [w2584 w2586] -> w2577
                        tunnel: w2575 -> [_ w2586]
                        tunnel: w2574 -> [w2581 _]
                        tunnel: [TRUE _] -> w2571
                        frame No Error {
                          n879 = Format Into String(w2581) -> (resulting string=w2580:string)  [unwired: 3 in, 1 out]
                          n880 = To Variant(anything=w2580) -> (Variant=w2583:variant)
                          n881 = Variant To Flattened String(Variant=w2583) -> (data string=w2582:string)  [unwired: 1 out]
                          n882 = Flattened String To Variant(6:w2582, 7:w2585) -> (3:w2584:variant)  [unwired: 1 in, 1 out]
                        }
                        frame Error {
                        }
                      }
                    }
                    frame 3 {
                      # "I32 (0x03)"
                      n883 = Variant To Data(type=0, Variant=w2588) -> (data=w2590:i32, error out=w2592:errorcluster)  [unwired: 1 in]
                      n884 = case shown="No Error" w2592 {
                        tunnel: w2594 -> [w2601 _]
                        tunnel: [w2600 w2602] -> w2593
                        tunnel: w2591 -> [_ w2602]
                        tunnel: w2590 -> [w2597 _]
                        tunnel: [TRUE _] -> w2587
                        frame No Error {
                          n885 = Format Into String(w2597) -> (resulting string=w2596:string)  [unwired: 3 in, 1 out]
                          n886 = To Variant(anything=w2596) -> (Variant=w2599:variant)
                          n887 = Variant To Flattened String(Variant=w2599) -> (data string=w2598:string)  [unwired: 1 out]
                          n888 = Flattened String To Variant(6:w2598, 7:w2601) -> (3:w2600:variant)  [unwired: 1 in, 1 out]
                        }
                        frame Error {
                        }
                      }
                    }
                    frame 4 {
                      # "I64 (0x04)"
                      n889 = Variant To Data(type=i64 0, Variant=w2604) -> (data=w2606:i64, error out=w2608:errorcluster)  [unwired: 1 in]
                      n890 = case shown="No Error" w2608 {
                        tunnel: w2610 -> [w2617 _]
                        tunnel: [w2616 w2618] -> w2609
                        tunnel: w2607 -> [_ w2618]
                        tunnel: w2606 -> [w2613 _]
                        tunnel: [TRUE _] -> w2603
                        frame No Error {
                          n891 = Format Into String(w2613) -> (resulting string=w2612:string)  [unwired: 3 in, 1 out]
                          n892 = To Variant(anything=w2612) -> (Variant=w2615:variant)
                          n893 = Variant To Flattened String(Variant=w2615) -> (data string=w2614:string)  [unwired: 1 out]
                          n894 = Flattened String To Variant(6:w2614, 7:w2617) -> (3:w2616:variant)  [unwired: 1 in, 1 out]
                        }
                        frame Error {
                        }
                      }
                    }
                    frame 5 {
                      # "U8 (0x05)"
                      n895 = Variant To Data(type=u8 0, Variant=w2620) -> (data=w2622:u8, error out=w2624:errorcluster)  [unwired: 1 in]
                      n896 = case shown="No Error" w2624 {
                        tunnel: w2626 -> [w2633 _]
                        tunnel: [w2632 w2634] -> w2625
                        tunnel: w2623 -> [_ w2634]
                        tunnel: w2622 -> [w2629 _]
                        tunnel: [TRUE _] -> w2619
                        frame No Error {
                          n897 = Format Into String(w2629) -> (resulting string=w2628:string)  [unwired: 3 in, 1 out]
                          n898 = To Variant(anything=w2628) -> (Variant=w2631:variant)
                          n899 = Variant To Flattened String(Variant=w2631) -> (data string=w2630:string)  [unwired: 1 out]
                          n900 = Flattened String To Variant(6:w2630, 7:w2633) -> (3:w2632:variant)  [unwired: 1 in, 1 out]
                        }
                        frame Error {
                        }
                      }
                    }
                    frame 6 {
                      # "U16 (0x06)"
                      n901 = Variant To Data(type=u16 0, Variant=w2636) -> (data=w2638:u16, error out=w2640:errorcluster)  [unwired: 1 in]
                      n902 = case shown="No Error" w2640 {
                        tunnel: w2642 -> [w2649 _]
                        tunnel: [w2648 w2650] -> w2641
                        tunnel: w2639 -> [_ w2650]
                        tunnel: w2638 -> [w2645 _]
                        tunnel: [TRUE _] -> w2635
                        frame No Error {
                          n903 = Format Into String(w2645) -> (resulting string=w2644:string)  [unwired: 3 in, 1 out]
                          n904 = To Variant(anything=w2644) -> (Variant=w2647:variant)
                          n905 = Variant To Flattened String(Variant=w2647) -> (data string=w2646:string)  [unwired: 1 out]
                          n906 = Flattened String To Variant(6:w2646, 7:w2649) -> (3:w2648:variant)  [unwired: 1 in, 1 out]
                        }
                        frame Error {
                        }
                      }
                    }
                    frame 7 {
                      # "U32 (0x07)"
                      n907 = Variant To Data(type=u32 0, Variant=w2652) -> (data=w2654:u32, error out=w2656:errorcluster)  [unwired: 1 in]
                      n908 = case shown="No Error" w2656 {
                        tunnel: w2658 -> [w2665 _]
                        tunnel: [w2664 w2666] -> w2657
                        tunnel: w2655 -> [_ w2666]
                        tunnel: w2654 -> [w2661 _]
                        tunnel: [TRUE _] -> w2651
                        frame No Error {
                          n909 = Format Into String(w2661) -> (resulting string=w2660:string)  [unwired: 3 in, 1 out]
                          n910 = To Variant(anything=w2660) -> (Variant=w2663:variant)
                          n911 = Variant To Flattened String(Variant=w2663) -> (data string=w2662:string)  [unwired: 1 out]
                          n912 = Flattened String To Variant(6:w2662, 7:w2665) -> (3:w2664:variant)  [unwired: 1 in, 1 out]
                        }
                        frame Error {
                        }
                      }
                    }
                    frame 8 {
                      # "U64 (0x08)"
                      n913 = Variant To Data(type=u64 0, Variant=w2668) -> (data=w2670:u64, error out=w2672:errorcluster)  [unwired: 1 in]
                      n914 = case shown="No Error" w2672 {
                        tunnel: w2674 -> [w2681 _]
                        tunnel: [w2680 w2682] -> w2673
                        tunnel: w2671 -> [_ w2682]
                        tunnel: w2670 -> [w2677 _]
                        tunnel: [TRUE _] -> w2667
                        frame No Error {
                          n915 = Format Into String(w2677) -> (resulting string=w2676:string)  [unwired: 3 in, 1 out]
                          n916 = To Variant(anything=w2676) -> (Variant=w2679:variant)
                          n917 = Variant To Flattened String(Variant=w2679) -> (data string=w2678:string)  [unwired: 1 out]
                          n918 = Flattened String To Variant(6:w2678, 7:w2681) -> (3:w2680:variant)  [unwired: 1 in, 1 out]
                        }
                        frame Error {
                        }
                      }
                    }
                    frame 9 {
                      # "SGL (0x09)"
                      n919 = Variant To Data(type=sgl 0.0, Variant=w2685) -> (data=w2687:sgl, error out=w2689:errorcluster)  [unwired: 1 in]
                      n920 = case shown="No Error" w2689 {
                        tunnel: w2691 -> [w2699 _]
                        tunnel: [w2698 w2700] -> w2690
                        tunnel: w2688 -> [_ w2700]
                        tunnel: w2687 -> [w2693 _]
                        tunnel: [TRUE _] -> w2684
                        tunnel: w2683 -> [w2694 _]
                        frame No Error {
                          n921 = call "SingleFloat (Scalar) to String.vi"("Use System Default Notation (F)"=w2694, "Value (Single)"=w2693) -> ("Value (String)"=w2692:string)  [unwired: 9 in]
                          n922 = To Variant(anything=w2692) -> (Variant=w2697:variant)
                          n923 = Variant To Flattened String(Variant=w2697) -> (data string=w2696:string)  [unwired: 1 out]
                          n924 = Flattened String To Variant(6:w2696, 7:w2699) -> (3:w2698:variant)  [unwired: 1 in, 1 out]
                        }
                        frame Error {
                        }
                      }
                    }
                    frame 10 {
                      # "DBL (0x0A)"
                      n925 = Variant To Data(type=0.0, Variant=w2703) -> (data=w2705:dbl, error out=w2707:errorcluster)  [unwired: 1 in]
                      n926 = case shown="No Error" w2707 {
                        tunnel: w2709 -> [w2717 _]
                        tunnel: [w2716 w2718] -> w2708
                        tunnel: w2706 -> [_ w2718]
                        tunnel: w2705 -> [w2712 _]
                        tunnel: [TRUE _] -> w2702
                        tunnel: w2701 -> [w2710 _]
                        frame No Error {
                          n927 = call "DoubleFloat (Scalar) to String.vi"("Use System Default Notation (F)"=w2710, "Value (Double)"=w2712) -> ("Value (String)"=w2711:string)  [unwired: 9 in]
                          n928 = To Variant(anything=w2711) -> (Variant=w2715:variant)
                          n929 = Variant To Flattened String(Variant=w2715) -> (data string=w2714:string)  [unwired: 1 out]
                          n930 = Flattened String To Variant(6:w2714, 7:w2717) -> (3:w2716:variant)  [unwired: 1 in, 1 out]
                        }
                        frame Error {
                        }
                      }
                    }
                    frame 11 {
                      # "EXT (0x0B)"
                      n931 = Variant To Data(type=ext 0.0, Variant=w2721) -> (data=w2723:ext, error out=w2725:errorcluster)  [unwired: 1 in]
                      n932 = case shown="No Error" w2725 {
                        tunnel: w2727 -> [w2735 _]
                        tunnel: [w2734 w2736] -> w2726
                        tunnel: w2724 -> [_ w2736]
                        tunnel: w2723 -> [w2730 _]
                        tunnel: [TRUE _] -> w2720
                        tunnel: w2719 -> [w2729 _]
                        frame No Error {
                          n933 = call "ExtendedFloat (Scalar) to String.vi"("Use System Default Notation (F)"=w2729, "Value (Extended)"=w2730) -> ("Value (String)"=w2728:string)  [unwired: 9 in]
                          n934 = To Variant(anything=w2728) -> (Variant=w2733:variant)
                          n935 = Variant To Flattened String(Variant=w2733) -> (data string=w2732:string)  [unwired: 1 out]
                          n936 = Flattened String To Variant(6:w2732, 7:w2735) -> (3:w2734:variant)  [unwired: 1 in, 1 out]
                        }
                        frame Error {
                        }
                      }
                    }
                    frame 12 {
                      # "CSG (0x0C)"
                      n937 = Variant To Data(type=csg 0.0+0.0i, Variant=w2739) -> (data=w2741:csg, error out=w2743:errorcluster)  [unwired: 1 in]
                      n938 = case shown="No Error" w2743 {
                        tunnel: w2745 -> [w2753 _]
                        tunnel: [w2752 w2754] -> w2744
                        tunnel: w2742 -> [_ w2754]
                        tunnel: w2741 -> [w2748 _]
                        tunnel: [TRUE _] -> w2738
                        tunnel: w2737 -> [w2746 _]
                        frame No Error {
                          n939 = call "SingleComplex (Scalar) to String.vi"("Use System Default Notation (F)"=w2746, "Value (CSG)"=w2748) -> ("Value (String)"=w2747:string)  [unwired: 9 in]
                          n940 = To Variant(anything=w2747) -> (Variant=w2751:variant)
                          n941 = Variant To Flattened String(Variant=w2751) -> (data string=w2750:string)  [unwired: 1 out]
                          n942 = Flattened String To Variant(6:w2750, 7:w2753) -> (3:w2752:variant)  [unwired: 1 in, 1 out]
                        }
                        frame Error {
                        }
                      }
                    }
                    frame 13 {
                      # "CDB (0x0D)"
                      n943 = Variant To Data(type=cdb 0.0+0.0i, Variant=w2757) -> (data=w2759:cdb, error out=w2761:errorcluster)  [unwired: 1 in]
                      n944 = case shown="No Error" w2761 {
                        tunnel: w2763 -> [w2771 _]
                        tunnel: [w2770 w2772] -> w2762
                        tunnel: w2760 -> [_ w2772]
                        tunnel: w2759 -> [w2766 _]
                        tunnel: [TRUE _] -> w2756
                        tunnel: w2755 -> [w2764 _]
                        frame No Error {
                          n945 = call "DoubleComplex (Scalar) to String.vi"("Use System Default Notation (F)"=w2764, "Value (CDB)"=w2766) -> ("Value (String)"=w2765:string)  [unwired: 9 in]
                          n946 = To Variant(anything=w2765) -> (Variant=w2769:variant)
                          n947 = Variant To Flattened String(Variant=w2769) -> (data string=w2768:string)  [unwired: 1 out]
                          n948 = Flattened String To Variant(6:w2768, 7:w2771) -> (3:w2770:variant)  [unwired: 1 in, 1 out]
                        }
                        frame Error {
                        }
                      }
                    }
                    frame 14 {
                      # "CXT (0x0E)"
                      n949 = Variant To Data(type=cxt 0.0+0.0i, Variant=w2775) -> (data=w2777:cxt, error out=w2779:errorcluster)  [unwired: 1 in]
                      n950 = case shown="No Error" w2779 {
                        tunnel: w2781 -> [w2789 _]
                        tunnel: [w2788 w2790] -> w2780
                        tunnel: w2778 -> [_ w2790]
                        tunnel: w2777 -> [w2784 _]
                        tunnel: [TRUE _] -> w2774
                        tunnel: w2773 -> [w2783 _]
                        frame No Error {
                          n951 = call "ExtendedComplex (Scalar) to String.vi"("Use System Default Notation (F)"=w2783, "Value (CXT)"=w2784) -> ("Value (String)"=w2782:string)  [unwired: 9 in]
                          n952 = To Variant(anything=w2782) -> (Variant=w2787:variant)
                          n953 = Variant To Flattened String(Variant=w2787) -> (data string=w2786:string)  [unwired: 1 out]
                          n954 = Flattened String To Variant(6:w2786, 7:w2789) -> (3:w2788:variant)  [unwired: 1 in, 1 out]
                        }
                        frame Error {
                        }
                      }
                    }
                    frame 21 {
                      # "EnumU8 (0x15)"
                      n955 = String To Byte Array(string=w2799) -> (unsigned byte array=w2796:u8[])
                      n956 = Index Array(array=w2796) -> (element=w2792:u8)  [unwired: 1 in]
                      n957 = call "TypeDescriptor_ListElementNames.vi"("type descriptor"=w2795) -> ("element names"=w2794:string[])  [unwired: 7 in, 3 out]
                      n958 = Index Array(array=w2794, index=w2792) -> (element=w2793:string)
                      n959 = To Variant(anything=w2793) -> (Variant=w2798:variant)
                      n960 = Variant To Flattened String(Variant=w2798) -> (data string=w2797:string)  [unwired: 1 out]
                      n961 = Flattened String To Variant(6:w2797, 7:w2801) -> (3:w2800:variant)  [unwired: 1 in, 1 out]
                    }
                  }
                }
              }
            }
            frame 50 {
              # "PATH (0x32)"
              n962 = Variant To Flattened String(Variant=w2814) -> (data string=w2813:string, 1:w2812:i16[])
              n963 = call "TypeDescriptor_GetType.vi"("type descriptor"=w2812) -> ("Type"=w2804:u8, "type descriptor dup"=w2808:i16[])  [unwired: 9 in]
              n964 = Equal?(x=w2805, y=w2804) -> (x = y?=w2806:bool)
              n965 = Compound Arithmetic op=OR(w2806, invert w2803) -> (w2802:bool)
              n966 = case shown="True" w2802 {
                tunnel: w2813 -> [_ w2822]
                tunnel: w2811 -> [w2815 w2821]
                tunnel: [w2815 w2820] -> w2810
                tunnel: w2809 -> [_ w2819]
                tunnel: w2808 -> [_ w2818]
                tunnel: [_ w2817] -> w2807
                tunnel: w2804 -> [_ w2816]
                frame False {
                }
                frame True {
                  n967 = case shown="32" w2816 {
                    tunnel: w2822 -> [_ w2827 w2836]
                    tunnel: w2821 -> [w2823 _ w2830]
                    tunnel: [w2823 w2826 w2832] -> w2820
                    tunnel: w2819 -> [_ w2825 w2838]
                    tunnel: w2818 -> [_ _ w2837]
                    tunnel: [_ TRUE w2828] -> w2817
                    frame Default {
                      # "INCOMPATIBLE DATATYPES"
                    }
                    frame 50 {
                      # "PATH (0x32)"
                      n968 = Flattened String To Variant(6:w2827, 7:w2825) -> (3:w2826:variant)  [unwired: 1 in, 1 out]
                    }
                    frame 48 {
                      # "STRING (0x30)"
                      n969 = Flattened String To Variant(6:w2836, 7:w2837) -> (0:w2833:errorcluster, 3:w2835:variant)  [unwired: 1 in]
                      n970 = Variant To Data(error in=w2833, type="", Variant=w2835) -> (data=w2829:string, error out=w2831:errorcluster)
                      n971 = case shown="No Error" w2831 {
                        tunnel: w2838 -> [w2845 _]
                        tunnel: [w2844 w2846] -> w2832
                        tunnel: w2830 -> [_ w2846]
                        tunnel: w2829 -> [w2840 _]
                        tunnel: [TRUE _] -> w2828
                        frame No Error {
                          n972 = call "String to Path.vi"("common path"=w2840) -> ("specific path"=w2839:path)  [unwired: 10 in]
                          n973 = To Variant(anything=w2839) -> (Variant=w2843:variant)
                          n974 = Variant To Flattened String(Variant=w2843) -> (data string=w2842:string)  [unwired: 1 out]
                          n975 = Flattened String To Variant(6:w2842, 7:w2845) -> (3:w2844:variant)  [unwired: 1 in, 1 out]
                        }
                        frame Error {
                        }
                      }
                    }
                  }
                }
              }
            }
            frame 64 {
              # "ARRAY (0x40)"
              n976 = Variant To Flattened String(Variant=w2854) -> (data string=w2868:string, 1:w2848:i16[])
              n977 = call "TypeDescriptor_GetArrayElementTypeDescriptor.vi"("Array Type Descriptor"=w2853) -> ("Element Type Descriptor"=w2851:i16[], "Array Type Descriptor dup"=w2852:i16[])  [unwired: 9 in]
              n978 = call "TypeDescriptor_GetArrayElementTypeDescriptor.vi"("Array Type Descriptor"=w2848) -> ("Element Type Descriptor"=w2849:i16[])  [unwired: 9 in, 1 out]
              n979 = call "TypeDescriptor_GetType.vi"("type descriptor"=w2848) -> ("Type"=w2862:u8, "type descriptor dup"=w2861:i16[])  [unwired: 9 in]
              n980 = call "TypeDescriptor_GetType.vi"("type descriptor"=w2851) -> ("Type"=w2850:u8)  [unwired: 9 in, 1 out]
              n981 = Equal?(x=w2863, y=w2862) -> (x = y?=w2864:bool)
              n982 = call "TypeDescriptor_GetType.vi"("type descriptor"=w2849) -> ("Type"=w2847:u8)  [unwired: 9 in, 1 out]
              n983 = Equal?(x=w2850, y=w2847) -> (x = y?=w2857:bool)
              n984 = call <vilib>:"TD_Compare Types.vi"("Type descriptor 2"=w2861, "Type descriptor"=w2852) -> ("Types Wireable?"=w2860:bool)  [unwired: 9 in]
              n985 = Compound Arithmetic op=OR(w2864, invert w2856) -> (w2858:bool)
              n986 = Compound Arithmetic op=OR(w2857, invert w2856) -> (w2855:bool)
              n987 = Compound Arithmetic op=AND(w2860, w2858, w2855) -> (w2859:bool)
              n988 = case shown="False" w2859 {
                tunnel: w2868 -> [w2875 _]
                tunnel: w2867 -> [w2873 w2878]
                tunnel: [w2871 w2881] -> w2866
                tunnel: w2852 -> [w2874 _]
                tunnel: w2861 -> [_ _]
                tunnel: [w2869 w2880] -> w2865
                tunnel: w2862 -> [_ _]
                tunnel: w2854 -> [_ w2879]
                frame True {
                  n989 = Flattened String To Variant(6:w2875, 7:w2874) -> (0:w2870:errorcluster, 3:w2872:variant)  [unwired: 1 in]
                  n990 = Select(t=w2873, s=w2870, f=w2872) -> (s? t:f=w2871:variant)
                  n991 = Not(x=w2870) -> (.not. x?=w2869:bool)
                }
                frame False {
                  # "Type Casting id subtypes\nCheck if wireable"
                  n992 = Variant To Data(type=w2878, Variant=w2879) -> (data=w2877:variant, error out=w2876:errorcluster)  [unwired: 1 in]
                  n993 = Select(t=w2878, s=w2876, f=w2877) -> (s? t:f=w2881:variant)
                  n994 = Not(x=w2876) -> (.not. x?=w2880:bool)
                }
              }
            }
            frame 80 {
              # "CLUSTER (0x50)"
              n995 = call "Variant_ExtractClusterElements.vi"("Cluster"=w2892) -> ("name"=w2882:string, "Elements"=w2888:variant[])  [unwired: 8 in, 1 out]
              n996 = for {
                tunnel: w2888 -> [w2899] mode=indexing
                tunnel: [w2902] -> w2887 mode=indexing
                shift-right: [w2901] -> w2883
                shift-left: variant ("variant") -> [w2900]
                n997 = call "Variant_GetName.vi"("Variant"=w2899) -> ("Name"=w2898:string, "Variant dup"=w2902:variant)  [unwired: 8 in, 1 out]
                n998 = Set Variant Attribute(Variant=w2900, name=w2898, value=w2899) -> (Variant out=w2901:variant)  [unwired: 1 in, 2 out]
              }
              n999 = for {
                tunnel: w2889 -> [w2897]
                tunnel: w2887 -> [w2896] mode=indexing
                tunnel: [w2895] -> w2886 mode=indexing
                tunnel: [w2894] -> w2885 mode=indexing
                tunnel: w2883 -> [w2893]
                n1000 = call "Variant_KVP to Strict Variant.vi"("KVP"=w2893, "Strict type matching? (F)"=w2897, "Default Value"=w2896) -> ("any found?"=w2894:bool, "Value"=w2895:variant)  [unwired: 5 in, 2 out]
              }
              n1001 = call "Variant_BuildClusterFromElementArray.vi"("name"=w2882, "Elements"=w2886) -> ("Cluster"=w2890:variant)  [unwired: 9 in]
              n1002 = Or Array Elements(Boolean array=w2885) -> (logical OR=w2891:bool)
            }
            frame 112 {
              # "REFNUMS (0x70)"
              n1003 = Variant To Flattened String(Variant=w2917) -> (data string=w2916:string, 1:w2915:i16[])
              n1004 = call "TypeDescriptor_GetType.vi"("type descriptor"=w2915) -> ("Type"=w2907:u8, "type descriptor dup"=w2912:i16[])  [unwired: 9 in]
              n1005 = Equal?(x=w2903, y=w2907) -> (x = y?=w2906:bool)
              n1006 = Index Array(array=w2910, index=2) -> (element=w2909:i16)
              n1007 = Compound Arithmetic op=OR(w2906, invert w2905) -> (w2904:bool)
              n1008 = case shown="True" w2904 {
                tunnel: w2916 -> [_ w2926]
                tunnel: w2914 -> [w2918 w2925]
                tunnel: [w2918 w2924] -> w2913
                tunnel: w2912 -> [_ w2923]
                tunnel: w2910 -> [_ w2922]
                tunnel: w2909 -> [_ w2921]
                tunnel: [_ w2920] -> w2908
                tunnel: w2907 -> [_ w2919]
                frame False {
                }
                frame True {
                  n1009 = case shown="1..8" w2919 {
                    tunnel: w2926 -> [_ w2931 w2946]
                    tunnel: w2925 -> [w2927 w2929 w2943]
                    tunnel: [w2927 w2930 w2942] -> w2924
                    tunnel: w2922 -> [_ w2932 w2945]
                    tunnel: w2923 -> [_ w2935 _]
                    tunnel: w2921 -> [_ w2934 w2944]
                    tunnel: [_ _ w2941] -> w2920
                    frame Default {
                      # "INCOMPATIBLE DATATYPES"
                    }
                    frame 112 {
                      # "Check if subtype matches"
                      # "REFNUM - CHECK SUBTYPE"
                      n1010 = Index Array(array=w2935, index=2) -> (element=w2933:i16)
                      n1011 = Equal?(x=w2934, y=w2933) -> (x = y?=w2928:bool)
                      n1012 = case shown="True" w2928 {
                        tunnel: w2932 -> [_ w2940]
                        tunnel: w2931 -> [_ w2939]
                        tunnel: [w2937 w2938] -> w2930
                        tunnel: w2929 -> [w2937 _]
                        frame False {
                        }
                        frame True {
                          n1013 = Flattened String To Variant(6:w2939, 7:w2940) -> (3:w2938:variant)  [unwired: 1 in, 1 out]
                        }
                      }
                    }
                    frame 1..8 {
                      # "4-byte types or higher resolution"
                      n1014 = case shown="1, 4, 8, 9, 11, 12, 14, 15, 17, 19" w2944 {
                        tunnel: w2946 -> [_ w2957]
                        tunnel: w2945 -> [_ w2951]
                        tunnel: w2943 -> [w2947 _]
                        tunnel: [w2947 w2949] -> w2942
                        tunnel: [_ TRUE] -> w2941
                        frame Default {
                        }
                        frame 1, 4, 8, 9, 17, 18, 20, 21, 23, 25 {
                          # "Any types that have at least\n4 bytes."
                          n1015 = String To Byte Array(string=w2957) -> (unsigned byte array=w2956:u8[])
                          n1016 = Reverse 1D Array(array=w2956) -> (reversed array=w2955:u8[])
                          n1017 = Array Subset(array=w2955, length=4) -> (w2953:u8[])  [unwired: 1 in]
                          n1018 = Reverse 1D Array(array=w2953) -> (reversed array=w2952:u8[])
                          n1019 = Byte Array To String(unsigned byte array=w2952) -> (string=w2950:string)
                          n1020 = Flattened String To Variant(6:w2950, 7:w2951) -> (3:w2949:variant)  [unwired: 1 in, 1 out]
                        }
                      }
                    }
                  }
                }
              }
            }
          }
        }
      }
    }
  }
  "Value" <- w13
  "name out" <- w14
  "any found?" <- w9
  "all found?" <- w10
